vi "H2O_DIAL_NCAR_4CH_TL-15_DREW_Bristal.vi"() -> ()   [LabVIEW 2012]
uses:
  C:/Users/H2ODial/Desktop/Shared Telescope WV DIAL Code/Libraries and VIs/PowerMeterCommands.dll
  Libraries and VIs/PowerMeterCommands.dll
  <vilib>/DAQmx/write.llb/DAQmx Write (Digital 1D Bool NChan 1Samp 1Line).vi
  <vilib>/DAQmx/miscellaneous.llb/DAQmx Fill In Error Info.vi
  <vilib>/Analysis/baseanly.llb/Mean (DBL).vi
  Libraries and VIs/Scalar_Data.vi
  Libraries and VIs/Scalar_Data_3.vi
  Libraries and VIs/Scalar_Data_2.vi
  Libraries and VIs/Scalar_Data_4.vi
  <vilib>/Analysis/NI_AALBase.lvlib
  Libraries and VIs/CLDevIFace.dll
panel:
  out "FileHour":i32=23
  out "L_Count":i32=53
  out "sigma_off_total":dbl[](array[numeric])=[5.208849205039598e-25, 5.179959292841174e-25, 5.151195803046657e-25, 5.1225586514732085e-25, 5.094047747144251e-25, 5.065662992367965e-25, 5.037404282778186e-25, 5.00927150737618e-25, 4.98126454861227e-25, 4.953383282405838e-25, 4.925627578216075e-25, 4.897997299094336e-25, 4.870492301729357e-25, 4.843112436506362e-25, 4.815857547548482e-25, 4.788727472782032e-25, 4.7617220439738645e-25, 4.734841086795625e-25, 4.708084420857158e-25, 4.681451859776211e-25, 4.654943211207717e-25, 4.628558276908839e-25, 4.602296852770688e-25, 4.576158728885113e-25, 4.550143689568926e-25, 4.524251513435461e-25, 4.498481973414584e-25, 4.472834836810143e-25, 4.447309865353064e-25, 4.421906815219908e-25, 4.396625437097018e-25, 4.37146547621306e-25, 4.34642667238312e-25, 4.321508760048986e-25, 4.296711468309777e-25, 4.272034520972826e-25, 4.247477636588709e-25, 4.2230405284857445e-25, 4.1987229048037515e-25, 4.174524468541791e-25, 4.150444917575941e-25, 4.12648394471143e-25, 4.1026412377049725e-25, 4.0789164793067997e-25, 4.0553093472760867e-25, 4.03181951443899e-25, 4.008446648699997e-25, 3.9851904130758393e-25, 3.9620504657373146e-25, 3.9390264600249443e-25, 3.9161180444812275e-25, 3.8933248628938693e-25, 3.870646554304343e-25, 3.84808275304455e-25, 3.825633088767387e-25, 3.803297186471312e-25, 3.7810746665244923e-25, 3.7589651446973412e-25, 3.7369682321861625e-25, 3.715083535633669e-25, 3.693310657166629e-25, 3.6716491944131738e-25, 3.650098740528568e-25, 3.6286588842268585e-25, 3.6073292098036786e-25, 3.5861092971590296e-25, 3.5649987218229575e-25, 3.5439970549843686e-25, 3.5231038635231225e-25, 3.5023187100210476e-25, 3.481641152797277e-25, 3.461070745934916e-25, 3.440607039307999e-25, 3.420249578605639e-25, 3.3999979053628286e-25, 3.379851556985435e-25, 3.359810066782027e-25, 3.339872963989893e-25, 3.3200397738047987e-25, 3.300310017418253e-25, 3.280683212038771e-25, 3.26115887093071e-25, 3.2417365034402865e-25, 3.222415615047108e-25, 3.2031957073673925e-25, 3.1840762782254487e-25, 3.1650568216660012e-25, 3.146136828003442e-25, 3.1273157838503186e-25, 3.108593172181254e-25, 3.089968472349119e-25, 3.0714411601444525e-25, 3.053010707845716e-25, 3.0346765842511636e-25, 3.016438254736196e-25, 2.9982951813091775e-25, 2.9802468226611423e-25, 2.962292634217252e-25, 2.9444320682080165e-25, 2.9266645737124647e-25, 2.9089895967297565e-25, 2.8914065802543346e-25, 2.8739149643214034e-25, 2.8565141861062935e-25, 2.8392036799705346e-25, 2.8219828775633244e-25, 2.8048512078777227e-25, 2.78780809737001e-25, 2.7708529700069687e-25, 2.7539852473878644e-25, 2.7372043488187197e-25, 2.7205096914273037e-25, 2.703900690255505e-25, 2.6873767583778413e-25, 2.6709373069960633e-25, 2.654581745560292e-25, 2.6383094819074984e-25, 2.6221199223631447e-25, 2.606012471889248e-25, 2.589986534187844e-25, 2.574041511891159e-25, 2.5581768066557376e-25, 2.542391819344354e-25, 2.526685950182175e-25, 2.5110585988760766e-25, 2.4955091648422562e-25, 2.4800370473221455e-25, 2.4646416456015127e-25, 2.4493223591642267e-25, 2.4340785878790737e-25, 2.4189097322232995e-25, 2.4038151934512195e-25, 2.3887943737973404e-25, 2.3738466767012817e-25, 2.3589715070396223e-25, 2.3441682712794586e-25, 2.3294363777860924e-25, 2.314775236976836e-25, 2.3001842616240263e-25, 2.2856628670238404e-25, 2.2712104713105327e-25, 2.2568264956406535e-25, 2.2425103644896206e-25, 2.2282615058785225e-25, 2.214079351630966e-25, 2.199963337672995e-25, 2.185912904247297e-25, 2.171927496176536e-25, 2.1580065631915612e-25, 2.1441495601166053e-25, 2.130355947199571e-25, 2.1166251903489134e-25, 2.102956761434408e-25, 2.089350138475947e-25, 2.075804806020214e-25, 2.0623202553022427e-25, 2.0488959845615565e-25, 2.0355314992873334e-25, 2.022226312470449e-25, 2.0089799448255746e-25, 1.9957919250810776e-25, 1.982661790138582e-25, 1.9695890854004894e-25, 1.9565733648873598e-25, 1.9436141915111585e-25, 1.9307111372629915e-25, 1.91786378336177e-25, 1.9050717205270306e-25, 1.8923345490220962e-25, 1.8796518789023204e-25, 1.8670233300839603e-25, 1.8544485325389802e-25, 1.841927126361547e-25, 1.8294587618299684e-25, 1.8170430995555026e-25, 1.804679810480881e-25, 1.7923685759181059e-25, 1.7801090876455487e-25, 1.7679010477844128e-25, 1.755744168902948e-25, 1.7436381738487216e-25, 1.7315827958133316e-25, 1.7195777781516077e-25, 1.7076228743061302e-25, 1.695717847711208e-25, 1.6838624715732568e-25, 1.6720565287447544e-25, 1.6602998115080602e-25, 1.6485921213522993e-25, 1.6369332687266632e-25, 1.6253230727521978e-25, 1.6137613609636032e-25, 1.6022479689748776e-25, 1.590782740120926e-25, 1.5793655251315856e-25, 1.5679961817100763e-25, 1.5566745741448175e-25, 1.545400572901165e-25, 1.5341740540969998e-25, 1.5229948991303635e-25, 1.5118629941358614e-25, 1.5007782295195033e-25, 1.489740499358663e-25, 1.4787497009842329e-25, 1.4678057342897598e-25, 1.4569085013281887e-25, 1.446057905553199e-25, 1.4352538513748305e-25, 1.424496243524175e-25, 1.413784986430072e-25, 1.403119983632073e-25, 1.39250113710464e-25, 1.3819283467716064e-25, 1.3714015097427362e-25, 1.3609205198754617e-25, 1.3504852669717757e-25, 1.3400956363074166e-25]
  out "sigma_on_total":dbl[](array[numeric])=[1.7816460568521e-23, 1.773895265159062e-23, 1.7660996726964617e-23, 1.7582606635691275e-23, 1.7503796165295856e-23, 1.742457904707209e-23, 1.7344968950332225e-23, 1.7264979476788507e-23, 1.7184624158522698e-23, 1.7103916450731765e-23, 1.70228697290092e-23, 1.6941497285179008e-23, 1.6859812322635967e-23, 1.6777827953068067e-23, 1.6695557191750322e-23, 1.6613012955150683e-23, 1.6530208056178096e-23, 1.6447155202046477e-23, 1.6363866989483097e-23, 1.628035590346711e-23, 1.6196634312396877e-23, 1.6112714466774645e-23, 1.6028608494950746e-23, 1.594432840236233e-23, 1.585988606693132e-23, 1.5775293239155563e-23, 1.5690561537464667e-23, 1.5605702447345527e-23, 1.5520727320269274e-23, 1.5435647369440912e-23, 1.5350473670174112e-23, 1.526521715738014e-23, 1.5179888624371733e-23, 1.5094498721480932e-23, 1.5009057953909757e-23, 1.4923576681755396e-23, 1.4838065118663258e-23, 1.4752533330592848e-23, 1.4666991234694497e-23, 1.4581448599733737e-23, 1.4495915043723148e-23, 1.441040003511776e-23, 1.432491289122247e-23, 1.4239462778701797e-23, 1.4154058711623008e-23, 1.406870955384024e-23, 1.398342401692949e-23, 1.3898210660483915e-23, 1.3813077893314117e-23, 1.3728033972217122e-23, 1.3643087002505864e-23, 1.3558244939697985e-23, 1.347351558797704e-23, 1.3388906601482023e-23, 1.330442548510279e-23, 1.3220079594796904e-23, 1.3135876137976992e-23, 1.3051822174761862e-23, 1.2967924618478218e-23, 1.2884190235963751e-23, 1.2800625649506368e-23, 1.2717237336984178e-23, 1.2634031632853991e-23, 1.25510147297007e-23, 1.246819267904798e-23, 1.2385571392220061e-23, 1.2303156641504887e-23, 1.222095406160734e-23, 1.2138969151380218e-23, 1.2057207273833233e-23, 1.1975673658193516e-23, 1.1894373401234403e-23, 1.1813311468632808e-23, 1.1732492696110752e-23, 1.1651921791093205e-23, 1.1571603333900983e-23, 1.1491541779450773e-23, 1.1411741458492443e-23, 1.1332206579108972e-23, 1.1252941228701505e-23, 1.1173949374808691e-23, 1.1095234867122125e-23, 1.1016801438577447e-23, 1.0938652708072228e-23, 1.0860792179973072e-23, 1.0783223247992995e-23, 1.0705949195180339e-23, 1.0628973196199999e-23, 1.0552298318266127e-23, 1.047592752408124e-23, 1.0399863671888359e-23, 1.0324109517969625e-23, 1.0248667718463947e-23, 1.0173540830105773e-23, 1.0098731312270984e-23, 1.0024241528791567e-23, 9.950073749338678e-24, 9.876230150809686e-24, 9.802712819544858e-24, 9.729523752075448e-24, 9.656664857121758e-24, 9.584137957566187e-24, 9.511944790994246e-24, 9.44008701246367e-24, 9.368566194835521e-24, 9.297383831309462e-24, 9.226541335953e-24, 9.15604004658773e-24, 9.085881224717996e-24, 9.016066058188983e-24, 8.946595661885089e-24, 8.877471079766275e-24, 8.80869328593128e-24, 8.74026318642537e-24, 8.672181620096636e-24, 8.604449360193221e-24, 8.537067116299817e-24, 8.470035534974442e-24, 8.403355201652768e-24, 8.337026641094161e-24, 8.27105032013882e-24, 8.205426647591286e-24, 8.140155976403815e-24, 8.075238604943476e-24, 8.010674777219785e-24, 7.946464685681034e-24, 7.882608471068495e-24, 7.819106224648686e-24, 7.755957988728922e-24, 7.693163757842924e-24, 7.630723480569596e-24, 7.56863706001298e-24, 7.506904354936172e-24, 7.445525181195512e-24, 7.384499313141995e-24, 7.323826483428576e-24, 7.263506385649789e-24, 7.203538673968723e-24, 7.143922965385938e-24, 7.084658839512623e-24, 7.025745840785392e-24, 6.967183478374333e-24, 6.908971227895747e-24, 6.851108531901346e-24, 6.793594800808018e-24, 6.736429414386207e-24, 6.67961172191959e-24, 6.623141043091801e-24, 6.567016669697881e-24, 6.5112378653508866e-24, 6.455803867159162e-24, 6.400713886115458e-24, 6.345967108304617e-24, 6.2915626947315444e-24, 6.237499783446669e-24, 6.18377748907835e-24, 6.130394904244926e-24, 6.077351100139125e-24, 6.024645127233271e-24, 5.972276015715119e-24, 5.9202427766811525e-24, 5.868544402036172e-24, 5.817179866157465e-24, 5.766148125522754e-24, 5.7154481199633725e-24, 5.6650787731456875e-24, 5.6150389928060976e-24, 5.565327672180314e-24, 5.515943689491057e-24, 5.466885909347513e-24, 5.418153182700111e-24, 5.36974434796048e-24, 5.321658231169485e-24, 5.273893646284607e-24, 5.2264493962483505e-24, 5.1793242730199045e-24, 5.1325170580578076e-24, 5.086026523333733e-24, 5.0398514309077376e-24, 4.993990534244649e-24, 4.9484425777837306e-24, 4.9032062982178666e-24, 4.8582804242653355e-24, 4.813663677287351e-24, 4.7693547718840175e-24, 4.7253524158646564e-24, 4.681655310929801e-24, 4.638262152931246e-24, 4.595171632226394e-24, 4.552382434023412e-24, 4.5098932386213854e-24, 4.467702721932566e-24, 4.425809555702291e-24, 4.3842124077257986e-24, 4.3429099423396456e-24, 4.301900820527674e-24, 4.261183700301938e-24, 4.220757237070317e-24, 4.180620083546408e-24, 4.140770890465617e-24, 4.101208306569908e-24, 4.061930979032737e-24, 4.022937553353332e-24, 3.9842266741114735e-24, 3.94579698459456e-24, 3.907647127699094e-24, 3.8697757453874826e-24, 3.832181479485934e-24, 3.79486297171598e-24, 3.757818863809392e-24, 3.7210477977800845e-24, 3.684548415872136e-24, 3.648319361213695e-24, 3.612359277439583e-24, 3.576666809480403e-24, 3.54124060303094e-24, 3.506079305171125e-24]
  out "background start":u32=209
  in  "Tab Control 2":enum32{"WV ND far", "WV ND near"}(tab)
  out "Water Vapor Number Density":dbl[][](graph)=[[-3.869176758577077, 1.7276694935317216, 2.7488871422111054, 1.7014197300850586, 1.5903170185720343, 1.5423321275662938, 1.8132607286797402, 1.9740256778767107, 1.8741507349652864, 1.86470777497544, 1.8050217471405994, 1.66518518330514, 1.7222522935643614, 1.742698018284987, 1.7186667192977487, 1.76396406976016, 1.8206709341870522, 1.8804172540359552, 1.7798038295977383, 1.685641859418033, 1.7032805323016422, 1.6821483240571278, 1.7628527236349734, 1.8316160827388441, 1.7868354165982292, 1.8176435654609677, 1.8911325035020297, 1.9070639564654333, 1.6511262934763296, 1.3290513703392042, 1.261765913847659, 1.1879210634564727, 1.3181838592004227, 1.4770043973103777, 1.515246627762386, 1.4475403930811108, 1.065848464452276, 1.0853345452851404, 1.2017781570763117, 0.9102790626084151, 0.9318943803136962, 0.9732524106405078, 0.8179973089248536, 0.6079032662908113, 0.561139551967481, 0.366828467183368, 0.05249595600990845, -0.09415617998531356, -0.03868889564187686, 0.07617721364907153, 0.03962425104838462, -0.12021617725713296, 0.03637946037051569, 0.14077744142052095, 0.0245296261927154, 0.24563205234877428, 0.5539197433725966, 0.263890494465195, 0.04766355724545887, 0.09570570854419765, 0.1664575082800971, 0.06746981079040626, -0.38375673627375345, -0.3520441975802064, -0.22147709479573255, -0.2987058066521773, -0.01283079930649804, 0.27293559298756215, 0.26610575594455993, 0.00637948968643232, -0.36080028041915424, -0.7602209267225687, 0.4514801381952214, 1.1532965328629945, -0.23548265802060744, -0.25988039893494896, -0.10346486157003504, -0.9068324993519856, -1.275622846338939, -0.7873849995684254, 0.5363570467662349, 1.1750455340428092, -0.4637762421465685, -0.9826963080532389, 0.7015531311665566, 1.2530696546508981, 1.0822536008721295, 1.7170434774279757, 1.2226388206906942, -0.16161614279730033, -0.5683199941258456, -0.5177748284798833, 0.08469425738265512, -0.19130410683826007, -0.08656337463651688, -0.3423075638169604, -0.840233672330641, -0.5847959086269064, 0.3038014646272331, -0.13050495344579416, -0.1376727003604833, 3.131072497793134, 1.0729187415399541, 0.08025498921874048, -0.3838816719506945, -0.9725388459388364, -0.6672976015227235, 2.560758632555869, 2.729719175818429, 2.3215477291096027, 3.992511565505456, -3.4414781626187976, -0.46339897120913937, 5.1718139470877835, 5.339784841332441, 1.5152541194098013, 0.14047483029231167, -2.810651224807273, -2.894122973967911, -0.9646913594986185, -3.1457768234772865, 0.9532976438947683, 0.2558999676656563, -4.453408932787016, -4.666689490838906, 0.37315557538439503, 2.2772866584050298, 9.102342735433101, 14.75511277527104, 5.0407452084138225, -2.8128831706899127, 5.027850129919315, 1.8931389085909622, -2.5178123636904877, -9.123913386897096, -7.628293920055456, -7.247916135816338, -21.468900020294242, -27.22073007893985, -13.633022532482114, -6.147500862719829, -3.560625137342051, 8.50678028294044, -9.907610681399557, -0.5951038934066528, 7.40264971170572, 15.060151878437237, 11.921795085668185, 18.717702285329914, 1.661459093699086, -2.719045903890811, -1.7707613039198502, -21.905540574534093, -1.0246737433253428, 11.484928239923606, -18.946452941933938, -17.06198763650667, -8.948109634815614, -24.40872593826368, -1.1349299955140333, 17.76186196255086, 7.211953881151515, 5.768882684316489, 1.8197219317421747, -8.601060392003859, 28.569279644062227, 45.756313628626245, -3.0966253403425252, 24.64942593279667, 6.740715774414794, -13.517696399672857, -18.245119081981933, -15.538137694765226, 43.914897074779645, -11.896913533924605, -38.50542587824902, -60.431586714709645, 3.4942649258288485, -2.9978367720438235, -15.508923651730063, -32.856452935921865, 1.3021555172975168, 8.620556918106015, -36.48761227825641, 10.036727386562887, 27.44659631342583, -6.0226777499226545, 27.362796040286657, -37.45596081084036, 86.37563919610214, 63.19805672056316, 25.89420561946089, 0.556775142694816, 80.7843185510899, 4.8800300899385975, -21.298521924929055, 13.798770304785254, 41.276796377764, 25.133260462123662, -131.76792036329653, -63.33200841129719, -42.49224251142825, -17.61716602055814, -100.97764607148362, -23.093541216998897, 20.565346438983532, -21.166943213929525, -66.85855512778777, 34.9469970207709, -36.534646589901264, 127.648061869762, 113.71968873955664, 116.76977055808356, 111.55231169466157, 114.09907634429825, 88.66274623657421, 0.0, 0.0, 0.0, 0.0]]
  out "Water Vapor Number Density 2":dbl[][](graph)=[[-1.5443306097046143, 2.8522805328006084, 3.9503962044958856, 1.7990159877935195, 1.718543728389198, 1.6932470135146567, 1.7872890959132228, 1.9444655123923098, 1.9109163630014983, 1.786790355844181, 1.8203570881289517, 1.8278832324692647, 1.8215867030739905, 1.8693881519091904, 1.774018488126486, 1.7651448395397114, 2.1121219489333822, 2.2540664534955406, 2.0439110551035746, 1.9629919736185735, 1.8298595633003019, 1.7095043482327141, 1.666013989260466, 1.366285095794705, 1.4616902151466857, 2.2573272602146743, 2.697366393087735, 2.767503701368858, 2.824231151211559, 1.8391949709521593, 1.7420479845117984, 2.830301488157029, 2.1524489733156393, 2.2937880254474106, 3.9229074879334824, 3.6257729421620533, 2.4101625171808236, 2.5600619420232316, 1.2917633097948769, 1.0096849664051895, 22.61444578462568, 0.25534016546905675, -0.8899854648514799, 1.8426887683335105, -0.7431804976403255, -3.091147289752489, -3.2685662586591704, -0.6268978238054816, 9.457130422245957, 12.987376965471386, -15.76217946676521, 5.117351146699065, 9.935146112695032, 5.310666522331181, 2.8243785343871637, 2.219814346002247, -1.6824882949711026, -3.1347232460324044, 6.274677522391716, -15.294434193506227, 4.9655234368204315, -7.499211539861518, -18.986284869525754, -22.146770284669905, -15.358627756713357, -11.410536018137048, 2.694880288695569, 1.0084240385621965, -24.302059778902542, -5.424444800831853, -8.374133035691955, -3.839271193448914, -7.237647107240136, -8.381370981005263, -12.644696124542769, -14.758763725308427, -229.1767077139342, -26.690833610496536, -27.137431619530496, -35.64066674098872, -29.396651111364527, -26.79804782533207, 0.5331643103900505, 7.663673000483812, 11.575946950935077, 6.507396151064453, 209.12899102577234, 11.41629111125545, 17.293199830760145, 6.792318505705173, 32.50778308178908, 44.797851527429785, 39.153268976697944, 34.703453008989634, 30.76080492824301, 49.359391431456224, 42.446731318655694, 30.0888196357715, 8.433409642645435, 13.168323747779349, -22.073856515721904, -28.682049927165874, -44.14597625638005, -32.48394246704076, -23.003786727142135, -47.09138656023136, -47.920840441120504, -31.8982280785437, -16.04539071651972, -2.7480282517398633, 5.248156676680989, 4.922612847871278, 0.318336139544576, -0.4862458105609459, -4.179014617318633, 0.7669045218891034, 13.338663676578376, 18.57437167630363, 38.78732302419309, 26.400175395888585, 17.39277458143397, 18.272895200830188, 27.623342106489204, 20.864190489619656, 26.226824008859122, 8.996876024344196, -16.383735405016303, -23.47162210047236, -33.740458481599866, -18.105503466986512, -48.11166006948978, -42.593887413019544, -24.53098108754986, -16.94813071741411, -25.996257810862737, -0.39358969043194625, 27.123587253355726, 8.014421627535988, -6.935017542522941, 1.4770044975105434, 36.40827027087462, 36.8340413388943, 18.655014433644215, -3.3515131672034886, -21.48412539473853, -20.759894357501476, -15.862065254431439, 9.101365563103611, 20.359635034836895, 0.6709218106358483, -9.832471896842145, -16.84514663391321, -20.5476550377528, -13.656934323110177, 17.193357185961737, -3.001810086333975, -30.404097981013283, -2.8019970495102795, 11.187088633119922, 11.930034566140032, -2.3269211234070606, -17.865366856340884, -7.841326713329807, 11.502546001559406, -5.698207821198067, 8.183280425430254, 24.595245021019227, -9.239519757011584, -56.82051834132085, -25.45057389070378, 3.68551297425237, 13.924870638300932, -11.703807237602431, 1.7327637589277107, 23.617738062249668, -0.38832652817943536, -9.793160089936272, 28.29754334951125, 53.38824852184467, -9.390908410980694, -7.039011955964897, -27.352587599268645, 24.40018260217878, 23.274510436680274, -14.773755808771865, 19.203702709910885, 41.08553410088621, -25.433481617817737, -42.296254212448005, 29.341189509465494, 8.293515144836189, 12.836812085227644, 12.01172385875116, -23.51640940790944, -3.844970096464795, 24.7018027378986, -15.629344885370898, 46.841354406997496, 18.846412127663438, -8.01413384755022, 20.173550353711494, 40.332927124397294, -36.0632814643046, 42.42659273396934, 15.266963000405319, -43.789869007181714, -4.314897141425726, -71.56712981596844, -14.119956089715068, -16.016149328363884, 13.688096121679713, 15.964585047763242, 60.89547744616684, -7.0780618158529744, 21.580968070414038, 45.81592366790833, 0.0, 0.0, 0.0, 0.0]] caption="Water Vapor Number Density"
  out "RingBuffer offline near":dbl[][](array[numeric])
  out "RingBuffer aerosol near":dbl[][](array[numeric])
  in  "?":T1(tab)=enum."Raw Counts far"
  out "NRB":dbl[][](graph)=[[0.003930472506649335, 0.01856167580177092, 0.02113550600005818, 0.00020659819039981744, 0.0004794046077180199, 0.001083137552512623, 0.0021988013419836265, 0.0041092544329047785, 0.007064816134335353, 0.011356733211595298, 0.01736467597668339, 0.025026701435469114, 0.03423478045562495, 0.044428545350929015, 0.05540162610487789, 0.06689414791198389, 0.07668063258939913, 0.08177270565134998, 0.08504838543823319, 0.0941773217771789, 0.1084250899373609, 0.13043489216970022, 0.16993149950013392, 0.21569106534945648, 0.24627293298723196, 0.2621348983374077, 0.2688103499187474, 0.2614066916235843, 0.23984353258011334, 0.21654175844380677, 0.20729347010352947, 0.211907581747061, 0.21498518012682463, 0.2099940641656903, 0.20422798251892263, 0.2002067122669493, 0.1956553193564138, 0.19231512805902898, 0.18941127292353704, 0.18521706136815214, 0.18228261326514122, 0.1803780884227828, 0.17451505611111093, 0.15596012460703929, 0.12845284806608473, 0.10613962907170191, 0.08638109669200546, 0.0698685441035237, 0.0657771979941857, 0.06701804654176632, 0.06592159640438976, 0.06744466192881599, 0.07920468748072622, 0.10083415139682901, 0.13028089521913505, 0.1620054293079384, 0.18624602524852493, 0.19705712872187683, 0.18360257948359815, 0.14751724796554955, 0.1096764233903891, 0.08021880453362741, 0.061532589115181065, 0.0816391129923796, 0.1743614835528636, 0.24584930708492536, 0.1850726081138991, 0.09165193218672707, 0.05956306826808834, 0.05340250064997599, 0.04709384690987805, 0.04552738122485284, 0.10513881642759977, 0.36679509075168293, 0.6832500352597682, 0.6228452598361331, 0.2955400136740759, 0.0965288379381804, 0.04463785561721723, 0.03331459806286399, 0.0295454069625369, 0.02954898513465661, 0.03053152365445197, 0.029744787993018985, 0.028849851226770928, 0.028395038404537717, 0.02752666688359724, 0.02637978994395, 0.024532339573489555, 0.022686590876590036, 0.022164556173745933, 0.024448917357890163, 0.025449268385637276, 0.024717277849119708, 0.025034235387734093, 0.03709636240721259, 0.08373681834453293, 0.1575651146703995, 0.23175935815265392, 0.26905595638618013, 0.2660007080148815, 0.281347881372177, 0.29637751983063615, 0.2120397193829469, 0.0822185358341878, 0.02420612946619511, 0.020626164977171818, 0.02295934815454573, 0.02239546298987765, 0.020926378758381003, 0.018942726450896123, 0.02027737989045651, 0.017257308197544903, 0.01648011969227998, 0.018769849948021472, 0.01825593588795685, 0.017358907238197958, 0.018140817164234692, 0.017772892504258498, 0.017134510556994755, 0.018184511447133216, 0.015589634114438389, 0.017449874393049788, 0.021395199934042586, 0.028950512550262614, 0.04868713410644236, 0.05855925424019936, 0.056765697373354365, 0.054040949320453766, 0.03018220698627995, 0.011980903082859833, 0.013481520746379885, 0.013317721859532882, 0.012036726009435648, 0.009066141155603936, 0.010518616820675755, 0.014832016505210856, 0.014950059454567273, 0.009275637744439192, 0.009477692868505897, 0.014639857997371816, 0.015408844654833068, 0.009071008168571152, 0.006225854023779428, 0.011299265176167623, 0.012492724514216815, 0.012401612152277457, 0.010192179039525382, 0.008941655568516869, 0.00783059022139205, 0.010807654434608422, 0.014283307333364035, 0.014288825705708002, 0.010849886806011332, 0.004980035722601281, 0.005826766078719105, 0.0075934368539790275, 0.008037485025773526, 0.008886305124129305, 0.008753787211165693, 0.0056883188106616875, 0.005371602816749897, 0.008808142387202697, 0.011136376378372276, 0.004318833387582044, 0.0020970880048393737, 0.007452790671203962, 0.004158550753810091, 0.004530769527373028, 0.006894416785182974, 0.00837296741786389, 0.008085657965933137, 0.0029017041584067137, 0.006012750679637745, 0.007359146716082699, 0.008062443335548567, 0.010250086388599922, 0.004833505314473423, 0.0010466212212718276, 0.005252360150149767, 0.008100118134763674, 0.006376919009661436, 0.008745621975673537, 0.012547520645679548, 0.008878360514416051, -0.003558532177769385, -0.003931068685129671, 0.009813463187450404, 0.012245644138306774, 0.00989792059445067, 0.010224238477378817, 0.006712617893126215, -0.002666463678070868, -0.00645420474485784, -0.0031184219652592524, 0.00369116947800459, 0.0072690806727548, 0.007990187139209782, 0.008002292031103739, 0.014824575432041054, 0.014797694751457974, 0.0022899778851920263, 0.004926149957744118, 0.010253351686953951, 0.012435192336721605, 0.003082031211657591, -0.0031790134065153614, -0.0028339485571887506, -0.005707333338889842, 0.0005976659162923159, -0.000982411230437747, -0.006145669137729354, -0.00044932331870984173, 0.00428091386606607, 0.006409250601951215, 0.006428477325402283, 0.004156327474142488, 0.0, 0.0, 0.0]] caption="Water Vapor Number Density"
  out "NRB 2":dbl[][](graph)=[[0.0036371496517445994, 0.01703650318832334, 0.020633248972062875, 0.0013800426335260302, 0.003467331928749565, 0.006919838499311271, 0.011930041065111517, 0.01842671636273905, 0.025866635016207524, 0.033788053491102525, 0.042013493867585815, 0.050516184965233954, 0.059459761392953926, 0.06841915921353516, 0.07661801215634156, 0.08328622123228714, 0.08582003015959876, 0.08226852580228898, 0.0758652361797178, 0.07335427213452467, 0.07399510467073478, 0.077832413415831, 0.09074755980363364, 0.10683744208633218, 0.11379427967792226, 0.11383489707097101, 0.11213088885610459, 0.10518492418354901, 0.0920399200182776, 0.07952493986949206, 0.07523446587339368, 0.07580443903113321, 0.07507434026665262, 0.07232025663049929, 0.07040748731651326, 0.06828916338398419, 0.06567080469336894, 0.06469037970451262, 0.0644425414544769, 0.06318734377370618, 0.06063209355900223, 0.059469665719634884, 0.05748777770520413, 0.04991857127969182, 0.04039318864390559, 0.03185073389094848, 0.024176677628144835, 0.018496094801403275, 0.01776963165623099, 0.01850891772014958, 0.018428861164685752, 0.019807659791999492, 0.024041941128934815, 0.029719396461916653, 0.038809029282185416, 0.05020034200015739, 0.05660877189095595, 0.06076443427680532, 0.05511663020936872, 0.043988455546614416, 0.03331345532712681, 0.02185250713851732, 0.01577029946685516, 0.022446119886150258, 0.05594357391945572, 0.0828190885036247, 0.06050139637782499, 0.02527859256760107, 0.011594307499489899, 0.008638484256569148, 0.008864910520450759, 0.009348729824449415, 0.029540262433234078, 0.12532949022668763, 0.24340139949844283, 0.22138119398182685, 0.10007438941564159, 0.032019365617949685, 0.012390245530805056, 0.004528276018205554, 0.003275796002140223, 0.004952505987005521, 0.0069991223807995846, 0.0018426755657387614, 0.0013916137984439276, 0.003536719849559254, 0.004936369466053812, 0.00805833393141099, 0.003530237474819559, -4.1280975248141e-05, -0.0031128209847992912, -0.0019544928287063244, 0.003915493745935216, 0.001173942428925932, -0.006350329178034576, 0.0006899543668811116, 0.031108497607104286, 0.06399430457460561, 0.09217643099719275, 0.10360682795834994, 0.0988357573984754, 0.10485562014796758, 0.10315263871478404, 0.06938872580477172, 0.018961832555909063, -0.0035917489198442724, -0.002744383733131294, 0.0021338721511815306, 0.01415905229358902, 0.010655942951313698, 0.002254067110314441, 0.007354262975912472, 0.0036375737229856144, 0.0005047422524058872, 0.0035815414407817767, -0.0005178767966525964, -0.009391539564641088, -0.00946712496314058, 0.005303356363483911, 0.0020270499020427057, -0.0035738458960578264, -0.001396774601107916, -0.007521451653945964, -0.00930600236629641, 0.001883706461300565, 0.018403847478748257, 0.021007462570787113, 0.019640636355698602, 0.026383250232868284, 0.006611280584980362, -0.012798886930294198, 0.0024680408939121525, 0.008116803607827227, 0.0011549383540302525, -0.007827595884048846, -0.00495364879429496, 0.01939889749061799, 0.022444448653450716, 0.0021764895193934737, -0.0030793419371683266, 0.00866841075399524, -0.0005811484210449667, -0.01605964672983413, -0.008942504556462935, 0.005416782653565494, 0.001595818932773196, -0.00407852130382172, -0.0058663885807870245, -0.012305286929516712, -0.005294513758219532, 0.009801323745479663, 0.008449529836930333, -0.0026493162817863725, -0.008873147676594886, -0.011268625608977586, -0.002027183814169297, -0.0025514075997150856, 0.0025708727112535097, 0.021153088711398944, 0.013568986385791905, -0.017031895122065075, 0.004432240632801877, 0.0032964694542234113, -0.00902308178105749, 0.0019664276294757313, -0.017791447391965472, -0.0105814723327946, 0.02086255624836402, 0.015289014861491292, -0.011879223092562698, -0.013072802023074051, -0.008053240428419393, 0.0035555595583932225, 0.011444910625672548, 0.025812896369300224, 0.024584415737324762, -0.0014810339765029656, -0.0013586140933279985, -0.0012331517866784963, -0.0022149323139001313, 0.01002370286931542, 0.00163575012314951, -0.004525777742427229, -0.017129143916830177, -0.004835752924455243, 0.01709079326051516, 0.014110065578375252, -0.003813723821663823, 0.0024231432824741634, 0.004732768871162198, 0.008725613632898954, 0.04681544982055149, 0.05126517573045018, 0.008208163504057038, 0.004818076358944868, 0.044330213093104746, 0.019581290580246866, -0.0010954537471730096, 0.05196173543341118, 0.07206495557244628, 0.05212384819727444, 0.05282307279007492, 0.060119382877862344, 0.04502404489351928, 0.02899591798938946, 0.04870805826786507, 0.049069136303961605, 0.05346037076736777, 0.014785011813988698, -0.010377246966110278, 0.0077928132458859115, -0.024042200815203283, -0.03718525117731811, -0.03439665496604084, -0.00445979226507979, 0.0441218508899156, 0.029220984290769872, 0.0, 0.0, 0.0]] caption="Water Vapor Number Density"
  out "raw counts":dbl[][](graph)=[[17706.9, 19006.9, 23324.9, 69.9, 98.9, 165.9, 240.9, 316.9, 472.9, 547.9, 776.9, 879.9, 1050.9, 1300.9, 1491.9, 1492.9, 1595.9, 1497.9, 1327.9, 1459.9, 1423.9, 1517.9, 1909.9, 2153.9, 2285.9, 2360.9, 2225.9, 1991.9, 1677.9, 1479.9, 1256.9, 1211.9, 1215.9, 1123.9, 978.9, 900.9, 804.9, 743.9, 716.9, 664.9, 669.9, 611.9, 598.9, 582.9, 408.9, 338.9, 274.9, 233.9, 150.9, 166.9, 160.9, 130.9, 174.9, 184.9, 216.9, 306.9, 304.9, 351.9, 314.9, 279.9, 202.9, 144.9, 94.9, 95.9, 154.9, 355.9, 376.9, 159.9, 69.9, 60.900000000000006, 58.900000000000006, 19.900000000000006, 40.900000000000006, 137.9, 568.9, 827.9, 528.9, 140.9, 38.900000000000006, 20.900000000000006, 31.900000000000006, 43.900000000000006, 38.900000000000006, 28.900000000000006, 39.900000000000006, 26.900000000000006, 6.900000000000006, 13.900000000000006, 29.900000000000006, 20.900000000000006, 14.900000000000006, 2.9000000000000057, 5.900000000000006, 30.900000000000006, 7.900000000000006, 17.900000000000006, 18.900000000000006, 97.9, 97.9, 139.9, 147.9, 122.9, 137.9, 176.9, 65.9, 27.900000000000006, 13.900000000000006, 48.900000000000006, 14.900000000000006, 14.900000000000006, 12.900000000000006, 12.900000000000006, 2.9000000000000057, 1.9000000000000057, -8.099999999999994, 15.900000000000006, 22.900000000000006, 30.900000000000006, 1.9000000000000057, 19.900000000000006, 12.900000000000006, -6.099999999999994, 21.900000000000006, 0.9000000000000057, 3.9000000000000057, -1.0999999999999943, -10.099999999999994, -8.099999999999994, -9.099999999999994, 13.900000000000006, 4.900000000000006, 8.900000000000006, -8.099999999999994, 9.900000000000006, 2.9000000000000057, 16.900000000000006, 2.9000000000000057, -11.099999999999994, 8.900000000000006, -2.0999999999999943, 7.900000000000006, -4.099999999999994, 3.9000000000000057, 4.900000000000006, 35.900000000000006, -1.0999999999999943, -2.0999999999999943, -6.099999999999994, 0.9000000000000057, 1.9000000000000057, 17.900000000000006, 20.900000000000006, -13.099999999999994, 18.900000000000006, 19.900000000000006, -8.099999999999994, -5.099999999999994, 7.900000000000006, -9.099999999999994, -1.0999999999999943, -2.0999999999999943, 8.900000000000006, -5.099999999999994, 0.9000000000000057, 16.900000000000006, 21.900000000000006, 5.900000000000006, -2.0999999999999943, 2.9000000000000057, 18.900000000000006, 23.900000000000006, 17.900000000000006, 14.900000000000006, 20.900000000000006, 25.900000000000006, 2.9000000000000057, -0.09999999999999432, -18.099999999999994, -2.0999999999999943, 14.900000000000006, 13.900000000000006, -0.09999999999999432, 3.9000000000000057, 0.9000000000000057, 1.9000000000000057, 6.900000000000006, 0.9000000000000057, 18.900000000000006, -1.0999999999999943, 6.900000000000006, 16.900000000000006, 15.900000000000006, 6.900000000000006, -0.09999999999999432, 10.900000000000006, 7.900000000000006, 14.900000000000006, -5.099999999999994, 7.900000000000006, 19.900000000000006, -2.0999999999999943, -19.099999999999994, 0.9000000000000057, 13.900000000000006, 15.900000000000006, 0.9000000000000057, 9.900000000000006, 5.900000000000006, 1.9000000000000057, -21.099999999999994, 8.900000000000006, 14.900000000000006, 11.900000000000006, -6.099999999999994, -0.09999999999999432, 3.9000000000000057, -3.0999999999999943, 3.9000000000000057, -13.099999999999994, 0.0]] caption="Water Vapor Number Density"
  out "raw counts near":dbl[][](graph)=[[17211.1, 16611.1, 22030.1, 377.0999999999999, 727.0999999999999, 995.0999999999999, 1357.1, 1605.1, 1926.1, 2118.1, 2152.1, 2227.1, 2148.1, 2287.1, 2231.1, 2087.1, 1963.1, 1592.1, 1278.1, 1052.1, 993.0999999999999, 1004.0999999999999, 1061.1, 1146.1, 1093.1, 1108.1, 853.0999999999999, 775.0999999999999, 722.0999999999999, 438.0999999999999, 446.0999999999999, 445.0999999999999, 353.0999999999999, 325.0999999999999, 387.0999999999999, 318.0999999999999, 288.0999999999999, 277.0999999999999, 199.0999999999999, 247.0999999999999, 178.0999999999999, 190.0999999999999, 166.0999999999999, 168.0999999999999, 117.09999999999991, 30.09999999999991, -25.90000000000009, 79.09999999999991, 60.09999999999991, 41.09999999999991, 66.09999999999991, 11.099999999999909, 42.09999999999991, 69.09999999999991, 59.09999999999991, 93.09999999999991, 100.09999999999991, 82.09999999999991, 123.09999999999991, 100.09999999999991, 17.09999999999991, -1.900000000000091, 34.09999999999991, -23.90000000000009, 72.09999999999991, 135.0999999999999, 139.0999999999999, 82.09999999999991, 40.09999999999991, 23.09999999999991, -44.90000000000009, -77.90000000000009, -36.90000000000009, 96.09999999999991, 154.0999999999999, 269.0999999999999, 200.0999999999999, 26.09999999999991, 28.09999999999991, -4.900000000000091, -45.90000000000009, -34.90000000000009, 21.09999999999991, -20.90000000000009, 35.09999999999991, 21.09999999999991, -29.90000000000009, -8.900000000000091, -6.900000000000091, -30.90000000000009, -53.90000000000009, 7.099999999999909, 20.09999999999991, 56.09999999999991, -11.900000000000091, -81.90000000000009, -27.90000000000009, 48.09999999999991, 78.09999999999991, 123.09999999999991, 31.09999999999991, 27.09999999999991, 28.09999999999991, 32.09999999999991, -37.90000000000009, 5.099999999999909, -56.90000000000009, 29.09999999999991, -1.900000000000091, -6.900000000000091, 46.09999999999991, 83.09999999999991, -49.90000000000009, -64.90000000000009, -2.900000000000091, 105.09999999999991, -98.90000000000009, -98.90000000000009, -59.90000000000009, -45.90000000000009, 6.099999999999909, -12.900000000000091, 3.099999999999909, -11.900000000000091, -33.90000000000009, -46.90000000000009, -68.90000000000009, 72.09999999999991, -32.90000000000009, 17.09999999999991, -55.90000000000009, -0.900000000000091, -3.900000000000091, -7.900000000000091, 11.099999999999909, -26.90000000000009, -5.900000000000091, -36.90000000000009, -54.90000000000009, 50.09999999999991, 55.09999999999991, 17.09999999999991, 5.099999999999909, -18.90000000000009, 43.09999999999991, -6.900000000000091, 54.09999999999991, -15.900000000000091, 38.09999999999991, -8.900000000000091, 55.09999999999991, 13.099999999999909, -4.900000000000091, 23.09999999999991, 9.099999999999909, 2.099999999999909, 16.09999999999991, 17.09999999999991, -8.900000000000091, 32.09999999999991, -114.90000000000009, 46.09999999999991, -45.90000000000009, -36.90000000000009, 1.099999999999909, -52.90000000000009, -59.90000000000009, -29.90000000000009, 57.09999999999991, -33.90000000000009, 17.09999999999991, -25.90000000000009, -30.90000000000009, 36.09999999999991, -16.90000000000009, -20.90000000000009, 37.09999999999991, -50.90000000000009, -37.90000000000009, 26.09999999999991, 53.09999999999991, 39.09999999999991, -15.900000000000091, -8.900000000000091, -26.90000000000009, -15.900000000000091, -84.90000000000009, 76.09999999999991, 2.099999999999909, -26.90000000000009, -39.90000000000009, 32.09999999999991, 31.09999999999991, 9.099999999999909, 76.09999999999991, 2.099999999999909, -32.90000000000009, 2.099999999999909, -50.90000000000009, -6.900000000000091, 52.09999999999991, -39.90000000000009, -0.900000000000091, -28.90000000000009, -10.900000000000091, -0.900000000000091, 16.09999999999991, -4.900000000000091, 43.09999999999991, 14.099999999999909, 4.099999999999909, 22.09999999999991, -57.90000000000009, -5.900000000000091, 6.099999999999909, -9.900000000000091, -14.900000000000091, 35.09999999999991, 7.099999999999909, 0.0]] caption="Water Vapor Number Density"
  out "Aerosol Smoothed 2":dbl[](array[numeric])=[16757.787962962968, 19211.093518518515, 11076.852777777774, 452.90370370370385, 726.7648148148149, 1005.1259259259261, 1270.5796296296294, 1499.9268518518513, 1661.593518518518, 1756.7879629629624, 1804.6861111111104, 1823.079629629629, 1828.338888888888, 1814.2138888888883, 1770.3527777777772, 1692.3944444444442, 1546.4638888888883, 1324.547222222222, 1098.139814814815, 959.2740740740744, 878.2277777777779, 841.9314814814816, 897.7555555555557, 970.1583333333336, 952.4453703703707, 881.3759259259261, 805.5240740740742, 703.1583333333335, 574.139814814815, 463.93611111111125, 411.2092592592594, 388.8990740740742, 362.2370370370371, 328.80648148148157, 302.1398148148148, 277.0472222222221, 252.2648148148147, 235.6212962962962, 222.85740740740732, 207.75092592592586, 189.7694444444444, 177.3898148148147, 163.61203703703697, 135.71388888888885, 105.01481481481478, 79.26018518518518, 57.63981481481483, 42.283333333333346, 38.98240740740741, 38.99629629629629, 37.32037037037037, 38.58425925925927, 45.079629629629636, 53.67685185185185, 67.56111111111109, 84.28796296296292, 91.73703703703701, 95.10277777777776, 83.3712962962963, 64.34814814814817, 47.15370370370371, 29.945370370370377, 20.931481481481484, 28.86666666666667, 69.72777777777777, 100.09814814814814, 70.97314814814814, 28.797222222222228, 12.829629629629629, 9.287962962962961, 9.264814814814814, 9.500925925925925, 29.200000000000003, 120.47777777777775, 227.59814814814808, 201.63518518518512, 88.87129629629626, 27.723148148148148, 10.459259259259259, 3.727777777777777, 2.6305555555555546, 3.880555555555555, 5.352777777777777, 1.3759259259259249, 1.014814814814814, 2.5194444444444435, 3.4361111111111104, 5.482407407407407, 2.348148148148147, -0.02685185185185268, -1.9805555555555565, -1.2166666666666677, 2.3851851851851844, 0.6999999999999992, -3.707407407407408, 0.3944444444444435, 17.417592592592598, 35.098148148148155, 49.533333333333346, 54.56574074074075, 51.02870370370371, 53.079629629629636, 51.20925925925926, 33.7925925925926, 9.061111111111117, -1.6842592592592602, -1.262962962962964, 0.9638888888888879, 6.278703703703703, 4.639814814814814, 0.963888888888888, 3.088888888888888, 1.500925925925925, 0.20462962962962883, 1.426851851851851, -0.20277777777777864, -3.6148148148148156, -3.582407407407408, 1.9731481481481474, 0.7416666666666658, -1.286111111111112, -0.4944444444444453, -2.6194444444444454, -3.1888888888888896, 0.6351851851851844, 6.107407407407407, 6.8620370370370365, 6.31574074074074, 8.352777777777778, 2.0611111111111104, -3.9296296296296305, 0.7462962962962953, 2.417592592592592, 0.338888888888888, -2.262962962962964, -1.411111111111112, 5.4453703703703695, 6.209259259259259, 0.5935185185185177, -0.8277777777777786, 2.2972222222222216, -0.1518518518518528, -4.137962962962964, -2.272222222222223, 1.3574074074074065, 0.3944444444444435, -0.9944444444444454, -1.411111111111112, -2.9203703703703714, -1.2398148148148158, 2.264814814814814, 1.9268518518518511, -0.5962962962962971, -1.971296296296297, -2.471296296296297, -0.43888888888888977, -0.5453703703703712, 0.5425925925925917, 4.408333333333332, 2.792592592592592, -3.462037037037038, 0.8898148148148142, 0.653703703703703, -1.7675925925925935, 0.38055555555555465, -3.401851851851853, -1.999074074074075, 3.8944444444444435, 2.8203703703703695, -2.1657407407407416, -2.355555555555556, -1.43425925925926, 0.6259259259259251, 1.9916666666666658, 4.44074074074074, 4.18148148148148, -0.24907407407407478, -0.22592592592592675, -0.2027777777777786, -0.36018518518518594, 1.612037037037036, 0.2601851851851843, -0.7120370370370379, -2.6657407407407416, -0.7444444444444451, 2.602777777777777, 2.125925925925925, -0.5685185185185193, 0.35740740740740673, 0.69074074074074, 1.2601851851851842, 6.69074074074074, 7.250925925925925, 1.1490740740740732, 0.6675925925925918, 6.079629629629629, 2.6583333333333323, -0.1472222222222231, 6.912962962962962, 9.491666666666665, 6.797222222222222, 6.8203703703703695, 7.68611111111111, 5.699999999999999, 3.6351851851851844, 6.047222222222221, 6.033333333333332, 6.510185185185184, 1.7833333333333328, -1.2398148148148156, 0.9222222222222214, -2.8185185185185198, -4.31851851851852, -3.957407407407408, -0.5083333333333344, 4.982407407407407, 3.2694444444444435]
  out "Off-Line Smoothed 2":dbl[](array[numeric])=[16312.774744027298, 18964.783276450507, 11043.148464163822, 438.67406143344704, 710.3941979522183, 979.965870307167, 1236.8976109215014, 1450.4846416382252, 1602.967576791809, 1704.5665529010244, 1760.9351535836186, 1781.5341296928336, 1782.6655290102399, 1768.8259385665538, 1735.8720136518778, 1662.2098976109219, 1505.2764505119455, 1299.324232081911, 1129.5051194539246, 1013.9402730375423, 918.7918088737199, 841.8293515358359, 836.4880546075083, 908.7235494880545, 949.8771331058019, 913.1774744027302, 844.2662116040954, 765.8276450511944, 670.1672354948803, 555.3088737201363, 456.5955631399315, 389.5102389078497, 350.48976109215016, 322.43174061433456, 291.2815699658704, 265.90443686006836, 246.4146757679182, 230.16894197952226, 215.2440273037543, 199.32764505119462, 184.04778156996593, 171.46757679180894, 155.95733788395916, 129.65187713310587, 101.11262798634816, 78.63993174061433, 57.863481228668924, 40.47440273037542, 34.24914675767918, 33.046075085324226, 33.74914675767918, 33.35324232081912, 32.21672354948806, 37.479522184300336, 48.97269624573378, 62.35494880546074, 74.09385665529007, 86.12969283276449, 86.95392491467578, 70.26109215017064, 47.21672354948804, 29.581911262798624, 20.203071672354945, 20.21672354948805, 46.61092150170647, 82.56143344709898, 74.0085324232082, 33.064846416382245, 8.481228668941982, 4.665529010238913, 6.709897610921507, 8.25767918088738, 36.76109215017063, 139.70819112627987, 225.44880546075092, 168.0034129692833, 62.9112627986348, 16.11945392491468, 3.7252559726962513, 1.2593856655290157, 0.9266211604095618, -1.063139931740609, 5.329070518200751e-15, -0.6433447098976055, -0.5767918088737147, 0.1723549488054661, -0.8395904436860014, -0.24744027303753724, -2.2781569965870254, -3.3105802047781516, -4.4266211604095504, -1.7133105802047726, 0.8737201365187768, -2.7713310580204724, -5.916382252559721, -0.1365187713310525, 16.27986348122867, 32.339590443686, 43.631399317406135, 47.964163822525585, 47.119453924914666, 50.873720136518756, 51.93003412969283, 37.93174061433447, 12.25938566552901, -2.9539249146757625, -4.286689419795216, -4.633105802047776, -2.032423208191121, -3.7354948805460673, -5.813993174061426, -1.9522184300341243, -0.912969283276445, -2.626279863481223, -1.433447098976104, -1.4965870307167182, -5.969283276450507, -4.76450511945392, -1.291808873720131, -3.7064846416382196, -5.817406143344704, -3.0938566552900966, 4.237201365187719, 16.36689419795222, 44.715017064846435, 124.27474402730378, 246.259385665529, 307.30716723549483, 256.40955631399316, 144.56825938566558, 46.720136518771355, 6.206484641638233, -0.587030716723544, -1.003412969283271, -2.406143344709892, -3.3088737201365133, -0.22866894197951682, 0.5477815699658757, -2.5187713310580153, -4.4317406143344655, -3.3412969283276395, -3.9095563139931686, -7.320819112627984, -5.600682593856652, -2.8191126279863425, -3.9761092150170594, -2.6843003412969226, -3.162116040955626, -4.218430034129687, -1.6058020477815644, -0.7576791808873666, -1.0273037542662062, -2.4914675767918033, -5.617747440273032, -5.9453924914675715, -2.660409556313988, -3.1211604095563086, -2.9709897610921447, 0.9880546075085378, 0.8156996587030771, -1.7218430034129637, -0.4522184300341242, -0.21160409556313453, -3.564846416382247, -3.5887372013651824, -2.14846416382252, -1.8566552901023838, 0.4846416382252613, -0.6706484641638173, -2.7730375426621108, -1.3532423208191071, -1.6211604095563086, -2.2201365187713256, -1.9095563139931686, -0.16382252559726418, 0.8703071672355003, 1.8464163822525652, 1.8174061433447153, -0.6433447098976055, -2.6587030716723494, -3.1365187713310525, -1.6075085324232028, 0.5819112627986402, -1.1484641638225201, -2.1348122866894146, 0.3703071672355003, 2.0068259385665583, 0.35494880546075636, -0.5716723549488, -0.7883959044368546, 1.2559726962457392, 5.576791808873725, 3.626279863481234, -1.3003412969283223, 0.4300341296928383, 4.13993174061434, 1.331058020477821, 0.34300341296928866, 3.694539249146763, 2.2116040955631453, 1.0614334470989815, 2.549488054607514, 1.3634812286689475, 1.0051194539249202, 1.0392491467576845, -0.7679180887371959, -1.4146757679180832, 0.5273037542662171, -0.24914675767917538, -0.8447098976109161, 1.800341296928333, 0.4351535836177529, -0.7081911262798579, 0.2303754266211659, 0.29351535836178017, -1.006825938566548, -0.7559726962457288]
  out "Off-Line Bin Readings 2":dbl[](array[numeric])=[18847.0, 18247.0, 23666.0, 2013.0, 2363.0, 2631.0, 2993.0, 3241.0, 3562.0, 3754.0, 3788.0, 3863.0, 3784.0, 3923.0, 3867.0, 3723.0, 3599.0, 3228.0, 2914.0, 2688.0, 2629.0, 2640.0, 2697.0, 2782.0, 2729.0, 2744.0, 2489.0, 2411.0, 2358.0, 2074.0, 2082.0, 2081.0, 1989.0, 1961.0, 2023.0, 1954.0, 1924.0, 1913.0, 1835.0, 1883.0, 1814.0, 1826.0, 1802.0, 1804.0, 1753.0, 1666.0, 1610.0, 1715.0, 1696.0, 1677.0, 1702.0, 1647.0, 1678.0, 1705.0, 1695.0, 1729.0, 1736.0, 1718.0, 1759.0, 1736.0, 1653.0, 1634.0, 1670.0, 1612.0, 1708.0, 1771.0, 1775.0, 1718.0, 1676.0, 1659.0, 1591.0, 1558.0, 1599.0, 1732.0, 1790.0, 1905.0, 1836.0, 1662.0, 1664.0, 1631.0, 1590.0, 1601.0, 1657.0, 1615.0, 1671.0, 1657.0, 1606.0, 1627.0, 1629.0, 1605.0, 1582.0, 1643.0, 1656.0, 1692.0, 1624.0, 1554.0, 1608.0, 1684.0, 1714.0, 1759.0, 1667.0, 1663.0, 1664.0, 1668.0, 1598.0, 1641.0, 1579.0, 1665.0, 1634.0, 1629.0, 1682.0, 1719.0, 1586.0, 1571.0, 1633.0, 1741.0, 1537.0, 1537.0, 1576.0, 1590.0, 1642.0, 1623.0, 1639.0, 1624.0, 1602.0, 1589.0, 1567.0, 1708.0, 1603.0, 1653.0, 1580.0, 1635.0, 1632.0, 1628.0, 1647.0, 1609.0, 1630.0, 1599.0, 1581.0, 1686.0, 1691.0, 1653.0, 1641.0, 1617.0, 1679.0, 1629.0, 1690.0, 1620.0, 1674.0, 1627.0, 1691.0, 1649.0, 1631.0, 1659.0, 1645.0, 1638.0, 1652.0, 1653.0, 1627.0, 1668.0, 1521.0, 1682.0, 1590.0, 1599.0, 1637.0, 1583.0, 1576.0, 1606.0, 1693.0, 1602.0, 1653.0, 1610.0, 1605.0, 1672.0, 1619.0, 1615.0, 1673.0, 1585.0, 1598.0, 1662.0, 1689.0, 1675.0, 1620.0, 1627.0, 1609.0, 1620.0, 1551.0, 1712.0, 1638.0, 1609.0, 1596.0, 1668.0, 1667.0, 1645.0, 1712.0, 1638.0, 1603.0, 1638.0, 1585.0, 1629.0, 1688.0, 1596.0, 1635.0, 1607.0, 1625.0, 1635.0, 1652.0, 1631.0, 1679.0, 1650.0, 1640.0, 1658.0, 1578.0, 1630.0, 1642.0, 1626.0, 1621.0, 1671.0, 1643.0]
  out "On-Line Smoothed 2":dbl[](array[numeric])=[15541.432423208193, 19397.596245733785, 11398.275426621158, 387.4733788395904, 598.5331058020479, 789.562116040956, 954.8931740614335, 1072.6320819112625, 1130.8965870307165, 1143.3607508532423, 1129.2464163822524, 1093.4255972696246, 1044.734470989761, 992.1832764505118, 930.4477815699661, 851.1491467576795, 740.2890784982937, 610.9836177474406, 501.90170648464175, 428.08088737201376, 370.4477815699659, 323.89317406143346, 309.4238907849829, 322.73447098976106, 325.12696245733787, 304.4119453924915, 270.1610921501707, 230.20716723549486, 189.63037542662107, 147.23788395904432, 113.7447098976109, 95.0877133105802, 80.79249146757678, 69.42730375426618, 61.055290102389066, 51.78225255972696, 43.53139931740615, 38.297610921501715, 34.2703071672355, 29.720819112627986, 27.72764505119454, 24.500682593856652, 19.200341296928322, 11.311262798634804, 3.4324232081911195, 2.7737201365187647, 0.09624573378838841, -6.053924914675779, -6.197269624573389, -3.2433447098976176, -5.610238907849838, -8.412286689419805, -7.315017064846424, -3.6648464163822596, -0.275767918088744, -0.18361774744027987, 3.142320819112621, 4.597952218430027, 2.2208191126279795, -2.420819112627992, -4.253583617747446, -4.410580204778165, -5.623890784982942, -3.33720136518772, -0.09488054607509211, 4.601365187713302, 1.2976109215016982, -6.71262798634813, -6.671672354948813, -8.492491467576798, -9.113651877133112, -9.024914675767926, -6.256996587030725, 19.500682593856652, 39.07747440273038, 26.06552901023891, 5.447781569965863, -6.434470989761099, -9.26211604095564, -8.274061433447107, -9.315017064846426, -12.308191126279873, -12.00955631399318, -9.47542662116042, -11.161433447098986, -11.538566552901035, -12.251877133105811, -9.995904436860073, -7.3645051194539315, -8.844027303754274, -9.67508532423209, -9.197269624573385, -5.50102389078499, -7.209215017064855, -8.30989761092151, -2.844027303754273, -1.934470989761099, -1.669965870307174, -0.4856655290102457, 0.8436860068259319, 1.202047781569959, 0.2191126279863413, 0.6798634812286621, -1.2092150170648532, -4.316723549488061, -6.651194539249154, -9.422525597269633, -11.417406143344717, -9.47201365187714, -5.697269624573385, -3.610238907849836, -5.359385665529017, -7.808191126279871, -6.5761092150170715, -4.420819112627994, -4.804778156996594, -6.893515358361782, -6.367918088737208, -5.485665529010245, -6.18361774744028, -6.617064846416389, -7.668259385665536, -6.700682593856662, -4.480546075085331, 1.3846416382252498, 16.886348122866902, 36.84027303754268, 47.56552901023892, 39.86416382252561, 20.33174061433448, 2.534812286689415, -4.661433447098982, -4.7433447098976185, -3.487372013651884, -3.4071672354948874, -3.4225255972696313, -6.282593856655297, -8.678498293515366, -6.05904436860069, -4.427645051194546, -3.5232081911262867, -3.398634812286696, -3.502730375426628, -8.379863481228677, -8.166552901023898, -3.7655290102389145, -1.7040955631399384, -1.1614334470989829, -1.5726962457337952, -2.1733788395904505, -5.97372013651878, -6.33890784982936, -5.639249146757686, -3.639249146757686, -2.5283276450512013, -2.4071672354948874, -5.018088737201372, -5.393515358361782, -2.5197952218430104, -3.7160409556314065, -2.729692832764512, -3.2399317406143413, -6.221160409556321, -3.2518771331058085, 0.6918088737201298, -0.7774744027303822, -3.664846416382259, -3.7843003412969347, -3.1853242320819177, -4.774061433447105, -3.463481228668949, -5.545392491467584, -7.705802047781577, -3.758703071672362, -2.9481228668942046, -2.5931740614334537, -2.9156996587030783, -4.709215017064853, -6.985665529010246, -4.289419795221851, -1.4941979522184368, -5.567576791808882, -3.9805460750853325, -0.3218430034129761, -0.7843003412969352, -2.0078498293515428, -5.193856655290109, -5.709215017064853, -1.0539249146757748, -0.2757679180887441, 1.770307167235488, 5.2208191126279795, 1.5348122866894132, -2.1187713310580274, -2.610238907849836, -3.2416382252559792, -1.9686006825938636, -2.01979522184301, -3.192150170648471, -3.6068259385665598, -1.8935153583617814, -0.5778156996587099, -1.6017064846416451, 0.10648464163821836, 1.8197952218429965, 0.9682593856655222, 0.6474402730375359, -0.27406143344710565, -1.555631399317413, -0.12730375426621848, -1.2843003412969352, -1.1409556313993243, 1.0109215017064779, -1.282593856655297, 1.0382252559726892, 2.917064846416375, 0.19180887372012967]
  out "On-Line Bin Readings 2":dbl[](array[numeric])=[17690.0, 19080.0, 24921.0, 1970.0, 2377.0, 2636.0, 2978.0, 3075.0, 3208.0, 3294.0, 3254.0, 3210.0, 3136.0, 3089.0, 2993.0, 2779.0, 2704.0, 2538.0, 2330.0, 2319.0, 2124.0, 2097.0, 2104.0, 1996.0, 2078.0, 2019.0, 2024.0, 1923.0, 1881.0, 1791.0, 1803.0, 1761.0, 1814.0, 1758.0, 1741.0, 1734.0, 1841.0, 1709.0, 1734.0, 1717.0, 1705.0, 1682.0, 1694.0, 1804.0, 1662.0, 1689.0, 1651.0, 1669.0, 1645.0, 1596.0, 1608.0, 1526.0, 1655.0, 1621.0, 1668.0, 1741.0, 1594.0, 1718.0, 1623.0, 1704.0, 1664.0, 1722.0, 1646.0, 1654.0, 1667.0, 1692.0, 1721.0, 1700.0, 1615.0, 1607.0, 1615.0, 1574.0, 1708.0, 1650.0, 1725.0, 1686.0, 1705.0, 1623.0, 1662.0, 1621.0, 1654.0, 1611.0, 1609.0, 1603.0, 1668.0, 1686.0, 1573.0, 1553.0, 1635.0, 1661.0, 1661.0, 1681.0, 1635.0, 1636.0, 1667.0, 1623.0, 1677.0, 1630.0, 1682.0, 1609.0, 1655.0, 1652.0, 1573.0, 1686.0, 1566.0, 1631.0, 1644.0, 1640.0, 1701.0, 1657.0, 1651.0, 1630.0, 1602.0, 1689.0, 1600.0, 1614.0, 1616.0, 1628.0, 1700.0, 1663.0, 1627.0, 1606.0, 1650.0, 1617.0, 1683.0, 1696.0, 1662.0, 1676.0, 1571.0, 1653.0, 1643.0, 1715.0, 1591.0, 1678.0, 1613.0, 1653.0, 1617.0, 1634.0, 1513.0, 1639.0, 1602.0, 1677.0, 1749.0, 1618.0, 1585.0, 1659.0, 1600.0, 1688.0, 1655.0, 1668.0, 1623.0, 1581.0, 1618.0, 1615.0, 1632.0, 1615.0, 1653.0, 1596.0, 1587.0, 1613.0, 1645.0, 1633.0, 1624.0, 1611.0, 1567.0, 1608.0, 1682.0, 1625.0, 1579.0, 1575.0, 1604.0, 1591.0, 1649.0, 1660.0, 1596.0, 1576.0, 1686.0, 1694.0, 1689.0, 1676.0, 1706.0, 1728.0, 1602.0, 1637.0, 1661.0, 1694.0, 1595.0, 1624.0, 1690.0, 1623.0, 1598.0, 1522.0, 1655.0, 1572.0, 1638.0, 1659.0, 1615.0, 1621.0, 1715.0, 1611.0, 1666.0, 1682.0, 1651.0, 1701.0, 1601.0, 1653.0, 1602.0, 1695.0, 1680.0, 1673.0, 1701.0, 1623.0, 1697.0, 1652.0, 1600.0, 1639.0, 1636.0, 1568.0, 1698.0]
  in  "stop":bool
  in  "Reset Average":bool=TRUE
  in  "Save Data?":bool=TRUE
  in  "Collect Data?":bool=TRUE
  in  "ILX Address":i32=6 min=0 step=1
  in  "Lambda On DBR Current":dbl=158.08
  in  "Lambda Off DBR Current":dbl=160.0
  in  "Tab Control":T2(tab)=enum."g/m^3"
  out "Water Vapor Number Density  2":cluster{"Y":dbl[], "Y":dbl[]}[](graph)=[{"Y"=array[216 elements], "Y"=[0.075, 0.15, 0.22499999999999998, 0.3, 0.375, 0.45, 0.5249999999999999, 0.6, 0.6749999999999999, 0.7499999999999999, 0.825, 0.8999999999999999, 0.9749999999999999, 1.05, 1.125, 1.2, 1.275, 1.3499999999999999, 1.4249999999999998, 1.5, 1.575, 1.65, 1.7249999999999999, 1.7999999999999998, 1.8749999999999998, 1.95, 2.025, 2.1, 2.1750000000000003, 2.25, 2.325, 2.4, 2.475, 2.5500000000000003, 2.625, 2.7, 2.775, 2.85, 2.9250000000000003, 3.0, 3.075, 3.15, 3.225, 3.3000000000000003, 3.375, 3.45, 3.525, 3.6, 3.675, 3.75, 3.825, 3.9, 3.975, 4.05, 4.125, 4.2, 4.275, 4.35, 4.425, 4.5, 4.575, 4.65, 4.725, 4.8, 4.875, 4.95, 5.025, 5.1, 5.175, 5.25, 5.325, 5.4, 5.475, 5.55, 5.625, 5.7, 5.775, 5.85, 5.925, 6.0, 6.075, 6.15, 6.225, 6.3, 6.375, 6.45, 6.525, 6.6, 6.675, 6.75, 6.825, 6.9, 6.975, 7.05, 7.125, 7.2, 7.2749999999999995, 7.35, 7.425, 7.5, 7.575, 7.6499999999999995, 7.725, 7.8, 7.875, 7.95, 8.024999999999999, 8.1, 8.174999999999999, 8.249999999999998, 8.325, 8.399999999999999, 8.475, 8.549999999999999, 8.624999999999998, 8.7, 8.774999999999999, 8.85, 8.924999999999999, 8.999999999999998, 9.075, 9.149999999999999, 9.225, 9.299999999999999, 9.374999999999998, 9.45, 9.524999999999999, 9.6, 9.674999999999999, 9.749999999999998, 9.825, 9.899999999999999, 9.975, 10.049999999999999, 10.124999999999998, 10.2, 10.274999999999999, 10.35, 10.424999999999999, 10.499999999999998, 10.575, 10.649999999999999, 10.725, 10.799999999999999, 10.874999999999998, 10.95, 11.024999999999999, 11.1, 11.174999999999999, 11.249999999999998, 11.325, 11.399999999999999, 11.475, 11.549999999999999, 11.624999999999998, 11.7, 11.774999999999999, 11.85, 11.924999999999999, 11.999999999999998, 12.075, 12.149999999999999, 12.225, 12.299999999999999, 12.374999999999998, 12.45, 12.524999999999999, 12.6, 12.674999999999999, 12.749999999999998, 12.825, 12.899999999999999, 12.975, 13.049999999999999, 13.124999999999998, 13.2, 13.274999999999999, 13.35, 13.424999999999999, 13.499999999999998, 13.575, 13.649999999999999, 13.725, 13.799999999999999, 13.874999999999998, 13.95, 14.024999999999999, 14.1, 14.174999999999999, 14.249999999999998, 14.325, 14.399999999999999, 14.474999999999998, 14.549999999999999, 14.624999999999998, 14.7, 14.774999999999999, 14.849999999999998, 14.924999999999999, 14.999999999999998, 15.075, 15.149999999999999, 15.224999999999998, 15.299999999999999, 15.374999999999998, 15.45, 15.524999999999999, 15.599999999999998, 15.674999999999999, 15.749999999999998, 15.825, 15.899999999999999, 15.974999999999998, 16.05, 16.125, 16.2, 16.275, 16.349999999999998, 16.424999999999997, 16.5]}, {"Y"=array[216 elements], "Y"=[0.075, 0.15, 0.22499999999999998, 0.3, 0.375, 0.45, 0.5249999999999999, 0.6, 0.6749999999999999, 0.7499999999999999, 0.825, 0.8999999999999999, 0.9749999999999999, 1.05, 1.125, 1.2, 1.275, 1.3499999999999999, 1.4249999999999998, 1.5, 1.575, 1.65, 1.7249999999999999, 1.7999999999999998, 1.8749999999999998, 1.95, 2.025, 2.1, 2.1750000000000003, 2.25, 2.325, 2.4, 2.475, 2.5500000000000003, 2.625, 2.7, 2.775, 2.85, 2.9250000000000003, 3.0, 3.075, 3.15, 3.225, 3.3000000000000003, 3.375, 3.45, 3.525, 3.6, 3.675, 3.75, 3.825, 3.9, 3.975, 4.05, 4.125, 4.2, 4.275, 4.35, 4.425, 4.5, 4.575, 4.65, 4.725, 4.8, 4.875, 4.95, 5.025, 5.1, 5.175, 5.25, 5.325, 5.4, 5.475, 5.55, 5.625, 5.7, 5.775, 5.85, 5.925, 6.0, 6.075, 6.15, 6.225, 6.3, 6.375, 6.45, 6.525, 6.6, 6.675, 6.75, 6.825, 6.9, 6.975, 7.05, 7.125, 7.2, 7.2749999999999995, 7.35, 7.425, 7.5, 7.575, 7.6499999999999995, 7.725, 7.8, 7.875, 7.95, 8.024999999999999, 8.1, 8.174999999999999, 8.249999999999998, 8.325, 8.399999999999999, 8.475, 8.549999999999999, 8.624999999999998, 8.7, 8.774999999999999, 8.85, 8.924999999999999, 8.999999999999998, 9.075, 9.149999999999999, 9.225, 9.299999999999999, 9.374999999999998, 9.45, 9.524999999999999, 9.6, 9.674999999999999, 9.749999999999998, 9.825, 9.899999999999999, 9.975, 10.049999999999999, 10.124999999999998, 10.2, 10.274999999999999, 10.35, 10.424999999999999, 10.499999999999998, 10.575, 10.649999999999999, 10.725, 10.799999999999999, 10.874999999999998, 10.95, 11.024999999999999, 11.1, 11.174999999999999, 11.249999999999998, 11.325, 11.399999999999999, 11.475, 11.549999999999999, 11.624999999999998, 11.7, 11.774999999999999, 11.85, 11.924999999999999, 11.999999999999998, 12.075, 12.149999999999999, 12.225, 12.299999999999999, 12.374999999999998, 12.45, 12.524999999999999, 12.6, 12.674999999999999, 12.749999999999998, 12.825, 12.899999999999999, 12.975, 13.049999999999999, 13.124999999999998, 13.2, 13.274999999999999, 13.35, 13.424999999999999, 13.499999999999998, 13.575, 13.649999999999999, 13.725, 13.799999999999999, 13.874999999999998, 13.95, 14.024999999999999, 14.1, 14.174999999999999, 14.249999999999998, 14.325, 14.399999999999999, 14.474999999999998, 14.549999999999999, 14.624999999999998, 14.7, 14.774999999999999, 14.849999999999998, 14.924999999999999, 14.999999999999998, 15.075, 15.149999999999999, 15.224999999999998, 15.299999999999999, 15.374999999999998, 15.45, 15.524999999999999, 15.599999999999998, 15.674999999999999, 15.749999999999998, 15.825, 15.899999999999999, 15.974999999999998, 16.05, 16.125, 16.2, 16.275, 16.349999999999998, 16.424999999999997, 16.5]}]
  out "Absolute Humidity":cluster{"Y":dbl[], "Y":dbl[]}[](graph)=[{"Y"=array[216 elements], "Y"=[0.075, 0.15, 0.22499999999999998, 0.3, 0.375, 0.45, 0.5249999999999999, 0.6, 0.6749999999999999, 0.7499999999999999, 0.825, 0.8999999999999999, 0.9749999999999999, 1.05, 1.125, 1.2, 1.275, 1.3499999999999999, 1.4249999999999998, 1.5, 1.575, 1.65, 1.7249999999999999, 1.7999999999999998, 1.8749999999999998, 1.95, 2.025, 2.1, 2.1750000000000003, 2.25, 2.325, 2.4, 2.475, 2.5500000000000003, 2.625, 2.7, 2.775, 2.85, 2.9250000000000003, 3.0, 3.075, 3.15, 3.225, 3.3000000000000003, 3.375, 3.45, 3.525, 3.6, 3.675, 3.75, 3.825, 3.9, 3.975, 4.05, 4.125, 4.2, 4.275, 4.35, 4.425, 4.5, 4.575, 4.65, 4.725, 4.8, 4.875, 4.95, 5.025, 5.1, 5.175, 5.25, 5.325, 5.4, 5.475, 5.55, 5.625, 5.7, 5.775, 5.85, 5.925, 6.0, 6.075, 6.15, 6.225, 6.3, 6.375, 6.45, 6.525, 6.6, 6.675, 6.75, 6.825, 6.9, 6.975, 7.05, 7.125, 7.2, 7.2749999999999995, 7.35, 7.425, 7.5, 7.575, 7.6499999999999995, 7.725, 7.8, 7.875, 7.95, 8.024999999999999, 8.1, 8.174999999999999, 8.249999999999998, 8.325, 8.399999999999999, 8.475, 8.549999999999999, 8.624999999999998, 8.7, 8.774999999999999, 8.85, 8.924999999999999, 8.999999999999998, 9.075, 9.149999999999999, 9.225, 9.299999999999999, 9.374999999999998, 9.45, 9.524999999999999, 9.6, 9.674999999999999, 9.749999999999998, 9.825, 9.899999999999999, 9.975, 10.049999999999999, 10.124999999999998, 10.2, 10.274999999999999, 10.35, 10.424999999999999, 10.499999999999998, 10.575, 10.649999999999999, 10.725, 10.799999999999999, 10.874999999999998, 10.95, 11.024999999999999, 11.1, 11.174999999999999, 11.249999999999998, 11.325, 11.399999999999999, 11.475, 11.549999999999999, 11.624999999999998, 11.7, 11.774999999999999, 11.85, 11.924999999999999, 11.999999999999998, 12.075, 12.149999999999999, 12.225, 12.299999999999999, 12.374999999999998, 12.45, 12.524999999999999, 12.6, 12.674999999999999, 12.749999999999998, 12.825, 12.899999999999999, 12.975, 13.049999999999999, 13.124999999999998, 13.2, 13.274999999999999, 13.35, 13.424999999999999, 13.499999999999998, 13.575, 13.649999999999999, 13.725, 13.799999999999999, 13.874999999999998, 13.95, 14.024999999999999, 14.1, 14.174999999999999, 14.249999999999998, 14.325, 14.399999999999999, 14.474999999999998, 14.549999999999999, 14.624999999999998, 14.7, 14.774999999999999, 14.849999999999998, 14.924999999999999, 14.999999999999998, 15.075, 15.149999999999999, 15.224999999999998, 15.299999999999999, 15.374999999999998, 15.45, 15.524999999999999, 15.599999999999998, 15.674999999999999, 15.749999999999998, 15.825, 15.899999999999999, 15.974999999999998, 16.05, 16.125, 16.2, 16.275, 16.349999999999998, 16.424999999999997, 16.5]}, {"Y"=array[216 elements], "Y"=[0.075, 0.15, 0.22499999999999998, 0.3, 0.375, 0.45, 0.5249999999999999, 0.6, 0.6749999999999999, 0.7499999999999999, 0.825, 0.8999999999999999, 0.9749999999999999, 1.05, 1.125, 1.2, 1.275, 1.3499999999999999, 1.4249999999999998, 1.5, 1.575, 1.65, 1.7249999999999999, 1.7999999999999998, 1.8749999999999998, 1.95, 2.025, 2.1, 2.1750000000000003, 2.25, 2.325, 2.4, 2.475, 2.5500000000000003, 2.625, 2.7, 2.775, 2.85, 2.9250000000000003, 3.0, 3.075, 3.15, 3.225, 3.3000000000000003, 3.375, 3.45, 3.525, 3.6, 3.675, 3.75, 3.825, 3.9, 3.975, 4.05, 4.125, 4.2, 4.275, 4.35, 4.425, 4.5, 4.575, 4.65, 4.725, 4.8, 4.875, 4.95, 5.025, 5.1, 5.175, 5.25, 5.325, 5.4, 5.475, 5.55, 5.625, 5.7, 5.775, 5.85, 5.925, 6.0, 6.075, 6.15, 6.225, 6.3, 6.375, 6.45, 6.525, 6.6, 6.675, 6.75, 6.825, 6.9, 6.975, 7.05, 7.125, 7.2, 7.2749999999999995, 7.35, 7.425, 7.5, 7.575, 7.6499999999999995, 7.725, 7.8, 7.875, 7.95, 8.024999999999999, 8.1, 8.174999999999999, 8.249999999999998, 8.325, 8.399999999999999, 8.475, 8.549999999999999, 8.624999999999998, 8.7, 8.774999999999999, 8.85, 8.924999999999999, 8.999999999999998, 9.075, 9.149999999999999, 9.225, 9.299999999999999, 9.374999999999998, 9.45, 9.524999999999999, 9.6, 9.674999999999999, 9.749999999999998, 9.825, 9.899999999999999, 9.975, 10.049999999999999, 10.124999999999998, 10.2, 10.274999999999999, 10.35, 10.424999999999999, 10.499999999999998, 10.575, 10.649999999999999, 10.725, 10.799999999999999, 10.874999999999998, 10.95, 11.024999999999999, 11.1, 11.174999999999999, 11.249999999999998, 11.325, 11.399999999999999, 11.475, 11.549999999999999, 11.624999999999998, 11.7, 11.774999999999999, 11.85, 11.924999999999999, 11.999999999999998, 12.075, 12.149999999999999, 12.225, 12.299999999999999, 12.374999999999998, 12.45, 12.524999999999999, 12.6, 12.674999999999999, 12.749999999999998, 12.825, 12.899999999999999, 12.975, 13.049999999999999, 13.124999999999998, 13.2, 13.274999999999999, 13.35, 13.424999999999999, 13.499999999999998, 13.575, 13.649999999999999, 13.725, 13.799999999999999, 13.874999999999998, 13.95, 14.024999999999999, 14.1, 14.174999999999999, 14.249999999999998, 14.325, 14.399999999999999, 14.474999999999998, 14.549999999999999, 14.624999999999998, 14.7, 14.774999999999999, 14.849999999999998, 14.924999999999999, 14.999999999999998, 15.075, 15.149999999999999, 15.224999999999998, 15.299999999999999, 15.374999999999998, 15.45, 15.524999999999999, 15.599999999999998, 15.674999999999999, 15.749999999999998, 15.825, 15.899999999999999, 15.974999999999998, 16.05, 16.125, 16.2, 16.275, 16.349999999999998, 16.424999999999997, 16.5]}]
  out "NRB plot":cluster{"Y":dbl[], "Y":dbl[]}[](graph)=[{"Y"=array[217 elements], "Y"=[0.075, 0.15, 0.22499999999999998, 0.3, 0.375, 0.45, 0.5249999999999999, 0.6, 0.6749999999999999, 0.7499999999999999, 0.825, 0.8999999999999999, 0.9749999999999999, 1.05, 1.125, 1.2, 1.275, 1.3499999999999999, 1.4249999999999998, 1.5, 1.575, 1.65, 1.7249999999999999, 1.7999999999999998, 1.8749999999999998, 1.95, 2.025, 2.1, 2.1750000000000003, 2.25, 2.325, 2.4, 2.475, 2.5500000000000003, 2.625, 2.7, 2.775, 2.85, 2.9250000000000003, 3.0, 3.075, 3.15, 3.225, 3.3000000000000003, 3.375, 3.45, 3.525, 3.6, 3.675, 3.75, 3.825, 3.9, 3.975, 4.05, 4.125, 4.2, 4.275, 4.35, 4.425, 4.5, 4.575, 4.65, 4.725, 4.8, 4.875, 4.95, 5.025, 5.1, 5.175, 5.25, 5.325, 5.4, 5.475, 5.55, 5.625, 5.7, 5.775, 5.85, 5.925, 6.0, 6.075, 6.15, 6.225, 6.3, 6.375, 6.45, 6.525, 6.6, 6.675, 6.75, 6.825, 6.9, 6.975, 7.05, 7.125, 7.2, 7.2749999999999995, 7.35, 7.425, 7.5, 7.575, 7.6499999999999995, 7.725, 7.8, 7.875, 7.95, 8.024999999999999, 8.1, 8.174999999999999, 8.249999999999998, 8.325, 8.399999999999999, 8.475, 8.549999999999999, 8.624999999999998, 8.7, 8.774999999999999, 8.85, 8.924999999999999, 8.999999999999998, 9.075, 9.149999999999999, 9.225, 9.299999999999999, 9.374999999999998, 9.45, 9.524999999999999, 9.6, 9.674999999999999, 9.749999999999998, 9.825, 9.899999999999999, 9.975, 10.049999999999999, 10.124999999999998, 10.2, 10.274999999999999, 10.35, 10.424999999999999, 10.499999999999998, 10.575, 10.649999999999999, 10.725, 10.799999999999999, 10.874999999999998, 10.95, 11.024999999999999, 11.1, 11.174999999999999, 11.249999999999998, 11.325, 11.399999999999999, 11.475, 11.549999999999999, 11.624999999999998, 11.7, 11.774999999999999, 11.85, 11.924999999999999, 11.999999999999998, 12.075, 12.149999999999999, 12.225, 12.299999999999999, 12.374999999999998, 12.45, 12.524999999999999, 12.6, 12.674999999999999, 12.749999999999998, 12.825, 12.899999999999999, 12.975, 13.049999999999999, 13.124999999999998, 13.2, 13.274999999999999, 13.35, 13.424999999999999, 13.499999999999998, 13.575, 13.649999999999999, 13.725, 13.799999999999999, 13.874999999999998, 13.95, 14.024999999999999, 14.1, 14.174999999999999, 14.249999999999998, 14.325, 14.399999999999999, 14.474999999999998, 14.549999999999999, 14.624999999999998, 14.7, 14.774999999999999, 14.849999999999998, 14.924999999999999, 14.999999999999998, 15.075, 15.149999999999999, 15.224999999999998, 15.299999999999999, 15.374999999999998, 15.45, 15.524999999999999, 15.599999999999998, 15.674999999999999, 15.749999999999998, 15.825, 15.899999999999999, 15.974999999999998, 16.05, 16.125, 16.2, 16.275, 16.349999999999998, 16.424999999999997, 16.5]}, {"Y"=array[217 elements], "Y"=[0.075, 0.15, 0.22499999999999998, 0.3, 0.375, 0.45, 0.5249999999999999, 0.6, 0.6749999999999999, 0.7499999999999999, 0.825, 0.8999999999999999, 0.9749999999999999, 1.05, 1.125, 1.2, 1.275, 1.3499999999999999, 1.4249999999999998, 1.5, 1.575, 1.65, 1.7249999999999999, 1.7999999999999998, 1.8749999999999998, 1.95, 2.025, 2.1, 2.1750000000000003, 2.25, 2.325, 2.4, 2.475, 2.5500000000000003, 2.625, 2.7, 2.775, 2.85, 2.9250000000000003, 3.0, 3.075, 3.15, 3.225, 3.3000000000000003, 3.375, 3.45, 3.525, 3.6, 3.675, 3.75, 3.825, 3.9, 3.975, 4.05, 4.125, 4.2, 4.275, 4.35, 4.425, 4.5, 4.575, 4.65, 4.725, 4.8, 4.875, 4.95, 5.025, 5.1, 5.175, 5.25, 5.325, 5.4, 5.475, 5.55, 5.625, 5.7, 5.775, 5.85, 5.925, 6.0, 6.075, 6.15, 6.225, 6.3, 6.375, 6.45, 6.525, 6.6, 6.675, 6.75, 6.825, 6.9, 6.975, 7.05, 7.125, 7.2, 7.2749999999999995, 7.35, 7.425, 7.5, 7.575, 7.6499999999999995, 7.725, 7.8, 7.875, 7.95, 8.024999999999999, 8.1, 8.174999999999999, 8.249999999999998, 8.325, 8.399999999999999, 8.475, 8.549999999999999, 8.624999999999998, 8.7, 8.774999999999999, 8.85, 8.924999999999999, 8.999999999999998, 9.075, 9.149999999999999, 9.225, 9.299999999999999, 9.374999999999998, 9.45, 9.524999999999999, 9.6, 9.674999999999999, 9.749999999999998, 9.825, 9.899999999999999, 9.975, 10.049999999999999, 10.124999999999998, 10.2, 10.274999999999999, 10.35, 10.424999999999999, 10.499999999999998, 10.575, 10.649999999999999, 10.725, 10.799999999999999, 10.874999999999998, 10.95, 11.024999999999999, 11.1, 11.174999999999999, 11.249999999999998, 11.325, 11.399999999999999, 11.475, 11.549999999999999, 11.624999999999998, 11.7, 11.774999999999999, 11.85, 11.924999999999999, 11.999999999999998, 12.075, 12.149999999999999, 12.225, 12.299999999999999, 12.374999999999998, 12.45, 12.524999999999999, 12.6, 12.674999999999999, 12.749999999999998, 12.825, 12.899999999999999, 12.975, 13.049999999999999, 13.124999999999998, 13.2, 13.274999999999999, 13.35, 13.424999999999999, 13.499999999999998, 13.575, 13.649999999999999, 13.725, 13.799999999999999, 13.874999999999998, 13.95, 14.024999999999999, 14.1, 14.174999999999999, 14.249999999999998, 14.325, 14.399999999999999, 14.474999999999998, 14.549999999999999, 14.624999999999998, 14.7, 14.774999999999999, 14.849999999999998, 14.924999999999999, 14.999999999999998, 15.075, 15.149999999999999, 15.224999999999998, 15.299999999999999, 15.374999999999998, 15.45, 15.524999999999999, 15.599999999999998, 15.674999999999999, 15.749999999999998, 15.825, 15.899999999999999, 15.974999999999998, 16.05, 16.125, 16.2, 16.275, 16.349999999999998, 16.424999999999997, 16.5]}]
  in  "background length":i32=10
  out "Correction":cluster{"Y":dbl[], "Y":dbl[]}[](graph)=[{"Y"=array[217 elements], "Y"=[0.075, 0.15, 0.22499999999999998, 0.3, 0.375, 0.45, 0.5249999999999999, 0.6, 0.6749999999999999, 0.7499999999999999, 0.825, 0.8999999999999999, 0.9749999999999999, 1.05, 1.125, 1.2, 1.275, 1.3499999999999999, 1.4249999999999998, 1.5, 1.575, 1.65, 1.7249999999999999, 1.7999999999999998, 1.8749999999999998, 1.95, 2.025, 2.1, 2.1750000000000003, 2.25, 2.325, 2.4, 2.475, 2.5500000000000003, 2.625, 2.7, 2.775, 2.85, 2.9250000000000003, 3.0, 3.075, 3.15, 3.225, 3.3000000000000003, 3.375, 3.45, 3.525, 3.6, 3.675, 3.75, 3.825, 3.9, 3.975, 4.05, 4.125, 4.2, 4.275, 4.35, 4.425, 4.5, 4.575, 4.65, 4.725, 4.8, 4.875, 4.95, 5.025, 5.1, 5.175, 5.25, 5.325, 5.4, 5.475, 5.55, 5.625, 5.7, 5.775, 5.85, 5.925, 6.0, 6.075, 6.15, 6.225, 6.3, 6.375, 6.45, 6.525, 6.6, 6.675, 6.75, 6.825, 6.9, 6.975, 7.05, 7.125, 7.2, 7.2749999999999995, 7.35, 7.425, 7.5, 7.575, 7.6499999999999995, 7.725, 7.8, 7.875, 7.95, 8.024999999999999, 8.1, 8.174999999999999, 8.249999999999998, 8.325, 8.399999999999999, 8.475, 8.549999999999999, 8.624999999999998, 8.7, 8.774999999999999, 8.85, 8.924999999999999, 8.999999999999998, 9.075, 9.149999999999999, 9.225, 9.299999999999999, 9.374999999999998, 9.45, 9.524999999999999, 9.6, 9.674999999999999, 9.749999999999998, 9.825, 9.899999999999999, 9.975, 10.049999999999999, 10.124999999999998, 10.2, 10.274999999999999, 10.35, 10.424999999999999, 10.499999999999998, 10.575, 10.649999999999999, 10.725, 10.799999999999999, 10.874999999999998, 10.95, 11.024999999999999, 11.1, 11.174999999999999, 11.249999999999998, 11.325, 11.399999999999999, 11.475, 11.549999999999999, 11.624999999999998, 11.7, 11.774999999999999, 11.85, 11.924999999999999, 11.999999999999998, 12.075, 12.149999999999999, 12.225, 12.299999999999999, 12.374999999999998, 12.45, 12.524999999999999, 12.6, 12.674999999999999, 12.749999999999998, 12.825, 12.899999999999999, 12.975, 13.049999999999999, 13.124999999999998, 13.2, 13.274999999999999, 13.35, 13.424999999999999, 13.499999999999998, 13.575, 13.649999999999999, 13.725, 13.799999999999999, 13.874999999999998, 13.95, 14.024999999999999, 14.1, 14.174999999999999, 14.249999999999998, 14.325, 14.399999999999999, 14.474999999999998, 14.549999999999999, 14.624999999999998, 14.7, 14.774999999999999, 14.849999999999998, 14.924999999999999, 14.999999999999998, 15.075, 15.149999999999999, 15.224999999999998, 15.299999999999999, 15.374999999999998, 15.45, 15.524999999999999, 15.599999999999998, 15.674999999999999, 15.749999999999998, 15.825, 15.899999999999999, 15.974999999999998, 16.05, 16.125, 16.2, 16.275, 16.349999999999998, 16.424999999999997, 16.5]}, {"Y"=array[217 elements], "Y"=[0.075, 0.15, 0.22499999999999998, 0.3, 0.375, 0.45, 0.5249999999999999, 0.6, 0.6749999999999999, 0.7499999999999999, 0.825, 0.8999999999999999, 0.9749999999999999, 1.05, 1.125, 1.2, 1.275, 1.3499999999999999, 1.4249999999999998, 1.5, 1.575, 1.65, 1.7249999999999999, 1.7999999999999998, 1.8749999999999998, 1.95, 2.025, 2.1, 2.1750000000000003, 2.25, 2.325, 2.4, 2.475, 2.5500000000000003, 2.625, 2.7, 2.775, 2.85, 2.9250000000000003, 3.0, 3.075, 3.15, 3.225, 3.3000000000000003, 3.375, 3.45, 3.525, 3.6, 3.675, 3.75, 3.825, 3.9, 3.975, 4.05, 4.125, 4.2, 4.275, 4.35, 4.425, 4.5, 4.575, 4.65, 4.725, 4.8, 4.875, 4.95, 5.025, 5.1, 5.175, 5.25, 5.325, 5.4, 5.475, 5.55, 5.625, 5.7, 5.775, 5.85, 5.925, 6.0, 6.075, 6.15, 6.225, 6.3, 6.375, 6.45, 6.525, 6.6, 6.675, 6.75, 6.825, 6.9, 6.975, 7.05, 7.125, 7.2, 7.2749999999999995, 7.35, 7.425, 7.5, 7.575, 7.6499999999999995, 7.725, 7.8, 7.875, 7.95, 8.024999999999999, 8.1, 8.174999999999999, 8.249999999999998, 8.325, 8.399999999999999, 8.475, 8.549999999999999, 8.624999999999998, 8.7, 8.774999999999999, 8.85, 8.924999999999999, 8.999999999999998, 9.075, 9.149999999999999, 9.225, 9.299999999999999, 9.374999999999998, 9.45, 9.524999999999999, 9.6, 9.674999999999999, 9.749999999999998, 9.825, 9.899999999999999, 9.975, 10.049999999999999, 10.124999999999998, 10.2, 10.274999999999999, 10.35, 10.424999999999999, 10.499999999999998, 10.575, 10.649999999999999, 10.725, 10.799999999999999, 10.874999999999998, 10.95, 11.024999999999999, 11.1, 11.174999999999999, 11.249999999999998, 11.325, 11.399999999999999, 11.475, 11.549999999999999, 11.624999999999998, 11.7, 11.774999999999999, 11.85, 11.924999999999999, 11.999999999999998, 12.075, 12.149999999999999, 12.225, 12.299999999999999, 12.374999999999998, 12.45, 12.524999999999999, 12.6, 12.674999999999999, 12.749999999999998, 12.825, 12.899999999999999, 12.975, 13.049999999999999, 13.124999999999998, 13.2, 13.274999999999999, 13.35, 13.424999999999999, 13.499999999999998, 13.575, 13.649999999999999, 13.725, 13.799999999999999, 13.874999999999998, 13.95, 14.024999999999999, 14.1, 14.174999999999999, 14.249999999999998, 14.325, 14.399999999999999, 14.474999999999998, 14.549999999999999, 14.624999999999998, 14.7, 14.774999999999999, 14.849999999999998, 14.924999999999999, 14.999999999999998, 15.075, 15.149999999999999, 15.224999999999998, 15.299999999999999, 15.374999999999998, 15.45, 15.524999999999999, 15.599999999999998, 15.674999999999999, 15.749999999999998, 15.825, 15.899999999999999, 15.974999999999998, 16.05, 16.125, 16.2, 16.275, 16.349999999999998, 16.424999999999997, 16.5]}]
  in  "dead time":dbl=3.7e-08
  out "Optical Depth":cluster{"Y":dbl[], "Y":dbl[]}[](graph)=[{"Y"=array[217 elements], "Y"=[0.075, 0.15, 0.22499999999999998, 0.3, 0.375, 0.45, 0.5249999999999999, 0.6, 0.6749999999999999, 0.7499999999999999, 0.825, 0.8999999999999999, 0.9749999999999999, 1.05, 1.125, 1.2, 1.275, 1.3499999999999999, 1.4249999999999998, 1.5, 1.575, 1.65, 1.7249999999999999, 1.7999999999999998, 1.8749999999999998, 1.95, 2.025, 2.1, 2.1750000000000003, 2.25, 2.325, 2.4, 2.475, 2.5500000000000003, 2.625, 2.7, 2.775, 2.85, 2.9250000000000003, 3.0, 3.075, 3.15, 3.225, 3.3000000000000003, 3.375, 3.45, 3.525, 3.6, 3.675, 3.75, 3.825, 3.9, 3.975, 4.05, 4.125, 4.2, 4.275, 4.35, 4.425, 4.5, 4.575, 4.65, 4.725, 4.8, 4.875, 4.95, 5.025, 5.1, 5.175, 5.25, 5.325, 5.4, 5.475, 5.55, 5.625, 5.7, 5.775, 5.85, 5.925, 6.0, 6.075, 6.15, 6.225, 6.3, 6.375, 6.45, 6.525, 6.6, 6.675, 6.75, 6.825, 6.9, 6.975, 7.05, 7.125, 7.2, 7.2749999999999995, 7.35, 7.425, 7.5, 7.575, 7.6499999999999995, 7.725, 7.8, 7.875, 7.95, 8.024999999999999, 8.1, 8.174999999999999, 8.249999999999998, 8.325, 8.399999999999999, 8.475, 8.549999999999999, 8.624999999999998, 8.7, 8.774999999999999, 8.85, 8.924999999999999, 8.999999999999998, 9.075, 9.149999999999999, 9.225, 9.299999999999999, 9.374999999999998, 9.45, 9.524999999999999, 9.6, 9.674999999999999, 9.749999999999998, 9.825, 9.899999999999999, 9.975, 10.049999999999999, 10.124999999999998, 10.2, 10.274999999999999, 10.35, 10.424999999999999, 10.499999999999998, 10.575, 10.649999999999999, 10.725, 10.799999999999999, 10.874999999999998, 10.95, 11.024999999999999, 11.1, 11.174999999999999, 11.249999999999998, 11.325, 11.399999999999999, 11.475, 11.549999999999999, 11.624999999999998, 11.7, 11.774999999999999, 11.85, 11.924999999999999, 11.999999999999998, 12.075, 12.149999999999999, 12.225, 12.299999999999999, 12.374999999999998, 12.45, 12.524999999999999, 12.6, 12.674999999999999, 12.749999999999998, 12.825, 12.899999999999999, 12.975, 13.049999999999999, 13.124999999999998, 13.2, 13.274999999999999, 13.35, 13.424999999999999, 13.499999999999998, 13.575, 13.649999999999999, 13.725, 13.799999999999999, 13.874999999999998, 13.95, 14.024999999999999, 14.1, 14.174999999999999, 14.249999999999998, 14.325, 14.399999999999999, 14.474999999999998, 14.549999999999999, 14.624999999999998, 14.7, 14.774999999999999, 14.849999999999998, 14.924999999999999, 14.999999999999998, 15.075, 15.149999999999999, 15.224999999999998, 15.299999999999999, 15.374999999999998, 15.45, 15.524999999999999, 15.599999999999998, 15.674999999999999, 15.749999999999998, 15.825, 15.899999999999999, 15.974999999999998, 16.05, 16.125, 16.2, 16.275, 16.349999999999998, 16.424999999999997, 16.5]}] caption="XY Graph"
  out "RingBuffer offline far":dbl[][](array[numeric])
  out "RingBuffer aerosol far":dbl[][](array[numeric])
  in  "Weather":T3(tab)=enum."Pulse Energy (Micro Joule)"
  in  "Temperature (C)":dbl=15.0
  out "Temperature (C)":dbl(graph)=15.0
  in  "Pressure (mbar or hPa)":dbl=832.0
  out "Pressure (mb)":dbl(graph)=832.0
  out "Relative Humdity (%)":dbl(graph)=40.0
  out "Pulse Energy (Micro Joule)":T4(graph)={"Online Pulse Energy"=5.089021, "Pulse Energy Offline"=5.111813}
  out "?":cluster{"mean":dbl, "mean":dbl}(graph)={"mean"=21620.0, "mean"=327180.0}
  out "Index":i32=54
  out "Aerosol Smoothed":dbl[](array[numeric])=[18132.924074074064, 20901.215740740732, 11453.206481481477, 68.77592592592589, 102.11388888888885, 160.14629629629627, 238.71111111111122, 341.29907407407416, 463.20648148148155, 602.5074074074075, 760.4657407407406, 919.8638888888884, 1070.9611111111103, 1197.2620370370364, 1299.5444444444438, 1378.2990740740734, 1399.3129629629625, 1331.7111111111108, 1243.9148148148142, 1243.1416666666662, 1297.6231481481477, 1421.0351851851851, 1690.4333333333334, 1966.4796296296292, 2067.6925925925925, 2035.322222222222, 1936.8453703703701, 1753.7759259259258, 1502.8731481481477, 1270.1231481481475, 1139.8083333333327, 1093.8685185185177, 1043.9055555555549, 961.1648148148142, 882.6370370370366, 818.248148148148, 757.3499999999999, 706.0259259259258, 660.387037037037, 614.0907407407408, 575.4055555555556, 542.7342592592593, 501.10925925925926, 427.93796296296296, 337.1972222222223, 266.78055555555574, 208.0675925925927, 161.41018518518518, 145.8361111111111, 142.70648148148146, 134.92870370370366, 132.7898148148148, 150.0953703703704, 184.02592592592597, 229.12314814814826, 274.73888888888905, 304.7944444444446, 311.4472222222223, 280.49351851851867, 218.01666666666674, 156.89166666666665, 111.1185185185185, 82.56759259259258, 106.13240740740738, 219.56759259259266, 300.10000000000014, 219.35000000000008, 105.54444444444441, 66.63703703703699, 58.053703703703675, 49.76666666666665, 46.78518518518517, 105.05833333333334, 356.01203703703703, 644.2157407407408, 572.2157407407408, 265.1138888888889, 84.49814814814813, 38.10462962962963, 27.73425925925926, 23.99351851851852, 23.414814814814815, 23.613888888888887, 22.461111111111116, 21.275925925925936, 20.45648148148149, 19.377777777777784, 18.150925925925932, 16.502777777777787, 14.924074074074083, 14.262037037037047, 15.391666666666676, 15.678703703703714, 14.905555555555566, 14.780555555555562, 21.447222222222226, 47.41018518518517, 87.37314814814812, 125.8962962962963, 143.22962962962964, 138.81759259259258, 143.95648148148146, 148.7111111111111, 104.39166666666664, 39.72962962962961, 11.479629629629635, 9.600000000000001, 10.48888888888889, 10.044444444444444, 9.215740740740742, 8.192592592592591, 8.613888888888887, 7.201851851851852, 6.757407407407408, 7.562962962962963, 7.22962962962963, 6.757407407407408, 6.942592592592593, 6.687962962962963, 6.34074074074074, 6.618518518518518, 5.581481481481482, 6.146296296296297, 7.414814814814815, 9.873148148148152, 16.34074074074075, 19.34537037037038, 18.461111111111123, 17.303703703703714, 9.516666666666671, 3.720370370370372, 4.12314814814815, 4.0120370370370395, 3.5722222222222233, 2.650925925925927, 3.0305555555555572, 4.211111111111112, 4.183333333333335, 2.5583333333333345, 2.576851851851853, 3.924074074074076, 4.072222222222224, 2.3638888888888903, 1.600000000000001, 2.86388888888889, 3.12314814814815, 3.058333333333335, 2.4796296296296303, 2.1462962962962964, 1.8546296296296299, 2.5259259259259266, 3.2944444444444456, 3.252777777777779, 2.437962962962964, 1.1046296296296305, 1.275925925925927, 1.641666666666668, 1.7157407407407415, 1.8731481481481487, 1.8222222222222224, 1.169444444444445, 1.090740740740742, 1.766666666666667, 2.206481481481482, 0.8453703703703717, 0.40555555555555634, 1.424074074074075, 0.7851851851851862, 0.8453703703703709, 1.2712962962962966, 1.5259259259259266, 1.4564814814814822, 0.5166666666666677, 1.058333333333334, 1.2805555555555563, 1.387037037037038, 1.7435185185185196, 0.8129629629629641, 0.1740740740740751, 0.8638888888888899, 1.3175925925925938, 1.0259259259259272, 1.3916666666666675, 1.9750000000000005, 1.3824074074074082, -0.5481481481481472, -0.5990740740740732, 1.479629629629631, 1.826851851851853, 1.4611111111111121, 1.4935185185185196, 0.9703703703703711, -0.38148148148148053, -0.9138888888888879, -0.437037037037036, 0.512037037037038, 0.9981481481481491, 1.0861111111111121, 1.0768518518518528, 1.9750000000000012, 1.951851851851853, 0.2990740740740751, 0.6370370370370381, 1.3129629629629638, 1.5768518518518524, 0.3870370370370377, -0.3953703703703694, -0.34907407407407304, -0.6962962962962953, 0.07222222222222324, -0.11759259259259158, -0.7287037037037027, -0.05277777777777676, 0.4981481481481492, 0.7388888888888899, 0.7342592592592602, 0.47037037037037127]
  out "Off-Line  Bin Readings":dbl[](array[numeric])=[17815.0, 19115.0, 23433.0, 178.0, 207.0, 274.0, 349.0, 425.0, 581.0, 656.0, 885.0, 988.0, 1159.0, 1409.0, 1600.0, 1601.0, 1704.0, 1606.0, 1436.0, 1568.0, 1532.0, 1626.0, 2018.0, 2262.0, 2394.0, 2469.0, 2334.0, 2100.0, 1786.0, 1588.0, 1365.0, 1320.0, 1324.0, 1232.0, 1087.0, 1009.0, 913.0, 852.0, 825.0, 773.0, 778.0, 720.0, 707.0, 691.0, 517.0, 447.0, 383.0, 342.0, 259.0, 275.0, 269.0, 239.0, 283.0, 293.0, 325.0, 415.0, 413.0, 460.0, 423.0, 388.0, 311.0, 253.0, 203.0, 204.0, 263.0, 464.0, 485.0, 268.0, 178.0, 169.0, 167.0, 128.0, 149.0, 246.0, 677.0, 936.0, 637.0, 249.0, 147.0, 129.0, 140.0, 152.0, 147.0, 137.0, 148.0, 135.0, 115.0, 122.0, 138.0, 129.0, 123.0, 111.0, 114.0, 139.0, 116.0, 126.0, 127.0, 206.0, 206.0, 248.0, 256.0, 231.0, 246.0, 285.0, 174.0, 136.0, 122.0, 157.0, 123.0, 123.0, 121.0, 121.0, 111.0, 110.0, 100.0, 124.0, 131.0, 139.0, 110.0, 128.0, 121.0, 102.0, 130.0, 109.0, 112.0, 107.0, 98.0, 100.0, 99.0, 122.0, 113.0, 117.0, 100.0, 118.0, 111.0, 125.0, 111.0, 97.0, 117.0, 106.0, 116.0, 104.0, 112.0, 113.0, 144.0, 107.0, 106.0, 102.0, 109.0, 110.0, 126.0, 129.0, 95.0, 127.0, 128.0, 100.0, 103.0, 116.0, 99.0, 107.0, 106.0, 117.0, 103.0, 109.0, 125.0, 130.0, 114.0, 106.0, 111.0, 127.0, 132.0, 126.0, 123.0, 129.0, 134.0, 111.0, 108.0, 90.0, 106.0, 123.0, 122.0, 108.0, 112.0, 109.0, 110.0, 115.0, 109.0, 127.0, 107.0, 115.0, 125.0, 124.0, 115.0, 108.0, 119.0, 116.0, 123.0, 103.0, 116.0, 128.0, 106.0, 89.0, 109.0, 122.0, 124.0, 109.0, 118.0, 114.0, 110.0, 87.0, 117.0, 123.0, 120.0, 102.0, 108.0, 112.0, 105.0, 112.0, 95.0]
  out "Off-Line Smoothed":dbl[](array[numeric])=[18133.184641638247, 20883.78020477818, 11445.612969283287, 70.39965870307174, 104.06689419795234, 161.3331058020479, 240.57372013651866, 341.3092150170645, 462.83993174061385, 605.3774744027298, 766.4883959044364, 931.7597269624576, 1082.5822525597277, 1213.2972696245747, 1326.0310580204791, 1404.672696245735, 1412.720477815701, 1361.648805460752, 1332.4252559726974, 1364.3126279863495, 1414.9491467576809, 1475.0344709897627, 1632.2597269624591, 1919.355290102391, 2144.587372013654, 2177.285324232084, 2101.4832764505136, 1978.8757679180906, 1795.746075085326, 1544.2802047781588, 1297.1812286689437, 1129.3467576791822, 1038.3279863481237, 964.9406143344718, 883.2511945392494, 814.4167235494879, 762.2836177474398, 718.5037542662112, 674.211945392491, 628.2563139931735, 585.0105802047776, 548.4747440273032, 503.4559726962452, 429.6010238907845, 347.0003412969279, 276.524232081911, 211.49351535836178, 162.4116040955633, 142.59419795221856, 139.56689419795234, 136.9013651877134, 131.4354948805462, 131.23412969283294, 145.79385665529026, 177.62491467576808, 222.79044368600682, 266.64368600682576, 294.3808873720133, 292.2119453924911, 245.41843003412953, 176.03105802047787, 121.60784982935166, 87.79726962457349, 89.57542662116052, 169.72730375426625, 273.65904436860046, 249.96450511945375, 132.5993174061434, 68.59078498293522, 58.070307167235526, 51.26313993174061, 48.71706484641636, 133.85017064846414, 426.845051194539, 664.6778156996581, 503.70682593856617, 203.08566552901016, 65.07713310580208, 34.11979522184297, 27.222184300341265, 23.964505119453904, 22.612969283276428, 22.271672354948784, 21.26825938566551, 20.239249146757658, 19.199999999999974, 18.619795221842978, 17.944027303754243, 17.024232081911247, 16.10273037542661, 15.452559726962448, 15.374061433447089, 15.698293515358351, 15.713651877133096, 15.186348122866885, 25.061774744027282, 55.374061433447125, 93.50204778157007, 125.70511945392502, 138.76825938566563, 136.17098976109224, 147.41501706484652, 159.02252559726975, 120.93378839590454, 53.38771331058025, 15.978156996587021, 9.746075085324241, 10.099317406143353, 9.133447098976117, 8.058361774744036, 7.96109215017066, 7.590784982935164, 7.295563139931749, 7.986689419795232, 8.034470989761102, 7.734129692832774, 6.863822525597277, 6.491808873720145, 6.476450511945401, 5.5788395904436925, 6.172696245733797, 9.720477815699665, 22.455972696245738, 52.959385665529084, 124.11808873720142, 319.044709897611, 611.2307167235496, 751.5378839590442, 627.8774744027303, 363.30750853242324, 127.51399317406145, 22.42866894197952, 4.3843003412969335, 3.3587030716723563, 2.8808873720136523, 3.2563139931740617, 3.9269624573378863, 4.403071672354955, 3.2750853242320837, 2.548122866894196, 3.1249146757679176, 3.6163822525597284, 2.6675767918088744, 1.7494880546075087, 2.3672354948805463, 2.534470989761092, 2.614675767918089, 2.752901023890784, 2.1317406143344693, 1.6641638225255968, 1.7017064846416385, 2.2546075085324224, 2.2989761092150163, 1.935494880546075, 2.010580204778156, 2.1505119453924895, 1.5327645051194532, 1.0225255972696254, 1.5378839590443691, 1.6488054607508535, 1.406484641638226, 1.1368600682593861, 1.7665529010238905, 2.1232081911262797, 1.3740614334470993, 1.7017064846416377, 2.322866894197951, 2.1095563139931732, 1.447440273037543, 1.0634812286689426, 0.9713310580204784, 0.9798634812286693, 1.399658703071672, 0.9713310580204779, 0.6505119453924921, 1.4440273037542664, 1.2938566552901027, 0.6010238907849836, 0.3518771331058027, 0.8450511945392498, 1.3843003412969288, 0.9525597269624578, 1.1300341296928327, 1.4781569965870305, 1.0122866894197955, 0.5310580204778163, 0.20341296928327746, 0.7119453924914684, 1.476450511945393, 1.4218430034129699, 0.9116040955631408, 0.7017064846416388, 0.4593856655290104, -0.4860068259385663, -0.294880546075085, 0.8075085324232087, 0.7580204778157005, 0.7051194539249153, 0.5174061433447106, 0.4832764505119463, 1.3126279863481227, 0.906484641638225, 0.049829351535837035, 0.9098976109215019, 1.1658703071672358, -0.08327645051194416, -0.4313993174061423, -0.32901023890784903, -0.5030716723549478, 0.5498293515358366, 0.24778156996586975, -0.6771331058020477, 0.19488054607508645, 0.4747440273037553, 0.3757679180887381, 0.017406143344710523, -0.35802047781569907]
  out "On-Line  Smoothed":dbl[](array[numeric])=[15120.81331058021, 21087.279180887384, 11665.705802047789, 65.04368600682595, 92.10000000000004, 136.6477815699659, 196.36109215017063, 267.3696245733788, 344.7877133105801, 429.5095563139931, 519.963481228669, 602.557337883959, 671.6443686006826, 722.859385665529, 756.1119453924914, 768.6955631399317, 741.0931740614335, 684.3167235494881, 640.4344709897612, 626.7160409556313, 624.8935153583616, 625.637542662116, 665.3252559726963, 752.4293515358362, 805.2484641638225, 784.0880546075086, 726.6802047781568, 655.6631399317405, 569.6563139931741, 469.27406143344706, 381.9549488054605, 323.32013651877116, 289.0027303754265, 262.0692832764504, 231.95836177474393, 207.31160409556313, 187.3901023890785, 171.76552901023894, 158.29112627986348, 143.36791808873716, 130.48907849829345, 120.42423208191124, 107.96006825938571, 89.93959044368604, 71.97201365187716, 57.219453924914696, 42.700682593856655, 31.671672354948804, 28.21092150170647, 28.043686006825922, 27.176791808873702, 26.71945392491466, 27.76382252559726, 31.036860068259386, 37.079522184300345, 45.38327645051194, 53.45153583617747, 58.89180887372015, 57.51638225255975, 48.05733788395905, 34.83208191126279, 23.611945392491457, 16.714334470989755, 18.09317406143344, 35.01638225255972, 54.69897610921503, 48.593174061433466, 26.188737201365186, 14.458361774744024, 12.113651877133105, 10.553924914675767, 9.987372013651878, 25.63754266211604, 82.26552901023888, 130.81501706484636, 100.58122866894196, 42.035153583617756, 14.615358361774739, 6.658020477815699, 4.685324232081912, 5.115358361774748, 4.826962457337887, 4.350853242320821, 4.753583617747442, 4.891808873720139, 4.354266211604097, 3.5470989761092158, 3.3389078498293516, 3.581228668941981, 3.263822525597271, 2.960068259385665, 2.709215017064846, 2.6136518771331056, 2.6972696245733783, 3.016382252559727, 5.750170648464162, 11.465187713310575, 18.80307167235494, 25.980546075085314, 28.82013651877132, 26.44129692832763, 27.460068259385658, 30.122184300341296, 22.746757679180885, 10.176791808873718, 3.693856655290104, 2.0505119453924916, 1.333788395904437, 1.6273037542662117, 1.6443686006825935, 1.6221843003412966, 1.6068259385665526, 1.5078498293515352, 1.0846416382252555, 1.0812286689419794, 1.3098976109215017, 0.8645051194539253, 1.3372013651877133, 1.2194539249146754, 0.598293515358362, 0.6477815699658709, 1.6733788395904439, 4.454948805460752, 10.106825938566551, 23.719453924914678, 60.22627986348125, 112.92252559726961, 136.70921501706476, 113.79965870307163, 66.60000000000001, 23.465187713310588, 3.726279863481229, 0.6733788395904438, 0.23651877133105811, 0.11023890784982943, 0.349146757679181, 0.951535836177475, 0.4600682593856657, -0.4733788395904437, 0.588054607508533, 1.427645051194539, 1.2911262798634806, 0.8525597269624572, 1.1358361774744024, 1.5539249146757668, 1.1238907849829347, 1.1802047781569962, 0.4464163822525592, 0.14607508532423152, 1.0129692832764499, 0.804778156996587, 0.40204778156996646, 0.1819112627986353, 0.39180887372013656, 0.2211604095563143, -0.7720136518771326, -0.828327645051194, -0.19863481228668917, -0.7993174061433455, -1.0245733788395908, 0.23481228668942053, 1.0573378839590444, 0.6648464163822524, 0.9532423208191129, 1.2843003412969287, 0.6836177474402731, 0.2877133105802046, 0.24163822525597262, 0.4583617747440276, 0.5436860068259394, 0.3406143344709902, -0.08941979522184297, 0.01467576791808875, 0.5163822525597274, 0.08122866894197994, -0.3232081911262797, 0.4515358361774748, 0.27747440273037566, -0.33686006825938564, 0.016382252559726945, 1.0744027303754269, 1.454948805460751, 1.1358361774744024, 0.5965870307167236, -0.17133105802047757, 0.3627986348122866, 0.6819112627986347, 0.3047781569965875, 0.7518771331058024, 0.4156996587030717, -0.3590443686006821, -0.16450511945392426, 0.6392491467576794, -0.03481228668942016, -0.5825938566552904, -0.0023890784982933053, 0.04027303754266254, 0.057337883959044524, -0.2310580204778157, 0.0010238907849831058, -0.34197952218430006, -0.6952218430034128, -0.024573378839590557, 0.006143344709897511, -0.40511945392491444, -0.6030716723549483, -0.9034129692832762, -0.31638225255972674, 0.5726962457337886, 0.47030716723549515, 0.2433447098976111, -0.16962457337883946, -0.3010238907849825, 0.16655290102389134, 0.02320819112628028, -0.6730375426621158, 0.0010238907849831613]
  out "On-Line Bin Readings":dbl[](array[numeric])=[13265.0, 19818.0, 24045.0, 199.0, 212.0, 279.0, 329.0, 423.0, 508.0, 578.0, 667.0, 784.0, 892.0, 950.0, 1040.0, 999.0, 1023.0, 1014.0, 891.0, 834.0, 836.0, 803.0, 952.0, 1083.0, 1091.0, 1116.0, 1002.0, 837.0, 696.0, 625.0, 520.0, 499.0, 508.0, 472.0, 389.0, 410.0, 311.0, 320.0, 301.0, 306.0, 257.0, 272.0, 279.0, 254.0, 191.0, 177.0, 171.0, 175.0, 145.0, 157.0, 146.0, 165.0, 151.0, 189.0, 154.0, 187.0, 202.0, 178.0, 193.0, 174.0, 165.0, 134.0, 149.0, 156.0, 164.0, 212.0, 202.0, 143.0, 104.0, 124.0, 114.0, 121.0, 121.0, 140.0, 209.0, 309.0, 199.0, 144.0, 134.0, 129.0, 120.0, 122.0, 100.0, 132.0, 99.0, 111.0, 132.0, 126.0, 113.0, 98.0, 113.0, 111.0, 115.0, 104.0, 111.0, 108.0, 110.0, 127.0, 125.0, 154.0, 167.0, 110.0, 154.0, 153.0, 140.0, 133.0, 121.0, 134.0, 120.0, 115.0, 132.0, 109.0, 129.0, 105.0, 109.0, 114.0, 113.0, 109.0, 106.0, 124.0, 106.0, 99.0, 109.0, 110.0, 88.0, 110.0, 110.0, 117.0, 114.0, 119.0, 103.0, 108.0, 103.0, 101.0, 108.0, 116.0, 104.0, 121.0, 110.0, 117.0, 134.0, 137.0, 114.0, 117.0, 110.0, 108.0, 94.0, 131.0, 115.0, 105.0, 116.0, 94.0, 108.0, 136.0, 103.0, 114.0, 110.0, 121.0, 117.0, 129.0, 124.0, 100.0, 99.0, 106.0, 125.0, 106.0, 103.0, 108.0, 107.0, 131.0, 113.0, 87.0, 108.0, 99.0, 113.0, 109.0, 130.0, 126.0, 112.0, 116.0, 122.0, 111.0, 104.0, 110.0, 106.0, 105.0, 133.0, 97.0, 105.0, 99.0, 124.0, 120.0, 104.0, 102.0, 115.0, 118.0, 110.0, 124.0, 111.0, 88.0, 113.0, 110.0, 101.0, 100.0, 117.0, 111.0, 91.0, 113.0, 103.0, 115.0, 109.0, 121.0, 126.0, 114.0, 107.0, 130.0, 97.0, 106.0, 112.0]
  out "Range Corrected Altitude Array":dbl[](array[numeric])=[5625.0, 22500.0, 50625.0, 90000.0, 140625.0, 202500.0, 275625.0, 360000.0, 455625.0, 562500.0, 680625.0, 810000.0, 950625.0, 1102500.0, 1265625.0, 1440000.0, 1625625.0, 1822500.0, 2030625.0, 2250000.0, 2480625.0, 2722500.0, 2975625.0, 3240000.0, 3515625.0, 3802500.0, 4100625.0, 4410000.0, 4730625.0, 5062500.0, 5405625.0, 5760000.0, 6125625.0, 6502500.0, 6890625.0, 7290000.0, 7700625.0, 8122500.0, 8555625.0, 9000000.0, 9455625.0, 9922500.0, 10400625.0, 10890000.0, 11390625.0, 11902500.0, 12425625.0, 12960000.0, 13505625.0, 14062500.0, 14630625.0, 15210000.0, 15800625.0, 16402500.0, 17015625.0, 17640000.0, 18275625.0, 18922500.0, 19580625.0, 20250000.0, 20930625.0, 21622500.0, 22325625.0, 23040000.0, 23765625.0, 24502500.0, 25250625.0, 26010000.0, 26780625.0, 27562500.0, 28355625.0, 29160000.0, 29975625.0, 30802500.0, 31640625.0, 32490000.0, 33350625.0, 34222500.0, 35105625.0, 36000000.0, 36905625.0, 37822500.0, 38750625.0, 39690000.0, 40640625.0, 41602500.0, 42575625.0, 43560000.0, 44555625.0, 45562500.0, 46580625.0, 47610000.0, 48650625.0, 49702500.0, 50765625.0, 51840000.0, 52925625.0, 54022500.0, 55130625.0, 56250000.0, 57380625.0, 58522500.0, 59675625.0, 60840000.0, 62015625.0, 63202500.0, 64400625.0, 65610000.0, 66830625.0, 68062500.0, 69305625.0, 70560000.0, 71825625.0, 73102500.0, 74390625.0, 75690000.0, 77000625.0, 78322500.0, 79655625.0, 81000000.0, 82355625.0, 83722500.0, 85100625.0, 86490000.0, 87890625.0, 89302500.0, 90725625.0, 92160000.0, 93605625.0, 95062500.0, 96530625.0, 98010000.0, 99500625.0, 101002500.0, 102515625.0, 104040000.0, 105575625.0, 107122500.0, 108680625.0, 110250000.0, 111830625.0, 113422500.0, 115025625.0, 116640000.0, 118265625.0, 119902500.0, 121550625.0, 123210000.0, 124880625.0, 126562500.0, 128255625.0, 129960000.0, 131675625.0, 133402500.0, 135140625.0, 136890000.0, 138650625.0, 140422500.0, 142205625.0, 144000000.0, 145805625.0, 147622500.0, 149450625.0, 151290000.0, 153140625.0, 155002500.0, 156875625.0, 158760000.0, 160655625.0, 162562500.0, 164480625.0, 166410000.0, 168350625.0, 170302500.0, 172265625.0, 174240000.0, 176225625.0, 178222500.0, 180230625.0, 182250000.0, 184280625.0, 186322500.0, 188375625.0, 190440000.0, 192515625.0, 194602500.0, 196700625.0, 198810000.0, 200930625.0, 203062500.0, 205205625.0, 207360000.0, 209525625.0, 211702500.0, 213890625.0, 216090000.0, 218300625.0, 220522500.0, 222755625.0, 225000000.0, 227255625.0, 229522500.0, 231800625.0, 234090000.0, 236390625.0, 238702500.0, 241025625.0, 243360000.0, 245705625.0, 248062500.0, 250430625.0, 252810000.0, 255200625.0, 257602500.0, 260015625.0, 262440000.0, 264875625.0, 267322500.0, 269780625.0, 272250000.0]
  out "Altitude Array (km)":dbl[](array[numeric])=[0.075, 0.15, 0.22499999999999998, 0.3, 0.375, 0.45, 0.5249999999999999, 0.6, 0.6749999999999999, 0.7499999999999999, 0.825, 0.8999999999999999, 0.9749999999999999, 1.05, 1.125, 1.2, 1.275, 1.3499999999999999, 1.4249999999999998, 1.5, 1.575, 1.65, 1.7249999999999999, 1.7999999999999998, 1.8749999999999998, 1.95, 2.025, 2.1, 2.1750000000000003, 2.25, 2.325, 2.4, 2.475, 2.5500000000000003, 2.625, 2.7, 2.775, 2.85, 2.9250000000000003, 3.0, 3.075, 3.15, 3.225, 3.3000000000000003, 3.375, 3.45, 3.525, 3.6, 3.675, 3.75, 3.825, 3.9, 3.975, 4.05, 4.125, 4.2, 4.275, 4.35, 4.425, 4.5, 4.575, 4.65, 4.725, 4.8, 4.875, 4.95, 5.025, 5.1, 5.175, 5.25, 5.325, 5.4, 5.475, 5.55, 5.625, 5.7, 5.775, 5.85, 5.925, 6.0, 6.075, 6.15, 6.225, 6.3, 6.375, 6.45, 6.525, 6.6, 6.675, 6.75, 6.825, 6.9, 6.975, 7.05, 7.125, 7.2, 7.2749999999999995, 7.35, 7.425, 7.5, 7.575, 7.6499999999999995, 7.725, 7.8, 7.875, 7.95, 8.024999999999999, 8.1, 8.174999999999999, 8.249999999999998, 8.325, 8.399999999999999, 8.475, 8.549999999999999, 8.624999999999998, 8.7, 8.774999999999999, 8.85, 8.924999999999999, 8.999999999999998, 9.075, 9.149999999999999, 9.225, 9.299999999999999, 9.374999999999998, 9.45, 9.524999999999999, 9.6, 9.674999999999999, 9.749999999999998, 9.825, 9.899999999999999, 9.975, 10.049999999999999, 10.124999999999998, 10.2, 10.274999999999999, 10.35, 10.424999999999999, 10.499999999999998, 10.575, 10.649999999999999, 10.725, 10.799999999999999, 10.874999999999998, 10.95, 11.024999999999999, 11.1, 11.174999999999999, 11.249999999999998, 11.325, 11.399999999999999, 11.475, 11.549999999999999, 11.624999999999998, 11.7, 11.774999999999999, 11.85, 11.924999999999999, 11.999999999999998, 12.075, 12.149999999999999, 12.225, 12.299999999999999, 12.374999999999998, 12.45, 12.524999999999999, 12.6, 12.674999999999999, 12.749999999999998, 12.825, 12.899999999999999, 12.975, 13.049999999999999, 13.124999999999998, 13.2, 13.274999999999999, 13.35, 13.424999999999999, 13.499999999999998, 13.575, 13.649999999999999, 13.725, 13.799999999999999, 13.874999999999998, 13.95, 14.024999999999999, 14.1, 14.174999999999999, 14.249999999999998, 14.325, 14.399999999999999, 14.474999999999998, 14.549999999999999, 14.624999999999998, 14.7, 14.774999999999999, 14.849999999999998, 14.924999999999999, 14.999999999999998, 15.075, 15.149999999999999, 15.224999999999998, 15.299999999999999, 15.374999999999998, 15.45, 15.524999999999999, 15.599999999999998, 15.674999999999999, 15.749999999999998, 15.825, 15.899999999999999, 15.974999999999998, 16.05, 16.125, 16.2, 16.275, 16.349999999999998, 16.424999999999997, 16.5]
  out "Offline Pulse Energy":dbl=5.101813999999999
  out "Online Pulse Energy":dbl=5.089021
  in  "Instrument Control":T5(tab)
  in  "ILX Address On":dbl=1.0 min=0.0 step=1.0
  in  "ILX Address Off":dbl=2.0 min=0.0 step=1.0
  in  "OnLineLD":dbl=170.4
  in  "OffLineLD":dbl=172.55
  in  "Pulse B Polarity":enum32{"Low", "High"}(ring)=enum."High"
  in  "Pulse A Delay(ns)":u32=1040 min=80 max=327600
  in  "Pulse B Delay(ns)":u32=170000 min=80 max=327600 step=1
  in  "Accumulation Delay(ns)":u32=10 min=10 max=1270 step=1
  in  "Sync Pulse Polarity":enum32{"Low", "High"}(ring)=enum."High"
  in  "Pulse A Polarity":enum32{"Low", "High"}(ring)=enum."High"
  in  "Number of Bins":u32=220 min=2 max=4095 step=1
  in  "Number of Accumulates":u32=10000 min=1 max=32767 step=1
  in  "Time Resolution Per Bin(ns)":u32=500 min=5 max=1063 step=1
  in  "Lambda On Set (nm)":dbl=828.198 format="%.5f"
  out "Lambda On Read (nm)":dbl=828.1989571183617 format="%.5f"
  out "Lambda Off Read (nm)":dbl=828.2984734786044 format="%.5f"
  in  "Lambda Off Set (nm)":dbl=828.29765 format="%#.5f"
  in  "Bristol In":i32=5
  out "Bristol Out":i32=4
  out "AB_DIF":dbl=5e-05 format="%#_15g"
  out "NONAB_DIF":dbl=5e-05 format="%#_15g"
  out "Wavelength Lock Online":bool=TRUE
  out "Wavelength Lock Offline":bool=TRUE
  in  "calculate absorption cross sections":bool
  in  "Smoothing Range":dbl=150.0
  in  "Total DIAL Integration Time (Minutes)":i32=3
  in  "Data Reads (number of loops)":i32=1
  in  "Total Aerosol Integration Time (Minutes)":dbl=0.5
  in  "Scalar Wait Time":u32
  out "Smoothed Bins":dbl=2.0
  in  "NewportIn":string
  in  "logging":bool
  out "Newport Device Key":string="1918-C SN10503"
  in  "SampleSize":i32=2
  out "NewportRef":refnum<k24>
  in  "Switch Comm Port":refnum<visa-resource-name>="COM3"
  out "FF_On_Ref":refnum<file>
  out "FF_On_Ptr":i64=4304848 format="%.2p"
  out "FF_Off_Ref":refnum<file>
  out "FF_Off_Ptr":i64=4304848 format="%.2p"
  out "NF_On_Ref":refnum<file>
  out "NF_On_Ptr":i64=4304848 format="%.2p"
  out "NF_Off_Ref":refnum<file>
  out "NF_Off_Ptr":i64=4304848 format="%.2p"
  out "DataOpen":bool=TRUE
  out "File Path_Far Field (out)":string="E:\\Micropulse_DIAL_data\\140717FF\\23"
  out "File Path_Near Field (out)":string="E:\\Micropulse_DIAL_data\\140717NF\\23"
  in  "Data File DIR (in)":string="C:\\Users\\H2ODial\\Desktop\\SharedTeleWVData\\"
  in  "bins":u32=220 min=2 max=4095 step=1
  out "y offset":u32=10
  in  "ns scale":u32=500
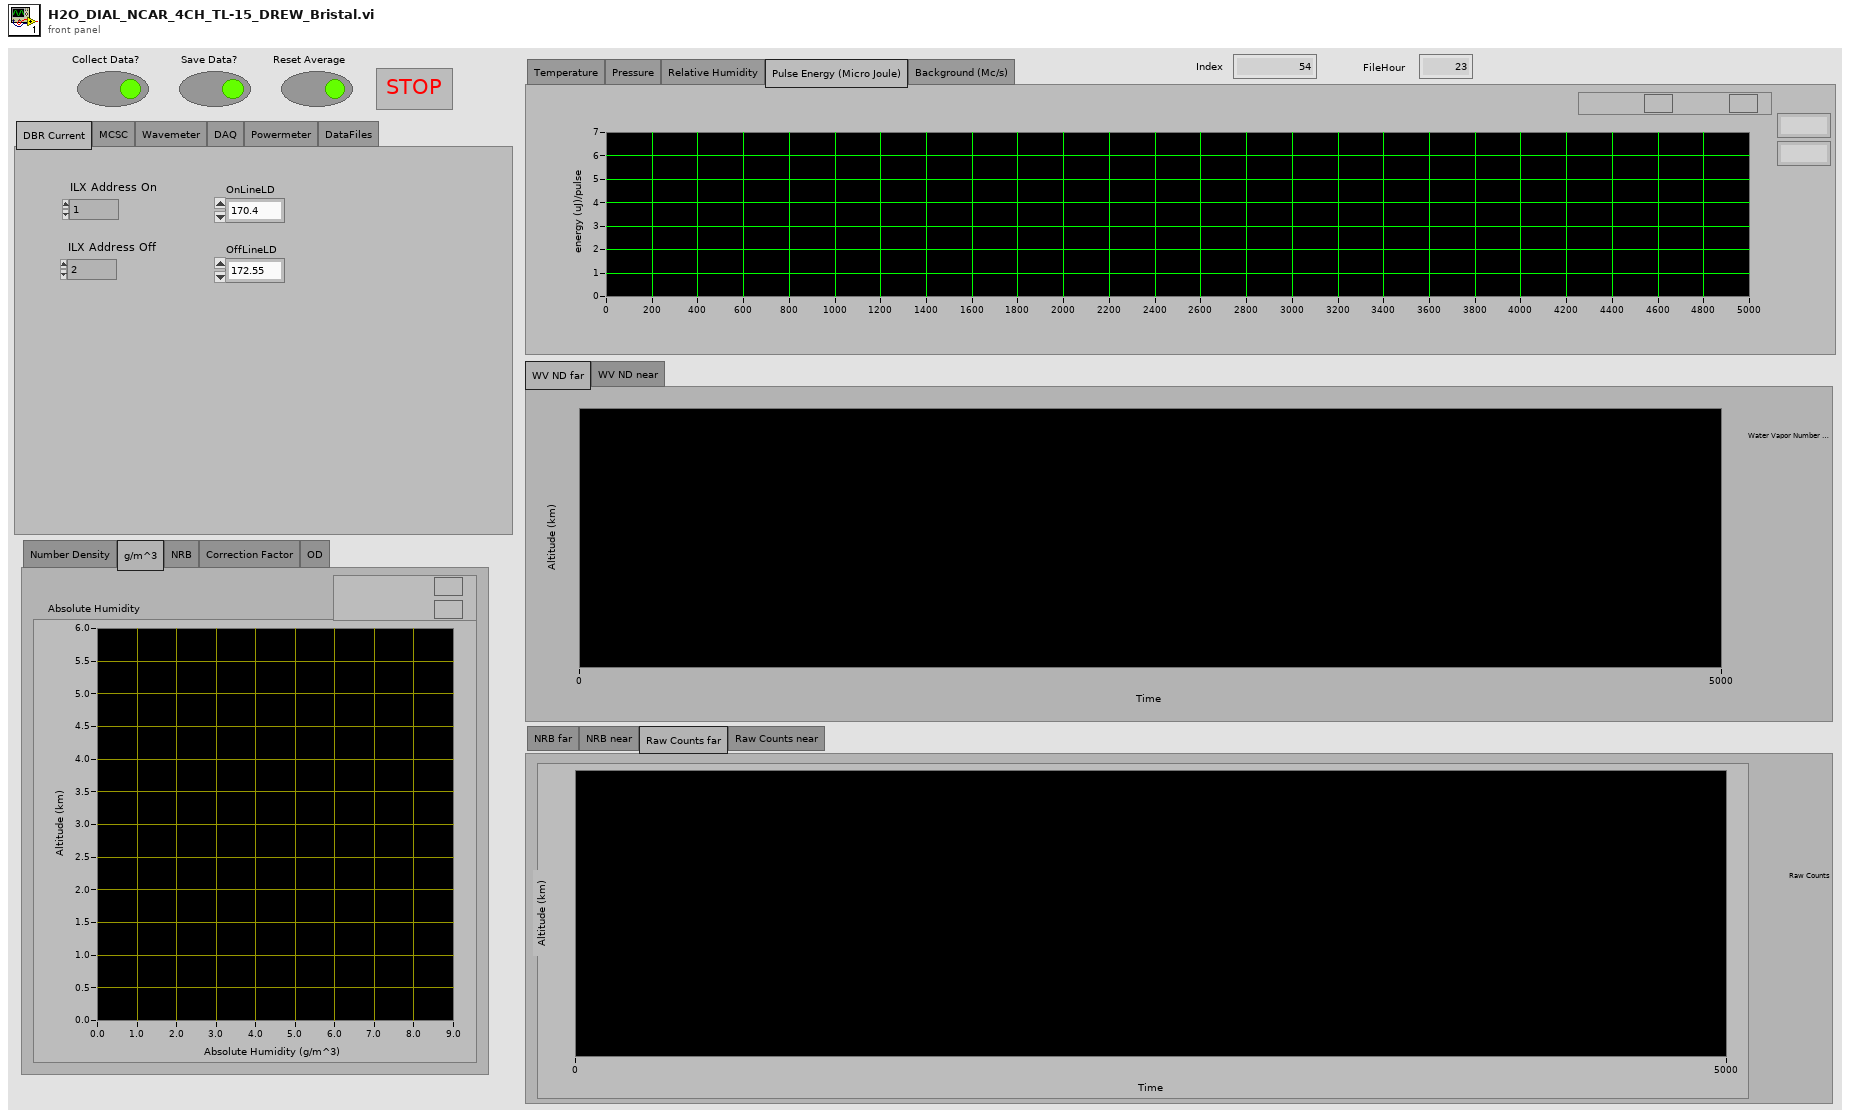
[diagram p1: front panel]
types:
  T1 = enum32{"NRB far", "NRB near", "Raw Counts far", "Raw Counts near"}
  T2 = enum32{"Number Density", "g/m^3", "NRB", "Correction Factor", "OD"}
  T3 = enum32{"Temperature", "Pressure", "Relative Humidity", "Pulse Energy (Micro Joule)", "Background (Mc/s)"}
  T4 = cluster{"Online Pulse Energy":dbl, "Pulse Energy Offline":dbl}
  T5 = enum32{"DBR Current", "MCSC", "Wavemeter", "DAQ", "Powermeter", "DataFiles"}
  T6 = enum16{"Initialize ILX", "Set ON T", "Set Off T", "Set ON I", "Set Off I", "Set On Lim", "Set Off Lim", "Read ILX", "TEC ON/OFF", "LASER ON/OFF", "Status?", "ILX OFF"}
  T7 = enum16{"open", "replace", "create", "open or create", "replace or create", "replace or create with confirmation"}
  T8 = typedef "LVDateTimeRec.ctl" = cluster{"fractional second":dbl, "second":i32, "minute":i32, "hour":i32, "day of month":i32, "month":i32, "year":i32, "day of week":i32, "day of year":i32, "DST":i32}
  T9 = cluster{"Online Pulse Energy":dbl, "Offline Pulse Energy":dbl}
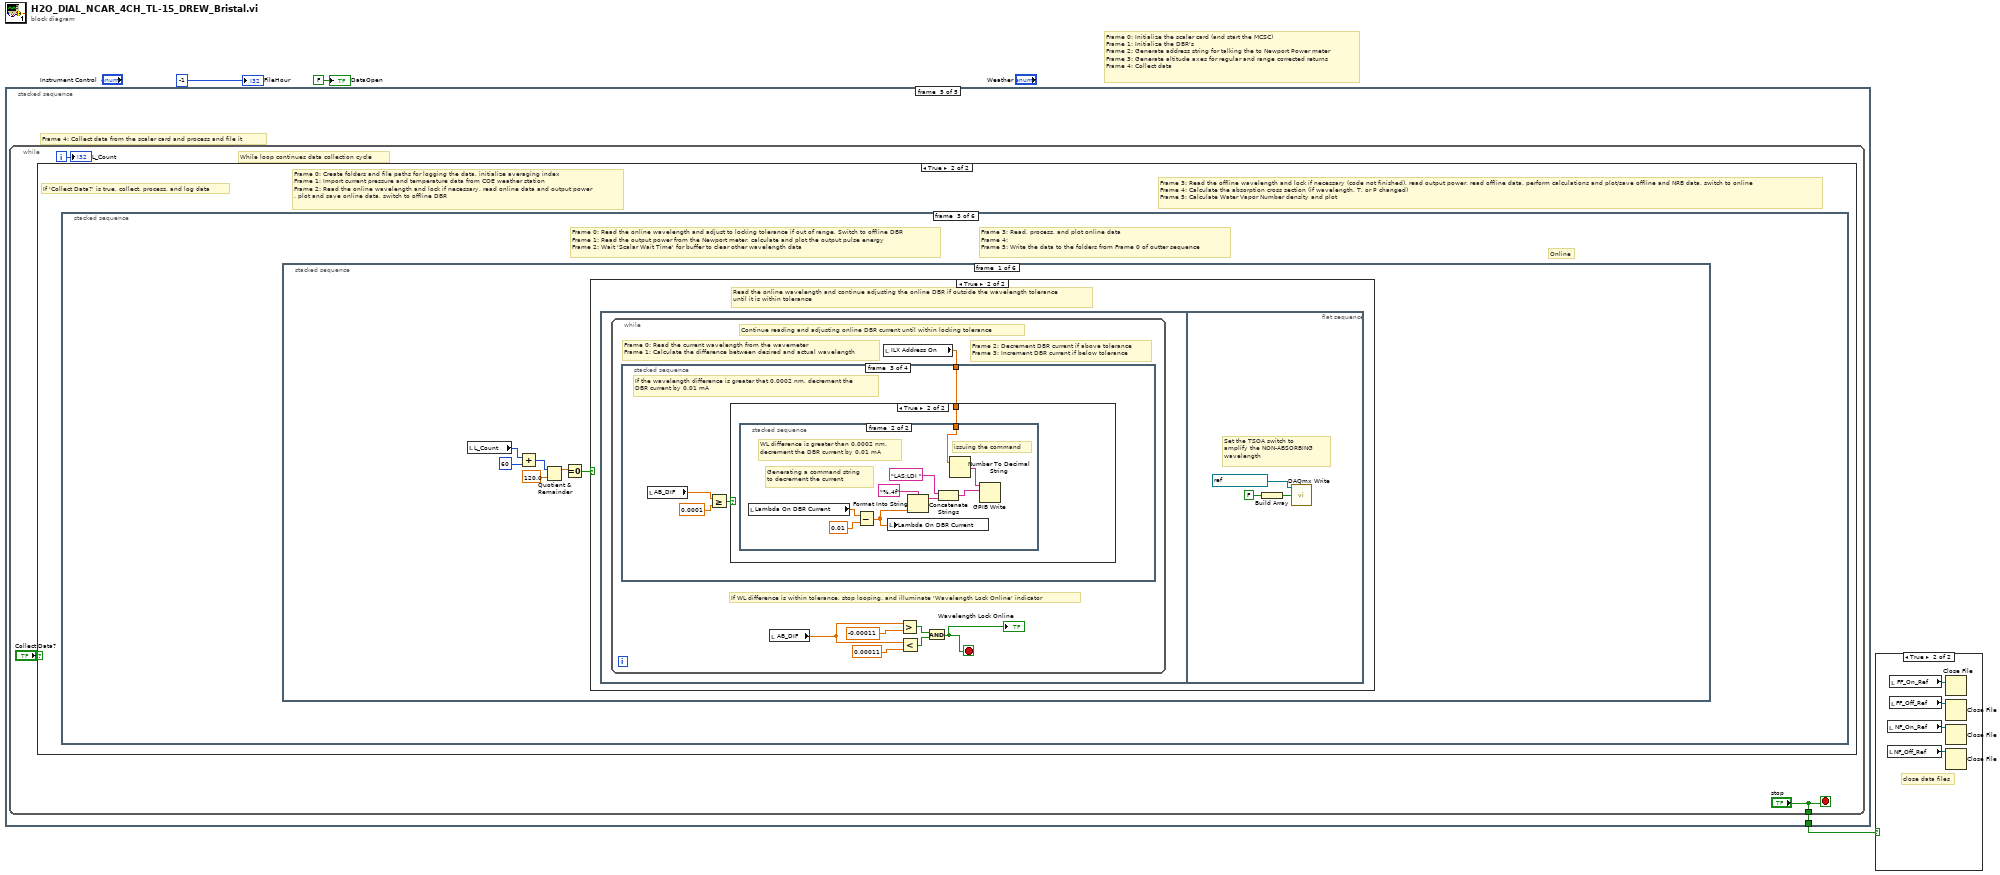
[diagram p0: block diagram]
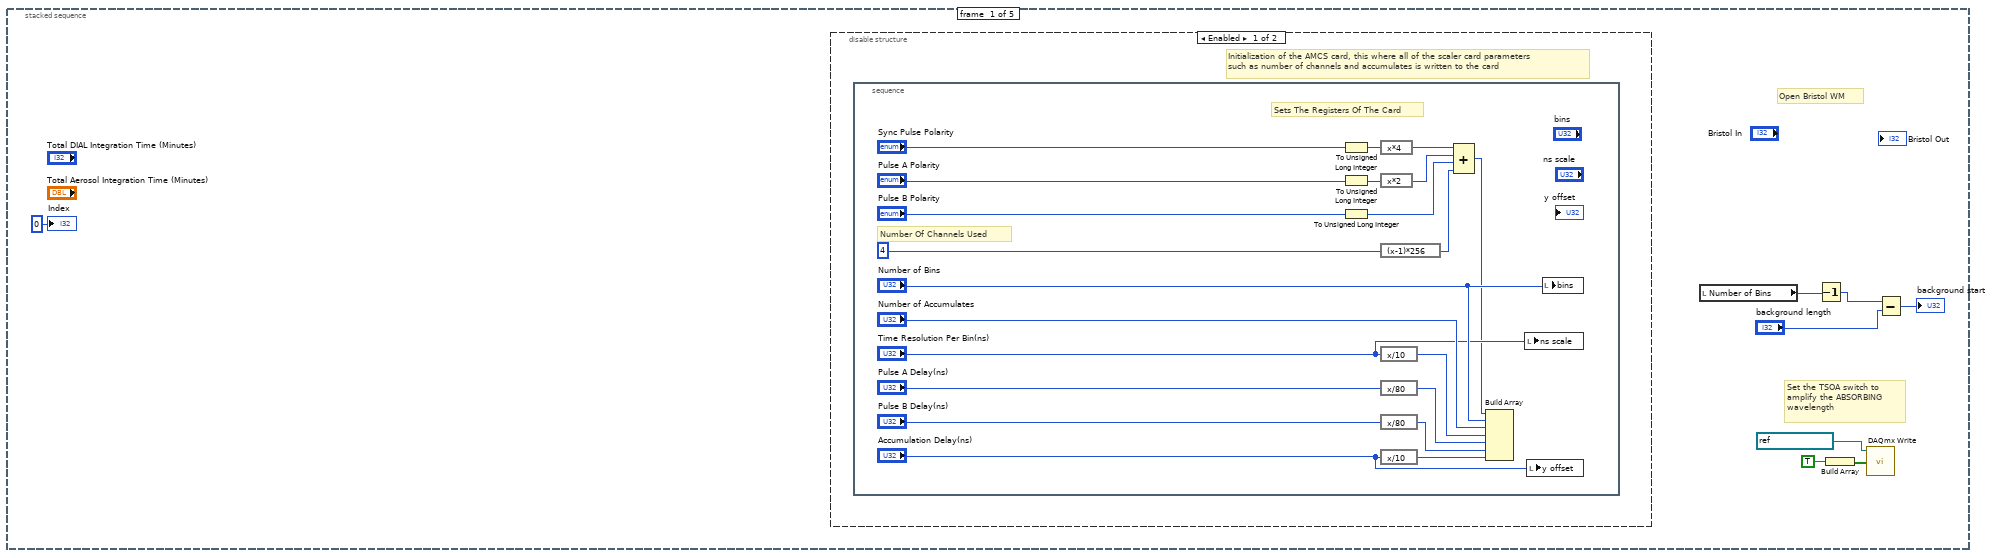
[diagram p3: hidden frame]
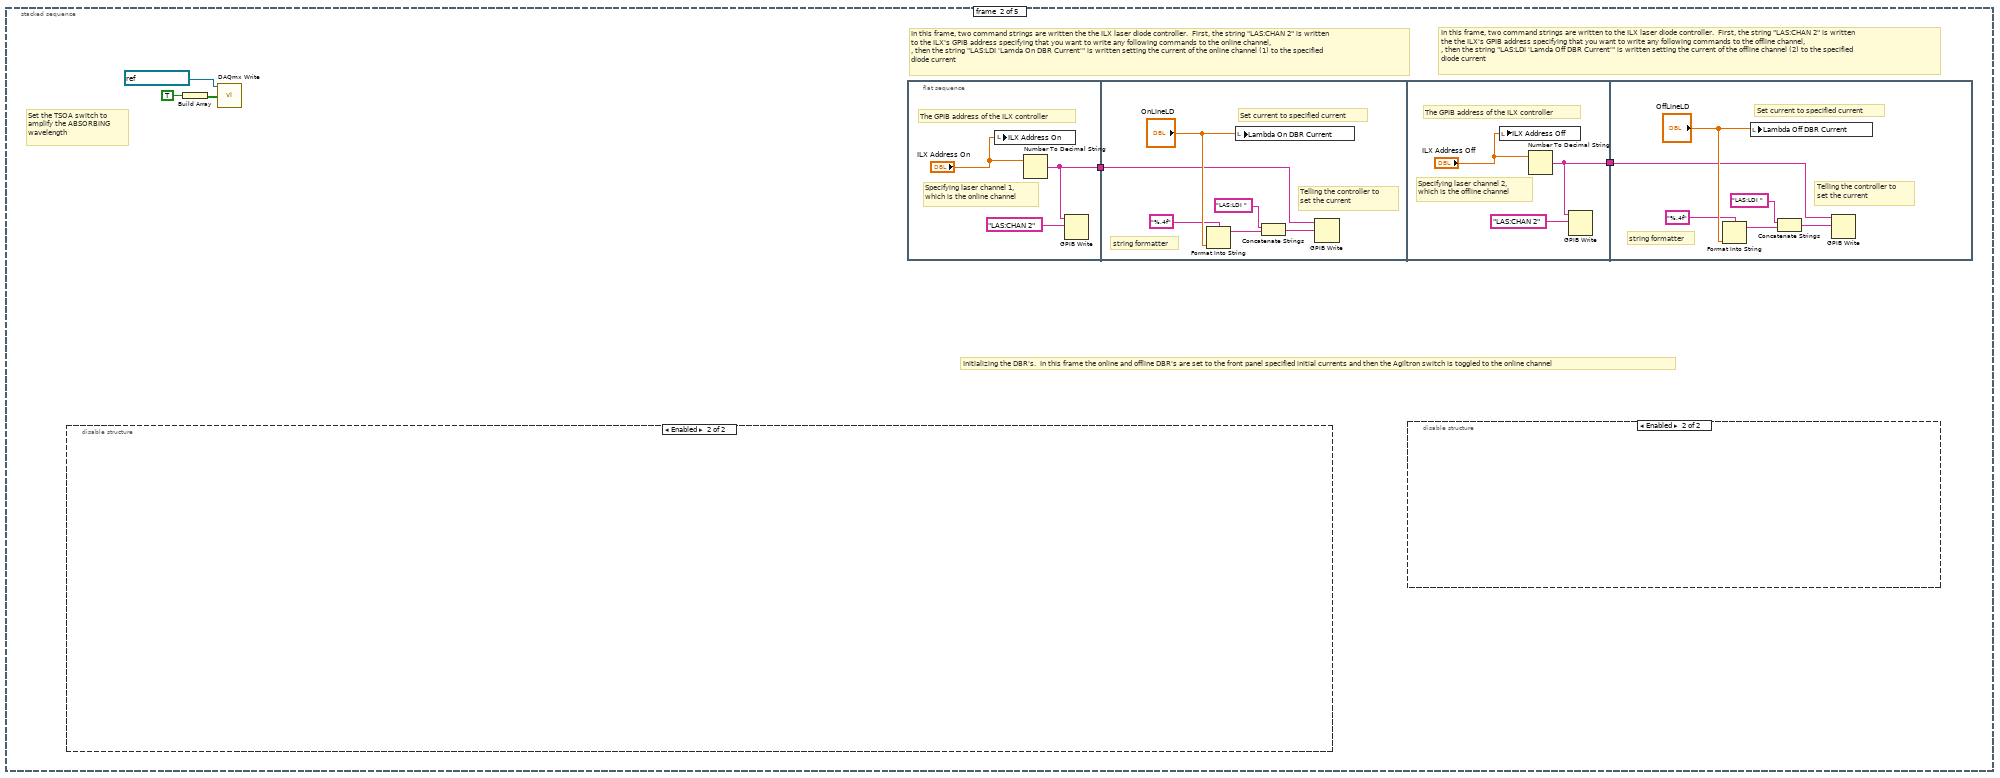
[diagram p5: hidden frame]
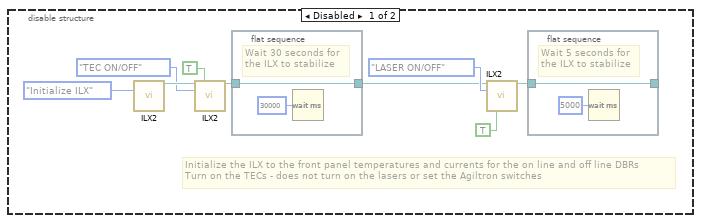
[diagram p6: hidden frame]
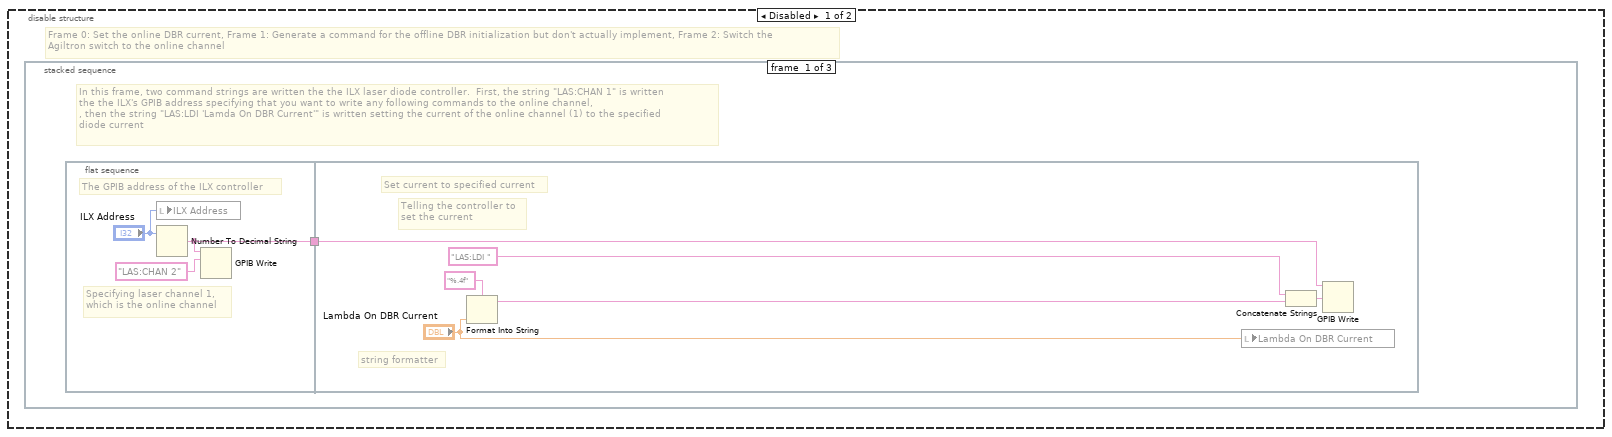
[diagram p7: hidden frame]
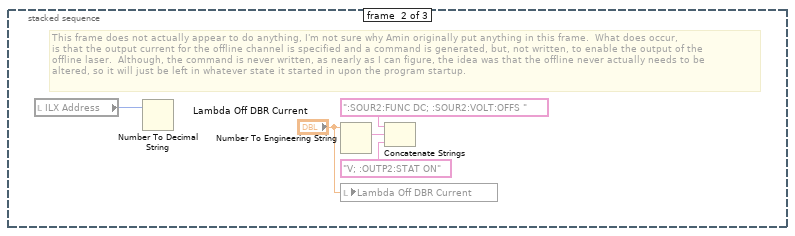
[diagram p8: hidden frame]
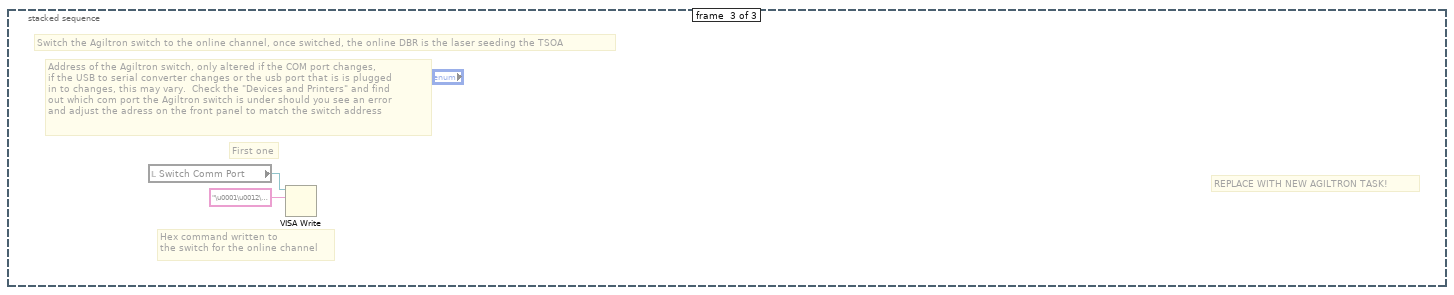
[diagram p9: hidden frame]
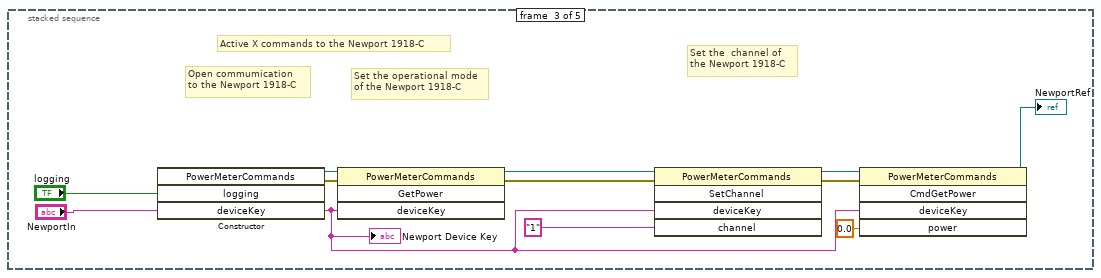
[diagram p10: hidden frame]
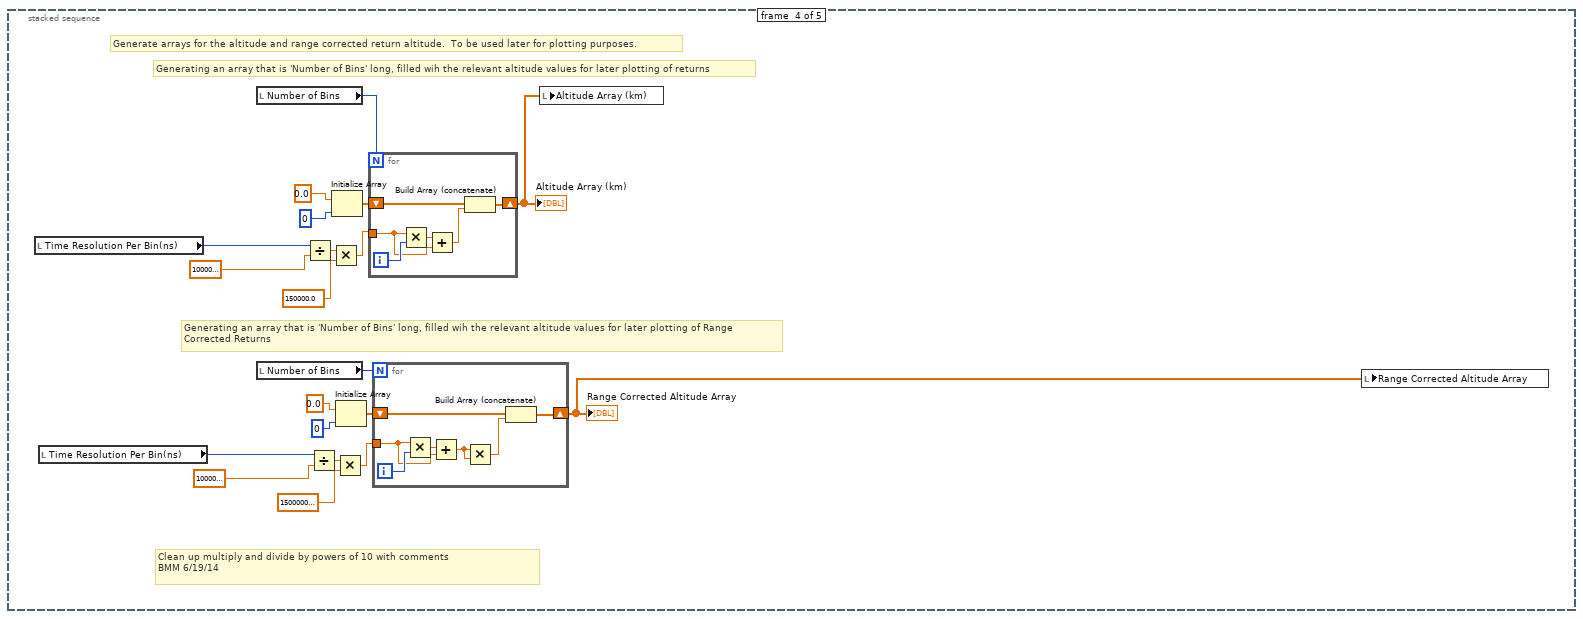
[diagram p11: hidden frame]
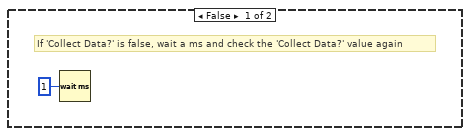
[diagram p12: hidden frame]
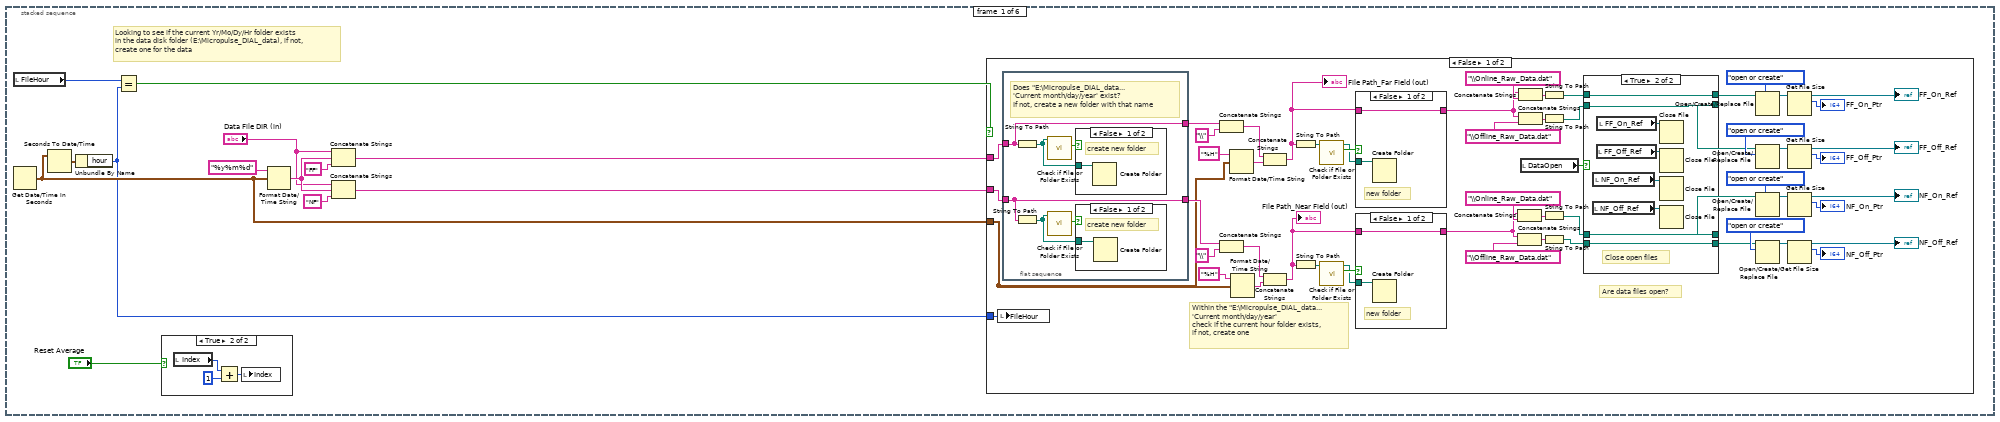
[diagram p13: hidden frame]
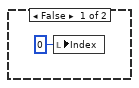
[diagram p20: hidden frame]
diagram:
  # "Frame 0: Initialize the scaler card (and start the MCSC)\nFrame 1: Initialize the DBR's\nFrame 2: Generate address string for talking the to Newport Power meter\nFrame 3: Generate altitude axes for regular and range corrected returns\nFrame 4: Collect data"
  n1 = stacked-sequence {
    tunnel: [_ _ _ _ w131] -> w3
    frame #0 {
      # "Set the TSOA switch to\namplify the ABSORBING\nwavelength"
      # "Open Bristol WM"
      n2 = disable-structure shown="Enabled" {
        frame Enabled {
          # "Initialization of the AMCS card, this where all of the scaler card parameters\nsuch as number of channels and accumulates is written to the card"
          n3 = stacked-sequence {
            frame #0 {
              # "Sets The Registers Of The Card"
              # "Number Of Channels Used"
              n4 = To Unsigned Long Integer(number="Sync Pulse Polarity") -> (unsigned 32bit integer=w12:u32)
              n5 = To Unsigned Long Integer(number="Pulse A Polarity") -> (unsigned 32bit integer=w16:u32)
              n6 = To Unsigned Long Integer(number="Pulse B Polarity") -> (unsigned 32bit integer=w14:u32)
              n7 = expression code="x*4"(w12) -> (w21:u32)
              n8 = expression code="x*2"(w16) -> (w20:u32)
              n9 = expression code="(x-1)*256"(u32 4 ("Number of Channels Used")) -> (w19:u32)
              n10 = expression code="x/10"("Time Resolution Per Bin(ns)") -> (w23:u32)
              n11 = expression code="x/80"("Pulse A Delay(ns)") -> (w30:u32)
              n12 = expression code="x/80"("Pulse B Delay(ns)") -> (w32:u32)
              n13 = expression code="x/10"("Accumulation Delay(ns)") -> (w31:u32)
              n14 = Compound Arithmetic op=ADD(w21, w20, w14, w19) -> (w18:u32)
              n15 = Build Array(w18, "Number of Bins", "Number of Accumulates", w23, w30, w32, w31) -> ()  [unwired: 1 out]
              n16 = local write "ns scale"("Time Resolution Per Bin(ns)") -> ()
              n17 = local write "y offset"("Accumulation Delay(ns)") -> ()
              n18 = local write "bins"("Number of Bins") -> ()
            }
          }
        }
        frame Disabled {
        }
      }
      n19 = local read "Number of Bins"() -> (w10:u32)
      n20 = Decrement(x=w10) -> (x-1=w9:u32)
      n21 = Build Array(TRUE ("Boolean")) -> (w6:bool[])
      n22 = call-poly <vilib>:"DAQmx Write.vi"("task/channels in"=refnum<k21> "BristolWM", "data"=w6) -> ()  [unwired: 11 in, 3 out]
      n23 = Subtract(x=w9, y="background length") -> (x-y=→"background start":u32)
      "Index" <- 0 ("Index")
    }
    frame #1 {
      # "In this frame, two command strings are written to the ILX laser diode controller.  First, the string \"LAS:CHAN 2\" is written\nthe the ILX's GPIB address specifying that you want to write any following commands to the offline channel,\n, then the string \"LAS:LDI 'Lamda Off DBR Current'\" is written setting the current of the offline channel (2) to the specified \ndiode current"
      # "In this frame, two command strings are written the the ILX laser diode controller.  First, the string \"LAS:CHAN 2\" is written\nto the ILX's GPIB address specifying that you want to write any following commands to the online channel,\n, then the string \"LAS:LDI 'Lamda On DBR Current'\" is written setting the current of the online channel (1) to the specified \ndiode current"
      # "Set the TSOA switch to\namplify the ABSORBING\nwavelength"
      # "Initializing the DBR's.  In this frame the online and offline DBR's are set to the front panel specified initial currents and then the Agiltron switch is toggled to the online channel"
      n24 = disable-structure shown="Enabled" {
        frame Disabled {
          # "Frame 0: Set the online DBR current, Frame 1: Generate a command for the offline DBR initialization but don't actually implement, Frame 2: Switch the \nAgiltron switch to the online channel"
          n25 = stacked-sequence {
            frame #0 {
              # "In this frame, two command strings are written the the ILX laser diode controller.  First, the string \"LAS:CHAN 1\" is written\nthe the ILX's GPIB address specifying that you want to write any following commands to the online channel,\n, then the string \"LAS:LDI 'Lamda On DBR Current'\" is written setting the current of the online channel (1) to the specified \ndiode current"
              n26 = flat-sequence {
                tunnel: [w71] -> w69
                tunnel: w69 -> [w73]
                frame #0 {
                  # "The GPIB address of the ILX controller"
                  # "Specifying laser channel 1,\nwhich is the online channel"
                  n27 = local write "ILX Address"("ILX Address") -> ()
                  n28 = Number To Decimal String(number="ILX Address") -> (decimal integer string=w71:string)  [unwired: 1 in]
                  n29 = GPIB Write(0:w71, 1:"LAS:CHAN 2") -> ()  [unwired: 3 in, 2 out]
                }
                frame #1 {
                  # "Telling the controller to\nset the current"
                  # "string formatter"
                  # "Set current to specified current"
                  n30 = Format Into String(format string="%.4f" ("Format String"), "Lambda On DBR Current") -> (resulting string=w76:string)  [unwired: 2 in, 1 out]
                  n31 = local write "Lambda On DBR Current"("Lambda On DBR Current") -> ()
                  n32 = Concatenate Strings("LAS:LDI ", w76) -> (w77:string)
                  n33 = GPIB Write(0:w73, 1:w77) -> ()  [unwired: 3 in, 2 out]
                }
              }
            }
            frame #1 {
              # "This frame does not actually appear to do anything, I'm not sure why Amin originally put anything in this frame.  What does occur, \nis that the output current for the offline channel is specified and a command is generated, but, not written, to enable the output of the\noffline laser.  Although, the command is never written, as nearly as I can figure, the idea was that the offline never actually needs to be \naltered, so it will just be left in whatever state it started in upon the program startup."
              n34 = local read "ILX Address"() -> (w79:i32)
              n35 = Number To Decimal String(number=w79) -> ()  [unwired: 1 in, 1 out]
              n36 = Number To Engineering String(4:"Lambda Off DBR Current") -> (0:w83:string)  [unwired: 3 in]
              n37 = local write "Lambda Off DBR Current"("Lambda Off DBR Current") -> ()
              n38 = Concatenate Strings(":SOUR2:FUNC DC; :SOUR2:VOLT:OFFS ", w83, "V; :OUTP2:STAT ON") -> ()  [unwired: 1 out]
            }
            frame #2 {
              # "REPLACE WITH NEW AGILTRON TASK!"
              # "First one"
              # "Address of the Agiltron switch, only altered if the COM port changes,\nif the USB to serial converter changes or the usb port that is is plugged\nin to changes, this may vary.  Check the \"Devices and Printers\" and find \nout which com port the Agiltron switch is under should you see an error \nand adjust the adress on the front panel to match the switch address"
              # "Hex command written to \nthe switch for the online channel"
              # "Switch the Agiltron switch to the online channel, once switched, the online DBR is the laser seeding the TSOA"
              n39 = local read "Switch Comm Port"() -> (w84:refnum<visa-resource-name>)
              n40 = VISA Write(VISA resource name=w84, write buffer="\u0001\u0012\u0000\u0002") -> ()  [unwired: 1 in, 3 out]
            }
          }
        }
        frame Enabled {
        }
      }
      n41 = Build Array(TRUE ("Boolean")) -> (w35:bool[])
      n42 = call-poly <vilib>:"DAQmx Write.vi"("task/channels in"=refnum<k21> "BristolWM", "data"=w35) -> ()  [unwired: 11 in, 3 out]
      n43 = flat-sequence {
        tunnel: [w39] -> w34
        tunnel: w34 -> [w41]
        tunnel: [w47] -> w33
        tunnel: w33 -> [w50]
        frame #0 {
          # "The GPIB address of the ILX controller"
          # "Specifying laser channel 1,\nwhich is the online channel"
          n44 = local write "ILX Address On"("ILX Address On") -> ()
          n45 = Number To Decimal String(number="ILX Address On") -> (decimal integer string=w39:string)  [unwired: 1 in]
          n46 = GPIB Write(0:w39, 1:"LAS:CHAN 2") -> ()  [unwired: 3 in, 2 out]
        }
        frame #1 {
          # "Telling the controller to\nset the current"
          # "string formatter"
          # "Set current to specified current"
          n47 = Format Into String(format string="%.4f" ("Format String"), "OnLineLD") -> (resulting string=w44:string)  [unwired: 2 in, 1 out]
          n48 = local write "Lambda On DBR Current"("OnLineLD") -> ()
          n49 = Concatenate Strings("LAS:LDI ", w44) -> (w45:string)
          n50 = GPIB Write(0:w41, 1:w45) -> ()  [unwired: 3 in, 2 out]
        }
        frame #2 {
          # "The GPIB address of the ILX controller"
          # "Specifying laser channel 2,\nwhich is the offline channel"
          n51 = local write "ILX Address Off"("ILX Address Off") -> ()
          n52 = Number To Decimal String(number="ILX Address Off") -> (decimal integer string=w47:string)  [unwired: 1 in]
          n53 = GPIB Write(0:w47, 1:"LAS:CHAN 2") -> ()  [unwired: 3 in, 2 out]
        }
        frame #3 {
          # "Telling the controller to\nset the current"
          # "string formatter"
          # "Set current to specified current"
          n54 = Format Into String(format string="%.4f" ("Format String"), "OffLineLD") -> (resulting string=w53:string)  [unwired: 2 in, 1 out]
          n55 = local write "Lambda Off DBR Current"("OffLineLD") -> ()
          n56 = Concatenate Strings("LAS:LDI ", w53) -> (w54:string)
          n57 = GPIB Write(0:w50, 1:w54) -> ()  [unwired: 3 in, 2 out]
        }
      }
      n58 = disable-structure shown="Enabled" {
        frame Disabled {
          # "Initialize the ILX to the front panel temperatures and currents for the on line and off line DBRs\nTurn on the TECs - does not turn on the lasers or set the Agiltron switches"
          n59 = call "ILX2.vi"("ILX Command"=T6."Initialize ILX") -> ("Device Out"=w63:refnum<visa-resource-name>)  [unwired: 10 in, 4 out]
          n60 = call "ILX2.vi"("Device In"=w63, "TEC Control"=TRUE, "ILX Command"=T6."TEC ON/OFF") -> ("Device Out"=w60:refnum<visa-resource-name>)  [unwired: 8 in, 4 out]
          n61 = flat-sequence {
            tunnel: w60 -> [w67]
            tunnel: [w67] -> w57
            frame #0 {
              # "Wait 30 seconds for\nthe ILX to stabilize"
              n62 = Wait (ms)(milliseconds to wait=u32 30000) -> ()  [unwired: 1 out]
            }
          }
          n63 = call "ILX2.vi"("Device In"=w57, "ILX Command"=T6."LASER ON/OFF", "Laser Control"=TRUE ("TEC Control")) -> ("Device Out"=w56:refnum<visa-resource-name>)  [unwired: 8 in, 4 out]
          n64 = flat-sequence {
            tunnel: w56 -> [w65]
            tunnel: [w65] -> _
            frame #0 {
              # "Wait 5 seconds for\nthe ILX to stabilize"
              n65 = Wait (ms)(milliseconds to wait=u32 5000) -> ()  [unwired: 1 out]
            }
          }
        }
        frame Enabled {
        }
      }
    }
    frame #2 {
      # "Active X commands to the Newport 1918-C"
      # "Set the  channel of\nthe Newport 1918-C"
      # "Set the operational mode\nof the Newport 1918-C"
      # "Open commumication\nto the Newport 1918-C"
      n66 = constructor class="PowerMeterCommands"("logging"="logging", "deviceKey"="NewportIn") -> (reference out=w97:refnum<k24>, error out=w94:errorcluster, "deviceKey"=w89:string)  [unwired: 3 in, 2 out]
      "Newport Device Key" <- w89
      n67 = invoke class="PowerMeterCommands" method="GetPower"(reference=w97, error in=w94, "deviceKey"=w89) -> (reference out=w96:refnum<k24>, error out=w93:errorcluster)  [unwired: 1 in, 2 out]
      n68 = invoke class="PowerMeterCommands" method="SetChannel"(reference=w96, error in=w93, "deviceKey"=w89, "channel"="1") -> (reference out=w90:refnum<k24>, error out=w92:errorcluster)  [unwired: 1 in, 3 out]
      n69 = invoke class="PowerMeterCommands" method="CmdGetPower"(reference=w90, error in=w92, "deviceKey"=w89, "power"=sgl 0.0) -> (reference out=→"NewportRef":refnum<k24>)  [unwired: 1 in, 4 out]
    }
    frame #3 {
      # "Clean up multiply and divide by powers of 10 with comments\nBMM 6/19/14"
      # "Generating an array that is 'Number of Bins' long, filled wih the relevant altitude values for later plotting of Range \nCorrected Returns"
      # "Generating an array that is 'Number of Bins' long, filled wih the relevant altitude values for later plotting of returns"
      # "Generate arrays for the altitude and range corrected return altitude.  To be used later for plotting purposes."
      n70 = local read "Time Resolution Per Bin(ns)"() -> (w110:u32)
      n71 = local read "Time Resolution Per Bin(ns)"() -> (w100:u32)
      n72 = local read "Number of Bins"() -> (w113:u32)
      n73 = local read "Number of Bins"() -> (w103:u32)
      n74 = Divide(x=w110, y=1000000000.0) -> (x/y=w108:dbl)
      n75 = Divide(x=w100, y=1000000000.0) -> (x/y=w98:dbl)
      n76 = Multiply(x=w108, y=150000.0) -> (x*y=w111:dbl)
      n77 = Initialize Array(0.0, 0) -> (w116:dbl[])
      n78 = Multiply(x=w98, y=150000000.0) -> (x*y=w101:dbl)
      n79 = Initialize Array(0.0, 0) -> (w106:dbl[])
      n80 = for {
        N: w113 -> [_]
        shift-right: [w129] -> w114
        shift-left: w116 -> [w130]
        tunnel: w111 -> [w126]
        i -> [w128]
        n81 = Multiply(x=w126, y=w128) -> (x*y=w127:dbl)
        n82 = Add(x=w127, y=w126) -> (x+y=w125:dbl)
        n83 = Build Array (concatenate)(w130, w125) -> (w129:dbl[])
      }
      "Altitude Array (km)" <- w114
      n84 = for {
        N: w103 -> [_]
        shift-right: [w123] -> w104
        shift-left: w106 -> [w124]
        tunnel: w101 -> [w119]
        i -> [w122]
        n85 = Multiply(x=w119, y=w122) -> (x*y=w120:dbl)
        n86 = Add(x=w120, y=w119) -> (x+y=w118:dbl)
        n87 = Multiply(x=w118, y=w118) -> (x*y=w121:dbl)
        n88 = Build Array (concatenate)(w124, w121) -> (w123:dbl[])
      }
      "Range Corrected Altitude Array" <- w104
      n89 = local write "Altitude Array (km)"(w114) -> ()
      n90 = local write "Range Corrected Altitude Array"(w104) -> ()
    }
    frame #4 {
      # "Frame 4: Collect data from the scaler card and process and file it"
      n91 = while {
        tunnel: ["stop"] -> w131
        i -> [w132]
        stop <- "stop" stop-if-true
        # "While loop continues data collection cycle"
        n92 = case shown="True" "Collect Data?" {
          frame False {
            # "If 'Collect Data?' is false, wait a ms and check the 'Collect Data?' value again"
            n93 = Wait (ms)(milliseconds to wait=u32 1) -> ()  [unwired: 1 out]
          }
          frame True {
            # "Frame 3: Read the offline wavelength and lock if necessary (code not finished), read output power, read offline data, perform calculations and plot/save offline and NRB data, switch to online\nFrame 4: Calculate the absorption cross section (if wavelength, T, or P changed)\nFrame 5: Calculate Water Vapor Number density and plot"
            # "Frame 0: Create folders and file paths for logging the data, initialize averaging index\nFrame 1: Import current pressure and temperature data from COE weather station\nFrame 2: Read the online wavelength and lock if necessary, read online data and output power\n, plot and save online data, switch to offline DBR"
            # "If 'Collect Data?' is true, collect, process, and log data"
            n94 = stacked-sequence {
              frame #0 {
                # "Looking to see if the current Yr/Mo/Dy/Hr folder exists\nin the data disk folder (E:\\Micropulse_DIAL_data), if not,\ncreate one for the data"
                n95 = local read "FileHour"() -> (w145:i32)
                n96 = Get Date/Time In Seconds() -> (seconds since 1Jan1904=w137:timestamp)
                n97 = Seconds To Date/Time(time stamp (now)=w137) -> (date time rec=w147:T8)  [unwired: 1 in]
                n98 = Unbundle By Name(w147) -> ("hour"=w136:i32)
                n99 = Equal?(x=w145, y=w136) -> (x = y?=w146:bool)
                n100 = case shown="True" "Reset Average" {
                  frame False {
                    n101 = local write "Index"(0 ("Index")) -> ()
                  }
                  frame True {
                    n102 = local read "Index"() -> (w235:i32)
                    n103 = Add(x=w235, y=1) -> (x+y=w234:i32)
                    n104 = local write "Index"(w234) -> ()
                  }
                }
                n105 = Format Date/Time String(time format string (%c)="%y%m%d", seconds (now)=w137) -> (date/time string=w141:string)  [unwired: 1 in]
                n106 = Concatenate Strings("Data File DIR (in)", w141, "FF" ("string")) -> (w143:string)
                n107 = Concatenate Strings("Data File DIR (in)", w141, "NF" ("string")) -> (w138:string)
                n108 = case shown="False" w146 {
                  tunnel: w143 -> [w205 _]
                  tunnel: w138 -> [w204 _]
                  tunnel: w137 -> [w191 _]
                  tunnel: w136 -> [w167 _]
                  frame False {
                    # "Are data files open?"
                    # "Within the \"E:\\Micropulse_DIAL_data...\n'Current month/day/year' \ncheck if the current hour folder exists,\nif not, create one"
                    n109 = local write "FileHour"(w167) -> ()
                    n110 = flat-sequence {
                      tunnel: [w225] -> w192
                      tunnel: w205 -> [w224]
                      tunnel: w204 -> [w225]
                      tunnel: [w224] -> w193
                      frame #0 {
                        # "Does \"E:\\Micropulse_DIAL_data...\n'Current month/day/year' exist?\nIf not, create a new folder with that name"
                        n111 = String To Path(string=w224) -> (path=w229:path)
                        n112 = String To Path(string=w225) -> (path=w227:path)
                        n113 = call <vilib>:"Check if File or Folder Exists.vi"("path"=w229) -> ("file or folder exists?"=w228:bool)  [unwired: 8 in, 2 out]
                        n114 = call <vilib>:"Check if File or Folder Exists.vi"("path"=w227) -> ("file or folder exists?"=w226:bool)  [unwired: 8 in, 2 out]
                        n115 = case shown="False" w228 {
                          tunnel: w229 -> [w231 _]
                          frame False {
                            # "create new folder"
                            n116 = Create Folder(path (use dialog)=w231) -> ()  [unwired: 2 in, 3 out]
                          }
                          frame True {
                            # "Folder exists\ndo nothing"
                          }
                        }
                        n117 = case shown="False" w226 {
                          tunnel: w227 -> [w230 _]
                          frame False {
                            # "create new folder"
                            n118 = Create Folder(path (use dialog)=w230) -> ()  [unwired: 2 in, 3 out]
                          }
                          frame True {
                            # "Folder exists\ndo nothing"
                          }
                        }
                      }
                    }
                    n119 = Concatenate Strings(w193, "\\" ("string")) -> (w200:string)
                    n120 = Concatenate Strings(w192, "\\" ("string")) -> (w195:string)
                    n121 = Format Date/Time String(time format string (%c)="%H", seconds (now)=w191) -> (date/time string=w203:string)  [unwired: 1 in]
                    n122 = Format Date/Time String(time format string (%c)="%H", seconds (now)=w191) -> (date/time string=w198:string)  [unwired: 1 in]
                    n123 = Concatenate Strings(w200, w203) -> (w163:string)
                    "File Path_Far Field (out)" <- w163
                    n124 = Concatenate Strings(w195, w198) -> (w164:string)
                    "File Path_Near Field (out)" <- w164
                    n125 = String To Path(string=w163) -> (path=w201:path)
                    n126 = String To Path(string=w164) -> (path=w196:path)
                    n127 = call <vilib>:"Check if File or Folder Exists.vi"("path"=w201) -> ("file or folder exists?"=w190:bool, "dup path"=w188:path)  [unwired: 8 in, 1 out]
                    n128 = call <vilib>:"Check if File or Folder Exists.vi"("path"=w196) -> ("file or folder exists?"=w189:bool, "dup path"=w187:path)  [unwired: 8 in, 1 out]
                    n129 = case shown="False" w190 {
                      tunnel: w188 -> [w222 _]
                      tunnel: w163 -> [w221 w223]
                      tunnel: [w221 w223] -> w161
                      frame False {
                        # "new folder"
                        n130 = Create Folder(path (use dialog)=w222) -> ()  [unwired: 2 in, 3 out]
                      }
                      frame True {
                        # "Folder exists\ndo nothing"
                      }
                    }
                    n131 = case shown="False" w189 {
                      tunnel: w187 -> [w219 _]
                      tunnel: w164 -> [w218 w220]
                      tunnel: [w218 w220] -> w162
                      frame False {
                        # "new folder"
                        n132 = Create Folder(path (use dialog)=w219) -> ()  [unwired: 2 in, 3 out]
                      }
                      frame True {
                        # "Folder exists\ndo nothing"
                      }
                    }
                    n133 = Concatenate Strings(w162, "\\Online_Raw_Data.dat" ("string")) -> (w181:string)
                    n134 = Concatenate Strings(w162, "\\Offline_Raw_Data.dat" ("string")) -> (w180:string)
                    n135 = Concatenate Strings(w161, "\\Online_Raw_Data.dat" ("string")) -> (w186:string)
                    n136 = Concatenate Strings(w161, "\\Offline_Raw_Data.dat" ("string")) -> (w185:string)
                    n137 = local read "DataOpen"() -> (w178:bool)
                    n138 = String To Path(string=w186) -> (path=w177:path)
                    n139 = String To Path(string=w185) -> (path=w176:path)
                    n140 = String To Path(string=w181) -> (path=w175:path)
                    n141 = String To Path(string=w180) -> (path=w174:path)
                    n142 = case shown="True" w178 {
                      tunnel: w177 -> [w209 w213]
                      tunnel: [w209 w213] -> w171
                      tunnel: w176 -> [w208 w212]
                      tunnel: [w208 w212] -> w170
                      tunnel: w175 -> [w207 w211]
                      tunnel: [w207 w211] -> w169
                      tunnel: [w206 w210] -> w168
                      tunnel: w174 -> [w206 w210]
                      frame False {
                        # "No files open\ndo nothing"
                      }
                      frame True {
                        # "Close open files"
                        n143 = local read "NF_Off_Ref"() -> (w215:refnum<file>)
                        n144 = local read "NF_On_Ref"() -> (w214:refnum<file>)
                        n145 = local read "FF_Off_Ref"() -> (w217:refnum<file>)
                        n146 = local read "FF_On_Ref"() -> (w216:refnum<file>)
                        n147 = Close File(refnum=w216) -> ()  [unwired: 1 in, 2 out]
                        n148 = Close File(refnum=w217) -> ()  [unwired: 1 in, 2 out]
                        n149 = Close File(refnum=w214) -> ()  [unwired: 1 in, 2 out]
                        n150 = Close File(refnum=w215) -> ()  [unwired: 1 in, 2 out]
                      }
                    }
                    n151 = Open/Create/Replace File(file path (use dialog)=w171, operation (0:open)=T7."open or create") -> (refnum out=w157:refnum<file>)  [unwired: 4 in, 2 out]
                    n152 = Open/Create/Replace File(file path (use dialog)=w170, operation (0:open)=T7."open or create") -> (refnum out=w158:refnum<file>)  [unwired: 4 in, 2 out]
                    n153 = Open/Create/Replace File(file path (use dialog)=w169, operation (0:open)=T7."open or create") -> (refnum out=w159:refnum<file>)  [unwired: 4 in, 2 out]
                    n154 = Open/Create/Replace File(file path (use dialog)=w168, operation (0:open)=T7."open or create") -> (refnum out=w160:refnum<file>)  [unwired: 4 in, 2 out]
                    n155 = Get File Size(file=w157) -> (refnum out=→"FF_On_Ref":refnum<file>, size (in bytes)=→"FF_On_Ptr":i64)  [unwired: 1 in, 1 out]
                    n156 = Get File Size(file=w158) -> (refnum out=→"FF_Off_Ref":refnum<file>, size (in bytes)=→"FF_Off_Ptr":i64)  [unwired: 1 in, 1 out]
                    n157 = Get File Size(file=w159) -> (refnum out=→"NF_On_Ref":refnum<file>, size (in bytes)=→"NF_On_Ptr":i64)  [unwired: 1 in, 1 out]
                    n158 = Get File Size(file=w160) -> (refnum out=→"NF_Off_Ref":refnum<file>, size (in bytes)=→"NF_Off_Ptr":i64)  [unwired: 1 in, 1 out]
                  }
                  frame True {
                    # "Don't need to do anything!"
                  }
                }
              }
              frame #1 {
                # "Writing and plotting retrieved\nweather parameters"
                # "Matlab script goes online and retrieves most recent press, temp, and relative humidity data \nfrom the weather station on the roof of Cobleigh"
                # "Importing the current weather conditions from the COE weather station"
                n159 = disable-structure shown="Disabled" {
                  frame Disabled {
                    n160 = script code="%try\n%s=urlread('http://www.coe.montana.edu/ee/weather/mostCurrentCSV.php');\n%amin=textscan(s,'%s %s %s %s %s %s %s %s %s %s %s %s %s');\n%data=amin{1}{2};\n%[test remain]=strtok(data,',');\n%remain=str2num(remain);\n%press=remain(3)./1000;\n%temp=remain(5);\n%RH=remain(7);\n%catch\npress=.850;\ntemp=20;\nRH=40;\n%end"() -> ()  [unwired: 1 in, 4 out]
                  }
                  frame Enabled {
                  }
                }
                "Temperature (C)" <- "Temperature (C)"
                "Pressure (mb)" <- "Pressure (mbar or hPa)"
                "Relative Humdity (%)" <- 40.0 ("Real")
              }
              frame #2 {
                # "Frame 3: Read, process, and plot online data\nFrame 4:\nFrame 5: Write the data to the folders from Frame 0 of outter sequence"
                # "Frame 0: Read the online wavelength and adjust to locking tolerance if out of range, Switch to offline DBR\nFrame 1: Read the output power from the Newport meter, calculate and plot the output pulse energy\nFrame 2: Wait 'Scalar Wait Time' for buffer to clear other wavelength data"
                # "Online"
                n161 = stacked-sequence {
                  frame #0 {
                    n162 = local read "L_Count"() -> (w241:i32)
                    n163 = Add(x=w241, y=60) -> (x+y=w239:i32)
                    n164 = Quotient & Remainder(x=w239, y=120.0) -> (x-y*floor(x/y)=w243:dbl)  [unwired: 1 out]
                    n165 = Equal To 0?(x=w243) -> (x = 0?=w242:bool)
                    n166 = case shown="True" w242 {
                      frame False {
                      }
                      frame True {
                        # "Read the online wavelength and continue adjusting the online DBR if outside the wavelength tolerance\nuntil it is within tolerance"
                        n167 = flat-sequence {
                          frame #0 {
                            n168 = while {
                              stop <- w245 stop-if-true
                              # "If WL difference is within tolerance, stop looping, and illuminate 'Wavelength Lock Online' indicator"
                              # "Frame 2: Decrement DBR current if above tolerance\nFrame 3: Increment DBR current if below tolerance"
                              # "Frame 0: Read the current wavelength from the wavemeter\nFrame 1: Calculate the difference between desired and actual wavelength"
                              # "Continue reading and adjusting online DBR current until within locking tolerance"
                              n169 = local read "AB_DIF"() -> (w248:dbl)
                              n170 = local read "ILX Address On"() -> (w246:dbl)
                              n171 = stacked-sequence {
                                tunnel: w246 -> [_ _ w260 w277]
                                frame #0 {
                                # "Reading the wavelength from the wavemeter"
                                n172 = flat-sequence {
                                frame #0 {
                                n173 = local read "Bristol In"() -> (w253:i32)
                                n174 = dll-call lib="C:/Users/H2ODial/Desktop/Shared Telescope WV DIAL Code/Libraries and VIs/CLDevIface.dll" fn="CLOpenUSBSerialDevice"("commPort"=w253) -> ("return type"=w252:i32)  [unwired: 4 in, 2 out]
                                n175 = local write "Bristol Out"(w252) -> ()
                                }
                                frame #1 {
                                n176 = local read "Bristol Out"() -> (w254:i32)
                                n177 = dll-call lib="C:/Users/H2ODial/Desktop/Shared Telescope WV DIAL Code/Libraries and VIs/CLDevIface.dll" fn="CLGetLambdaReading"("devHandle"=w254) -> ("return type"=→"Lambda On Read (nm)":dbl)  [unwired: 4 in, 2 out]
                                }
                                frame #2 {
                                n178 = local read "Bristol Out"() -> (w256:i32)
                                n179 = dll-call lib="C:/Users/H2ODial/Desktop/Shared Telescope WV DIAL Code/Libraries and VIs/CLDevIface.dll" fn="CLCloseDevice"("devHandle"=w256) -> ()  [unwired: 5 in, 2 out]
                                }
                                }
                                }
                                frame #1 {
                                # "Calculating the difference between the actual and desired online wavelength"
                                n180 = local read "Lambda On Read (nm)"() -> (w259:dbl)
                                n181 = Subtract(x=w259, y="Lambda On Set (nm)") -> (x-y=→"AB_DIF":dbl)
                                }
                                frame #2 {
                                # "If the wavelength difference is greater that 0.0002 nm, decrement the \nDBR current by 0.01 mA"
                                n182 = local read "AB_DIF"() -> (w263:dbl)
                                n183 = Greater Or Equal?(x=w263, y=0.0001) -> (x >= y?=w261:bool)
                                n184 = case shown="True" w261 {
                                tunnel: w260 -> [_ w264]
                                frame False {
                                # "Wavelength difference is not greater than 0.0002 nm, do nothing"
                                }
                                frame True {
                                n185 = stacked-sequence {
                                tunnel: w264 -> [w265 w268]
                                frame #0 {
                                # "Specifying laser channel 1,\nwhich is the online channel"
                                n186 = Number To Decimal String(number=w265) -> (decimal integer string=w266:string)  [unwired: 1 in]
                                n187 = GPIB Write(0:w266, 1:"LAS:CHAN 2") -> ()  [unwired: 3 in, 2 out]
                                }
                                frame #1 {
                                # "issuing the command"
                                # "Generating a command string\nto decrement the current"
                                # "WL difference is greater than 0.0002 nm,\ndecrement the DBR current by 0.01 mA"
                                n188 = local read "Lambda On DBR Current"() -> (w275:dbl)
                                n189 = Subtract(x=w275, y=0.01) -> (x-y=w269:dbl)
                                n190 = local write "Lambda On DBR Current"(w269) -> ()
                                n191 = Format Into String(format string="%.4f" ("Format String"), w269) -> (resulting string=w272:string)  [unwired: 2 in, 1 out]
                                n192 = Concatenate Strings("LAS:LDI ", w272) -> (w271:string)
                                n193 = Number To Decimal String(number=w268) -> (decimal integer string=w270:string)  [unwired: 1 in]
                                n194 = GPIB Write(0:w270, 1:w271) -> ()  [unwired: 3 in, 2 out]
                                }
                                }
                                }
                                }
                                }
                                frame #3 {
                                # "If WL difference is < 0.0002 nm, increment the DBR current"
                                n195 = local read "AB_DIF"() -> (w280:dbl)
                                n196 = Less Or Equal?(x=w280, y=-0.0001) -> (x <= y?=w278:bool)
                                n197 = case shown="True" w278 {
                                tunnel: w277 -> [_ w281]
                                frame False {
                                # "WL difference is no <= to -0.0002 nm, do nothing"
                                }
                                frame True {
                                n198 = stacked-sequence {
                                tunnel: w281 -> [w283 w285]
                                frame #0 {
                                # "Specifying laser channel 1,\nwhich is the online channel"
                                n199 = Number To Decimal String(number=w283) -> (decimal integer string=w282:string)  [unwired: 1 in]
                                n200 = GPIB Write(0:w282, 1:"LAS:CHAN 2") -> ()  [unwired: 3 in, 2 out]
                                }
                                frame #1 {
                                # "issuing the command"
                                # "Generating a command \nstring to increment the current"
                                # "WL difference is < -0.0002,\nincrement the DBR current by 0.01 mA"
                                n201 = local read "Lambda On DBR Current"() -> (w292:dbl)
                                n202 = Add(x=w292, y=0.01) -> (x+y=w287:dbl)
                                n203 = local write "Lambda On DBR Current"(w287) -> ()
                                n204 = Format Into String(format string="%.4f" ("Format String"), w287) -> (resulting string=w289:string)  [unwired: 2 in, 1 out]
                                n205 = Concatenate Strings("LAS:LDI ", w289) -> (w288:string)
                                n206 = Number To Decimal String(number=w285) -> (decimal integer string=w286:string)  [unwired: 1 in]
                                n207 = GPIB Write(0:w286, 1:w288) -> ()  [unwired: 3 in, 2 out]
                                }
                                }
                                }
                                }
                                }
                              }
                              n208 = Greater?(x=w248, y=-0.00011) -> (0:w250:bool)
                              n209 = Less?(x=w248, y=0.00011) -> (x < y?=w249:bool)
                              n210 = And(x=w250, y=w249) -> (x .and. y?=w245:bool)
                              "Wavelength Lock Online" <- w245
                            }
                          }
                          frame #1 {
                            # "Set the TSOA switch to\namplify the NON-ABSORBING\nwavelength"
                            n211 = Build Array(FALSE ("Boolean")) -> (w294:bool[])
                            n212 = call-poly <vilib>:"DAQmx Write.vi"("task/channels in"=refnum<k21> "BristolWM", "data"=w294) -> ()  [unwired: 11 in, 3 out]
                          }
                        }
                      }
                    }
                  }
                  frame #1 {
                    # "Converting to pulse energy, assumes 5 percent pickoff"
                    # "Reading the Newport Power meter"
                    # "Reading the output power of the laser transmitter from the Newport power meter, once read, convert to corresponding pulse energy and plot"
                    n213 = local read "Newport Device Key"() -> (w301:string)
                    n214 = local read "NewportRef"() -> (w297:refnum<k24>)
                    n215 = disable-structure shown="Disabled" {
                      frame Disabled {
                        # "Plotting the online and offling pulse energies"
                        n216 = local read "Online Pulse Energy"() -> (w312:dbl)
                        n217 = local read "Offline Pulse Energy"() -> (w311:dbl)
                        n218 = Bundle("Online Pulse Energy"=w312, "Offline Pulse Energy"=w311) -> (→"Pulse Energy (Micro Joule)":T9)  [unwired: 1 in]
                      }
                      frame Enabled {
                      }
                    }
                    n219 = Number To Decimal String(number="SampleSize") -> (decimal integer string=w299:string)  [unwired: 1 in]
                    n220 = invoke class="PowerMeterCommands" method="PerformDAQ"(reference=w297, "deviceKey"=w301, "interval"="1", "sampleSize"=w299) -> ("PerformDAQ"=w302:dbl[])  [unwired: 2 in, 5 out]
                    n221 = call-poly <vilib>:"Mean.vi"("X"=w302) -> ("mean"=w300:dbl)  [unwired: 1 out]
                    n222 = Multiply(x=w300, y=1000.0) -> (x*y=w308:dbl)
                    n223 = Divide(x=w308, y=0.05) -> (x/y=w306:dbl)
                    n224 = Divide(x=w306, y=10.0) -> (x/y=→"Online Pulse Energy":dbl)
                  }
                  frame #2 {
                    # "Waiting 'Scalar Wait Time'"
                    # "Wait 'Scalar Wait Time' for the next available batch of scalar card data"
                    n225 = Wait (ms)(milliseconds to wait="Scalar Wait Time") -> ()  [unwired: 1 out]
                  }
                  frame #3 {
                    # "convert time per range bin to meters\nand calculate smoothed bins using\nsmoothing range"
                    # "Plotting online cross section and smoothed online data"
                    # "Calculate the bin by bin mean of the data"
                    # "Collect 'Integration Period (Seconds)' number\nof scalar data"
                    # "Reading, processing, and plotting the online data"
                    n226 = local read "Data Reads (number of loops)"() -> (w339:i32)
                    n227 = for {
                      N: w339 -> [_]
                      tunnel: [w360] -> w351 mode=indexing
                      tunnel: [w359] -> w314 mode=indexing
                      # "Scalar Data is retrieved from Global \nVariable that scaler.vi is writing to,"
                      n228 = global read "Scalar_Data.vi" "Scalar Data"() -> (w360:u16[])
                      n229 = global read "Scalar_Data_3.vi" "Scalar Data 3"() -> (w359:u16[])
                    }
                    n230 = Transpose 2D Array(2D array=w351) -> (transposed array=w355:u16[][])
                    n231 = Transpose 2D Array(2D array=w314) -> (transposed array=w337:u16[][])
                    n232 = for {
                      tunnel: w355 -> [w362] mode=indexing
                      tunnel: [w361] -> w356 mode=indexing
                      n233 = call-poly <vilib>:"Mean.vi"("X"=w362) -> ("mean"=w361:dbl)  [unwired: 1 out]
                    }
                    n234 = for {
                      tunnel: w337 -> [w358] mode=indexing
                      tunnel: [w357] -> w338 mode=indexing
                      n235 = call-poly <vilib>:"Mean.vi"("X"=w358) -> ("mean"=w357:dbl)  [unwired: 1 out]
                    }
                    n236 = local read "bins"() -> (w331:u32)
                    n237 = Array Subset(array=w356, index=1 ("dimension size"), length=w331) -> (w343:dbl[])
                    n238 = Array Subset(array=w338, index=1 ("dimension size"), length=w331) -> (w335:dbl[])
                    n239 = local read "background length"() -> (w321:i32)
                    n240 = local read "background start"() -> (w322:u32)
                    n241 = Array Size(array=w343) -> (size(s)=w340:i32)
                    n242 = Array Size(array=w335) -> (size(s)=w332:i32)
                    n243 = Initialize Array(1.0 ("element"), w340) -> (w342:dbl[])
                    n244 = Initialize Array(1.0 ("element"), w332) -> (w334:dbl[])
                    n245 = Multiply(x=w343, y=w342) -> (x*y=w344:dbl[])
                    "On-Line Bin Readings" <- w344
                    n246 = Multiply(x=w335, y=w334) -> (x*y=w325:dbl[])
                    "On-Line Bin Readings 2" <- w325
                    n247 = local read "Total DIAL Integration Time (Minutes)"() -> (w347:i32)
                    n248 = local read "Time Resolution Per Bin(ns)"() -> (w317:u32)
                    n249 = Array Subset(array=w344, index=w322, length=w321) -> (w353:dbl[])
                    n250 = Array Subset(array=w325, index=w322, length=w321) -> (w327:dbl[])
                    n251 = call-poly <vilib>:"Mean.vi"("X"=w353) -> ("mean"=w352:dbl)  [unwired: 1 out]
                    n252 = call-poly <vilib>:"Mean.vi"("X"=w327) -> ("mean"=w328:dbl)  [unwired: 1 out]
                    n253 = Divide(x=w347, y=w339) -> (x/y=w345:dbl)
                    n254 = local read "Index"() -> (w326:i32)
                    n255 = Subtract(x=w344, y=w352) -> (x-y=w349:dbl[])
                    n256 = Subtract(x=w325, y=w328) -> (x-y=w329:dbl[])
                    n257 = To Double Precision Float(number=w317) -> (double precision float=w318:dbl)
                    n258 = Multiply(x=w345, y=60.0) -> (x*y=w323:dbl)
                    n259 = Multiply(x=w318, y=0.15) -> (x*y=w320:dbl)
                    n260 = call "Ring Buffer Online Far.vi"("Index"=w326, "Profiles to Average"=w323, "Input Array"=w349) -> ("AvgArray"=w348:dbl[])  [unwired: 7 in, 1 out]
                    n261 = call "Ring Buffer Online Near.vi"("Index"=w326, "Profiles to Average"=w323, "Input Array"=w329) -> ("AvgArray"=w330:dbl[])  [unwired: 7 in, 1 out]
                    n262 = Divide(x="Smoothing Range", y=w320) -> (x/y=w315:dbl)
                    "Smoothed Bins" <- w315
                    n263 = call "Smooth Arrray.vi"("smooth size"=w315, "Raw Array"=w348) -> ("Smoothed Array"=→"On-Line  Smoothed":dbl[])  [unwired: 9 in]
                    n264 = call "Smooth Arrray.vi"("smooth size"=w315, "Raw Array"=w330) -> ("Smoothed Array"=→"On-Line Smoothed 2":dbl[])  [unwired: 9 in]
                    n265 = disable-structure shown="Disabled" {
                      frame Disabled {
                        n266 = script code="format long;\ncounts=sum(Online);\nif counts >=0.5e6\ntime=time;\nelse\ntime=time\nend"() -> ()  [unwired: 3 in, 2 out]
                      }
                      frame Enabled {
                      }
                    }
                  }
                  frame #4 {
                    # "Toggling the Agiltron switch to the offline DBR seed laser"
                    n267 = disable-structure shown="Disabled" {
                      frame Disabled {
                        n268 = flat-sequence {
                          frame #0 {
                            # "Second one"
                            # "Command the switch to switch to position 2\ncorresponding to the offline DBR"
                            # "Hex string command \ncorrespond to offline"
                            n269 = VISA Write(VISA resource name="Switch Comm Port", write buffer="\u0001\u0012\u0000\u0001") -> ()  [unwired: 1 in, 3 out]
                          }
                        }
                      }
                      frame Enabled {
                      }
                    }
                  }
                  frame #5 {
                    # "Save the recently collected online data if 'Save Data?' is true"
                    n270 = case shown="True" "Save Data?" {
                      frame False {
                        # "'Save Data?' is false, do nothing"
                      }
                      frame True {
                        # "'Save Data?' is true, save onfline data to the Data Disk"
                        # "Write only one copy of data at this time"
                        # "Retrieve Julian Date"
                        n271 = local read "Lambda On DBR Current"() -> (w390:dbl)
                        n272 = local read "Lambda On Read (nm)"() -> (w391:dbl)
                        n273 = local read "On-Line Bin Readings 2"() -> (w385:dbl[])
                        n274 = local read "Relative Humdity (%)"() -> (w386:dbl)
                        n275 = local read "On-Line Bin Readings"() -> (w393:dbl[])
                        n276 = local read "Online Pulse Energy"() -> (w389:dbl)
                        n277 = local read "Temperature (C)"() -> (w388:dbl)
                        n278 = local read "Pressure (mb)"() -> (w387:dbl)
                        n279 = call "Julian_Date_2.vi"() -> ("Julian Date"=w392:dbl)  [unwired: 11 in]
                        n280 = Build Array (concatenate)(w392, w391, w390, w389, w388, w387, w386, w393) -> (w380:dbl[])
                        n281 = Build Array (concatenate)(w392, w391, w390, w389, w388, w387, w386, w385) -> (w370:dbl[])
                        n282 = local write "DataOpen"(TRUE ("DataOpen")) -> ()
                        n283 = local read "NF_On_Ref"() -> (w368:refnum<file>)
                        n284 = local read "FF_On_Ref"() -> (w384:refnum<file>)
                        n285 = local read "NF_On_Ptr"() -> (w369:i64)
                        n286 = local read "FF_On_Ptr"() -> (w383:i64)
                        n287 = Set File Position(offset (in bytes) (0)=w383, refnum=w384) -> (refnum out=w381:refnum<file>, error out=w378:errorcluster)  [unwired: 2 in]
                        n288 = Set File Position(offset (in bytes) (0)=w369, refnum=w368) -> (refnum out=w374:refnum<file>, error out=w372:errorcluster)  [unwired: 2 in]
                        n289 = Write to Binary File(file (use dialog)=w374, data=w370, error in=w372, 5:FALSE ("prepend array or string size? (T)")) -> (refnum out=w373:refnum<file>, error out=w371:errorcluster)  [unwired: 2 in, 1 out]
                        n290 = Write to Binary File(file (use dialog)=w381, data=w380, error in=w378, 5:FALSE ("prepend array or string size? (T)")) -> (refnum out=w379:refnum<file>, error out=w377:errorcluster)  [unwired: 2 in, 1 out]
                        n291 = Get File Position(4:w371, 7:w373) -> (2:w367:i64)  [unwired: 2 out]
                        n292 = Get File Position(4:w377, 7:w379) -> (2:w376:i64)  [unwired: 2 out]
                        n293 = local write "NF_On_Ptr"(w367) -> ()
                        n294 = local write "FF_On_Ptr"(w376) -> ()
                      }
                    }
                  }
                }
              }
              frame #3 {
                # "Frame 3: Read offline data, calculate aerosol data, and plot offline and normalized relative backscatter\nFrame 4:\nFrame 5: Save the offline data and related information"
                # "Frame 0: Read the offline wavelength and lock if necessary, Switch to online DBR\nFrame 1: Read the output power from the Newport power meter\nFrame 2: Wait 'Scalar Wait Time' for buffers to clear of online contiminated data"
                # "offline"
                n295 = stacked-sequence {
                  frame #0 {
                    # "Every 60 data collection cycles, read the offline DBR wavelength, and if outside of wavelength tolerance, adjust DBR current until within tolerance"
                    n296 = local read "L_Count"() -> (w395:i32)
                    n297 = Quotient & Remainder(x=w395, y=120.0) -> (x-y*floor(x/y)=w396:dbl)  [unwired: 1 out]
                    n298 = Equal To 0?(x=w396) -> (x = 0?=w394:bool)
                    n299 = case shown="True" w394 {
                      frame False {
                      }
                      frame True {
                        n300 = flat-sequence {
                          frame #0 {
                            n301 = while {
                              stop <- w398 stop-if-true
                              # "If WL difference is within tolerance, stop looping, and illuminate 'Wavelength Lock Offline' indicator"
                              # "Frame 2: Decrement DBR current if above tolerance\nFrame 3: Increment DBR current if below tolerance"
                              # "Frame 0: Read the current wavelength from the wavemeter\nFrame 1: Calculate the difference between desired and actual wavelength"
                              # "Continue reading and adjusting offline DBR current until within locking tolerance"
                              n302 = local read "NONAB_DIF"() -> (w401:dbl)
                              n303 = local read "ILX Address Off"() -> (w399:dbl)
                              n304 = stacked-sequence {
                                tunnel: w399 -> [_ _ w413 w430]
                                frame #0 {
                                # "Reading the wavelength from the wavemeter"
                                n305 = flat-sequence {
                                frame #0 {
                                n306 = local read "Bristol In"() -> (w406:i32)
                                n307 = dll-call lib="C:/Users/H2ODial/Desktop/Shared Telescope WV DIAL Code/Libraries and VIs/CLDevIface.dll" fn="CLOpenUSBSerialDevice"("commPort"=w406) -> ("return type"=w405:i32)  [unwired: 4 in, 2 out]
                                n308 = local write "Bristol Out"(w405) -> ()
                                }
                                frame #1 {
                                n309 = local read "Bristol Out"() -> (w408:i32)
                                n310 = dll-call lib="C:/Users/H2ODial/Desktop/Shared Telescope WV DIAL Code/Libraries and VIs/CLDevIface.dll" fn="CLGetLambdaReading"("devHandle"=w408) -> ("return type"=→"Lambda Off Read (nm)":dbl)  [unwired: 4 in, 2 out]
                                }
                                frame #2 {
                                n311 = local read "Bristol Out"() -> (w409:i32)
                                n312 = dll-call lib="C:/Users/H2ODial/Desktop/Shared Telescope WV DIAL Code/Libraries and VIs/CLDevIface.dll" fn="CLCloseDevice"("commPort"=w409) -> ()  [unwired: 5 in, 2 out]
                                }
                                }
                                }
                                frame #1 {
                                # "Calculating the difference between the actual and desired online wavelength"
                                n313 = local read "Lambda Off Read (nm)"() -> (w412:dbl)
                                n314 = Subtract(x=w412, y="Lambda Off Set (nm)") -> (x-y=→"NONAB_DIF":dbl)
                                }
                                frame #2 {
                                # "If the wavelength difference is greater that 0.0002 nm, decrement the \nDBR current by 0.01 mA"
                                n315 = local read "NONAB_DIF"() -> (w416:dbl)
                                n316 = Greater Or Equal?(x=w416, y=0.0001) -> (x >= y?=w414:bool)
                                n317 = case shown="True" w414 {
                                tunnel: w413 -> [_ w417]
                                frame False {
                                # "Wavelength difference is not greater than 0.0002 nm, do nothing"
                                }
                                frame True {
                                n318 = stacked-sequence {
                                tunnel: w417 -> [w418 w421]
                                frame #0 {
                                # "Specifying laser channel 1,\nwhich is the online channel"
                                n319 = Number To Decimal String(number=w418) -> (decimal integer string=w419:string)  [unwired: 1 in]
                                n320 = GPIB Write(0:w419, 1:"LAS:CHAN 2") -> ()  [unwired: 3 in, 2 out]
                                }
                                frame #1 {
                                # "issuing the command"
                                # "Generating a command string\nto decrement the current"
                                # "WL difference is greater than 0.0002 nm,\ndecrement the DBR current by 0.01 mA"
                                n321 = local read "Lambda Off DBR Current"() -> (w428:dbl)
                                n322 = Subtract(x=w428, y=0.01) -> (x-y=w422:dbl)
                                n323 = local write "Lambda Off DBR Current"(w422) -> ()
                                n324 = Format Into String(format string="%.4f" ("Format String"), w422) -> (resulting string=w425:string)  [unwired: 2 in, 1 out]
                                n325 = Concatenate Strings("LAS:LDI ", w425) -> (w424:string)
                                n326 = Number To Decimal String(number=w421) -> (decimal integer string=w423:string)  [unwired: 1 in]
                                n327 = GPIB Write(0:w423, 1:w424) -> ()  [unwired: 3 in, 2 out]
                                }
                                }
                                }
                                }
                                }
                                frame #3 {
                                # "If WL difference is < 0.0002 nm, increment the DBR current"
                                n328 = local read "NONAB_DIF"() -> (w433:dbl)
                                n329 = Less Or Equal?(x=w433, y=-0.0001) -> (x <= y?=w431:bool)
                                n330 = case shown="True" w431 {
                                tunnel: w430 -> [_ w434]
                                frame False {
                                # "WL difference is no <= to -0.0002 nm, do nothing"
                                }
                                frame True {
                                n331 = stacked-sequence {
                                tunnel: w434 -> [w436 w438]
                                frame #0 {
                                # "Specifying laser channel 1,\nwhich is the online channel"
                                n332 = Number To Decimal String(number=w436) -> (decimal integer string=w435:string)  [unwired: 1 in]
                                n333 = GPIB Write(0:w435, 1:"LAS:CHAN 2") -> ()  [unwired: 3 in, 2 out]
                                }
                                frame #1 {
                                # "issuing the command"
                                # "Generating a command \nstring to increment the current"
                                # "WL difference is < -0.0002,\nincrement the DBR current by 0.01 mA"
                                n334 = local read "Lambda Off DBR Current"() -> (w445:dbl)
                                n335 = Add(x=w445, y=0.01) -> (x+y=w440:dbl)
                                n336 = local write "Lambda Off DBR Current"(w440) -> ()
                                n337 = Format Into String(format string="%.4f" ("Format String"), w440) -> (resulting string=w442:string)  [unwired: 2 in, 1 out]
                                n338 = Concatenate Strings("LAS:LDI ", w442) -> (w441:string)
                                n339 = Number To Decimal String(number=w438) -> (decimal integer string=w439:string)  [unwired: 1 in]
                                n340 = GPIB Write(0:w439, 1:w441) -> ()  [unwired: 3 in, 2 out]
                                }
                                }
                                }
                                }
                                }
                              }
                              n341 = Greater?(x=w401, y=-0.00011) -> (0:w403:bool)
                              n342 = Less?(x=w401, y=0.00011) -> (x < y?=w402:bool)
                              n343 = And(x=w403, y=w402) -> (x .and. y?=w398:bool)
                              "Wavelength Lock Offline" <- w398
                            }
                          }
                          frame #1 {
                            # "Set the TSOA switch to\namplify the ABSORBING\nwavelength"
                            n344 = Build Array(TRUE ("Boolean")) -> (w449:bool[])
                            n345 = call-poly <vilib>:"DAQmx Write.vi"("task/channels in"=refnum<k21> "BristolWM", "data"=w449) -> ()  [unwired: 11 in, 3 out]
                          }
                        }
                      }
                    }
                  }
                  frame #1 {
                    # "Reading the power meter"
                    # "Updating the pulse energy plot"
                    # "Converting to pulse energy"
                    # "Reading the offline output power, converting to pulse energy,  and updating the Pulse energy plot"
                    n346 = local read "SampleSize"() -> (w452:i32)
                    n347 = local read "Newport Device Key"() -> (w453:string)
                    n348 = local read "Online Pulse Energy"() -> (w459:dbl)
                    n349 = local read "Offline Pulse Energy"() -> (w458:dbl)
                    n350 = local read "NewportRef"() -> (w450:refnum<k24>)
                    n351 = Number To Decimal String(number=w452) -> (decimal integer string=w454:string)  [unwired: 1 in]
                    n352 = invoke class="PowerMeterCommands" method="PerformDAQ"(reference=w450, "deviceKey"=w453, "interval"="1", "sampleSize"=w454) -> ("PerformDAQ"=w455:dbl[])  [unwired: 2 in, 5 out]
                    n353 = Bundle("Online Pulse Energy"=w459, "Offline Pulse Energy"=w458) -> (w457:T9)  [unwired: 1 in]
                    n354 = local write "Pulse Energy (Micro Joule)"(w457) -> ()
                    n355 = call-poly <vilib>:"Mean.vi"("X"=w455) -> ("mean"=w451:dbl)  [unwired: 1 out]
                    n356 = Multiply(x=w451, y=1000.0) -> (x*y=w464:dbl)
                    n357 = Divide(x=w464, y=0.05) -> (x/y=w462:dbl)
                    n358 = Divide(x=w462, y=10.0) -> (x/y=→"Offline Pulse Energy":dbl)
                  }
                  frame #2 {
                    # "Wait 'Scalar Wait Time' for buffers to clear of online contiminated offline data"
                    n359 = disable-structure shown="Disabled" {
                      frame Disabled {
                        # "Wait 'Scalar Wait Time'"
                        n360 = local read "Scalar Wait Time"() -> (w466:u32)
                        n361 = Wait (ms)(milliseconds to wait=w466) -> ()  [unwired: 1 out]
                      }
                      frame Enabled {
                      }
                    }
                  }
                  frame #3 {
                    w500 = 1 ("dimension size")
                    w504 = 1
                    # "Plotting the normalized relative \nbackscatter"
                    # "Calculating the normalized relative backscatter"
                    # "Calculating/Plotting smoothed data,\ncross sections etc."
                    # "Pick off data with\nout header"
                    # "Calculate mean bin by bin mean"
                    # "Reading in 'Integration Period (Seconds)' of data"
                    # "Read the offline data from the scalar card, perform smoothing, calculate normalized relative backscatter, and plot"
                    # "File path in MATLAB script is of old dial is:\nF:\\Micropulse DIAL\\Micropulse DIAL Matlab\\\nFinal Overlap Function.mat')];"
                    # "Collects Data From Card,\nSends It To The Chart,\nAnd Saves A Copy As A\nFile If Option Selected On\nFront Panel"
                    n362 = for {
                      N: "Data Reads (number of loops)" -> [_]
                      tunnel: [w536] -> w468 mode=indexing
                      tunnel: [w535] -> w467 mode=indexing
                      # "Read in latest scalar card data from \n'Scalar Data' global variable that \nscaler.vi is writing to, then wait 1 sec\nfor next batch of data"
                      n363 = global read "Scalar_Data_2.vi" "Scalar Data 2"() -> (w536:u16[])
                      n364 = global read "Scalar_Data_4.vi" "Scalar Data 4"() -> (w535:u16[])
                    }
                    n365 = local read "Total DIAL Integration Time (Minutes)"() -> (w525:i32)
                    n366 = Divide(x=w525, y="Data Reads (number of loops)") -> (x/y=w523:dbl)
                    n367 = local read "Total Aerosol Integration Time (Minutes)"() -> (w527:dbl)
                    n368 = local read "background length"() -> (w472:i32)
                    n369 = Multiply(x=w523, y=60.0) -> (x*y=w510:dbl)
                    n370 = local read "background start"() -> (w473:u32)
                    n371 = Transpose 2D Array(2D array=w468) -> (transposed array=w533:u16[][])
                    n372 = Transpose 2D Array(2D array=w467) -> (transposed array=w516:u16[][])
                    n373 = Divide(x=w527, y="Data Reads (number of loops)") -> (x/y=w528:dbl)
                    n374 = for {
                      tunnel: w533 -> [w540] mode=indexing
                      tunnel: [w539] -> w534 mode=indexing
                      tunnel: w516 -> [w538] mode=indexing
                      tunnel: [w537] -> _ mode=indexing
                      tunnel: [w537] -> w513 mode=indexing
                      n375 = call-poly <vilib>:"Mean.vi"("X"=w540) -> ("mean"=w539:dbl)  [unwired: 1 out]
                      n376 = call-poly <vilib>:"Mean.vi"("X"=w538) -> ("mean"=w537:dbl)  [unwired: 1 out]
                    }
                    n377 = local read "bins"() -> (w501:u32)
                    n378 = Multiply(x=w528, y=60.0) -> (x*y=w491:dbl)
                    n379 = Array Subset(array=w513, index=w500, length=w501) -> (w514:dbl[])
                    "Off-Line Bin Readings 2" <- w514
                    n380 = Array Subset(array=w534, index=w500, length=w501) -> (w512:dbl[])
                    "Off-Line  Bin Readings" <- w512
                    n381 = Array Subset(array=w514, index=w473, length=w472) -> (w515:dbl[])
                    n382 = Array Subset(array=w512, index=w473, length=w472) -> (w532:dbl[])
                    n383 = local read "Smoothed Bins"() -> (w469:dbl)
                    n384 = call-poly <vilib>:"Mean.vi"("X"=w515) -> ("mean"=w479:dbl)  [unwired: 1 out]
                    n385 = call-poly <vilib>:"Mean.vi"("X"=w532) -> ("mean"=w480:dbl)  [unwired: 1 out]
                    n386 = local read "Index"() -> (w490:i32)
                    n387 = Subtract(x=w514, y=w479) -> (x-y=w492:dbl[])
                    n388 = Subtract(x=w512, y=w480) -> (x-y=w508:dbl[])
                    n389 = call "Ring Buffer Offline Far.vi"("Index"=w490, "Profiles to Average"=w510, "Input Array"=w508) -> ("AvgArray"=w530:dbl[], "RingBufferOut"=→"RingBuffer offline far":dbl[][])  [unwired: 7 in]
                    n390 = call "Ring Buffer Aerosol Far.vi"("Index"=w490, "Profiles to Average"=w491, "Input Array"=w508) -> ("AvgArray"=w526:dbl[], "RingBufferOut"=→"RingBuffer aerosol far":dbl[][])  [unwired: 7 in]
                    n391 = call "Ring Buffer Offline Near.vi"("Index"=w490, "Profiles to Average"=w510, "Input Array"=w492) -> ("AvgArray"=w511:dbl[], "RingBufferOut"=→"RingBuffer offline near":dbl[][])  [unwired: 7 in]
                    n392 = call "Ring Buffer Aerosol Near.vi"("Index"=w490, "Profiles to Average"=w491, "Input Array"=w492) -> ("AvgArray"=w488:dbl[], "RingBufferOut"=→"RingBuffer aerosol near":dbl[][])  [unwired: 7 in]
                    n393 = Reshape Array(w508, w500, w501) -> (→"raw counts":dbl[][])
                    n394 = Reshape Array(w492, w500, w501) -> (→"raw counts near":dbl[][])
                    n395 = call "Smooth Arrray.vi"("smooth size"=w469, "Raw Array"=w530) -> ("Smoothed Array"=→"Off-Line Smoothed":dbl[])  [unwired: 9 in]
                    n396 = call "Smooth Arrray.vi"("smooth size"=w469, "Raw Array"=w526) -> ("Smoothed Array"=w499:dbl[])  [unwired: 9 in]
                    "Aerosol Smoothed" <- w499
                    n397 = call "Smooth Arrray.vi"("smooth size"=w469, "Raw Array"=w511) -> ("Smoothed Array"=→"Off-Line Smoothed 2":dbl[])  [unwired: 9 in]
                    n398 = call "Smooth Arrray.vi"("smooth size"=w469, "Raw Array"=w488) -> ("Smoothed Array"=w471:dbl[])  [unwired: 9 in]
                    "Aerosol Smoothed 2" <- w471
                    n399 = local read "Number of Accumulates"() -> (w475:u32)
                    n400 = local read "Temperature (C)"() -> (w522:dbl)
                    n401 = local read "Pressure (mb)"() -> (w521:dbl)
                    n402 = script code="%accum_num=10000;     % scaler card setting number of accumulations\nt_bin = 500e-9                 % scaler card setting time per bin\n%t_d = 37.3e-9;                % APD dead time from spec sheet\n\n% conversion from accumulated counts to count rate  (c/s)\nc_convert = 1./t_bin./accum_num;\nCR_far = p_raw_far.*c_convert;\nCR_near = p_raw_near.*c_convert;\nCR_total_far = (p_raw_far+b_far).*c_convert;\nCR_total_near = (p_raw_near+b_near).*c_convert;\nb_CR_far =b_far.*c_convert;\nb_CR_near =b_near.*c_convert;\n\n% create a range array\nsize_p =  size(p_raw_far,2);\nr = (75:75:size_p*75)./1e3; \n    \n%APD correction factor\n D_far = 1./(1-(t_d*CR_total_far));\n D_near = 1./(1-(t_d*CR_total_near));\n\n %Calculating normalize relative backscatter profile\n nrb_far = CR_far.*D_far.*r.^2./E.*1e-6;\n nrb_near = CR_near.*D_near.*r.^2./E.*1e-6;"("E"=6.0 ("Real"), "temp"=w522, "press"=w521, "p_raw_far"=w499, "b_far"=w480, "b_near"=w479, "p_raw_near"=w471, "accum_num"=w475, "t_d"="dead time") -> ("nrb_far"=w494:cdb[], "D_far"=w485:dbl[], "nrb_near"=w493:cdb[], "D_near"=w484:dbl[], "b_CR_far"=w477:dbl, "b_CR_near"=w476:dbl)  [unwired: 1 in, 1 out]
                    n403 = local read "bins"() -> (w503:u32)
                    n404 = local read "Altitude Array (km)"() -> (w496:dbl[])
                    n405 = Bundle(w477, w476) -> (→"?":cluster{dbl, dbl})  [unwired: 1 in]
                    n406 = Build Array(w494, w493) -> (w498:cdb[][])
                    n407 = Build Array(w485, w484) -> (w483:dbl[][])
                    n408 = Reshape Array(w493, w504, w503) -> (→"NRB 2":cdb[][])
                    n409 = Reshape Array(w494, w504, w503) -> (→"NRB":cdb[][])
                    n410 = Build Array(w496, w496) -> (w495:dbl[][])
                    n411 = call "Convert to Dynamic Data7"("2D Array"=w483) -> ("Dynamic Data Type"=w482:dynamicdata)  [unwired: 3 in]
                    n412 = call "Convert to Dynamic Data3"("2D Array"=w498) -> ("Dynamic Data Type"=w497:dynamicdata)  [unwired: 3 in]
                    n413 = call "Convert to Dynamic Data4"("2D Array"=w495) -> ("Dynamic Data Type"=w486:dynamicdata)  [unwired: 3 in]
                    n414 = call "Build XY Graph2"("Y Input"=w486, "X Input"=w497) -> ("XY Graph"=→"NRB plot":cluster{"Y":dbl[], "Y":dbl[]}[])  [unwired: 3 in, 6 out]
                    n415 = call "Build XY Graph4"("Y Input"=w486, "X Input"=w482) -> ("XY Graph"=→"Correction":cluster{"Y":dbl[], "Y":dbl[]}[])  [unwired: 3 in, 6 out]
                  }
                  frame #4 {
                    # "REPLACE WITH NEW AGILTRON TASK!"
                    # "Toggle Agiltron switch to online DBR"
                    n416 = disable-structure shown="Disabled" {
                      frame Disabled {
                        # "ABSORBING"
                        n417 = flat-sequence {
                          frame #0 {
                            # "Third one"
                            # "Command the switch to switch to position 1\ncorresponding to the online DBR"
                            # "Hex string command \ncorrespond to online"
                            n418 = local read "Switch Comm Port"() -> (w544:refnum<visa-resource-name>)
                            n419 = VISA Write(VISA resource name=w544, write buffer="\u0001\u0012\u0000\u0002") -> ()  [unwired: 1 in, 3 out]
                          }
                        }
                        n420 = Build Array(FALSE ("Boolean")) -> (w543:bool[])
                        n421 = call-poly <vilib>:"DAQmx Write.vi"("task/channels in"=refnum<k21> "AgiltronSwitch", "data"=w543) -> ()  [unwired: 11 in, 3 out]
                      }
                      frame Enabled {
                      }
                    }
                  }
                  frame #5 {
                    # "If 'Save Data?' is true, save all relavant offline info"
                    n422 = local read "Save Data?"() -> (w546:bool)
                    n423 = case shown="True" w546 {
                      frame False {
                        # "'Save Data?' is false, do nothing"
                      }
                      frame True {
                        # "Write only one data file at this time"
                        # "Retrive Julian Date"
                        # "'Save Data?' is true, save offline data to the Data Disk"
                        n424 = local read "Lambda Off DBR Current"() -> (w568:dbl)
                        n425 = local read "Off-Line Bin Readings 2"() -> (w565:dbl[])
                        n426 = local read "Lambda Off Read (nm)"() -> (w567:dbl)
                        n427 = local read "Off-Line  Bin Readings"() -> (w573:dbl[])
                        n428 = local read "Relative Humdity (%)"() -> (w572:dbl)
                        n429 = local read "Offline Pulse Energy"() -> (w569:dbl)
                        n430 = local read "Temperature (C)"() -> (w570:dbl)
                        n431 = local read "Pressure (mb)"() -> (w571:dbl)
                        n432 = call "Julian_Date_2.vi"() -> ("Julian Date"=w566:dbl)  [unwired: 11 in]
                        n433 = Build Array (concatenate)(w566, w567, w568, w569, w570, w571, w572, w573) -> (w551:dbl[])
                        n434 = Build Array (concatenate)(w566, w567, w568, w569, w570, w571, w572, w565) -> (w548:dbl[])
                        n435 = local read "FF_Off_Ref"() -> (w553:refnum<file>)
                        n436 = local read "NF_Off_Ref"() -> (w550:refnum<file>)
                        n437 = local read "FF_Off_Ptr"() -> (w552:i64)
                        n438 = local read "NF_Off_Ptr"() -> (w549:i64)
                        n439 = Set File Position(offset (in bytes) (0)=w552, refnum=w553) -> (refnum out=w564:refnum<file>, error out=w562:errorcluster)  [unwired: 2 in]
                        n440 = Set File Position(offset (in bytes) (0)=w549, refnum=w550) -> (refnum out=w560:refnum<file>, error out=w558:errorcluster)  [unwired: 2 in]
                        n441 = Write to Binary File(file (use dialog)=w564, data=w551, error in=w562, 5:FALSE ("prepend array or string size? (T)")) -> (refnum out=w563:refnum<file>, error out=w561:errorcluster)  [unwired: 2 in, 1 out]
                        n442 = Write to Binary File(file (use dialog)=w560, data=w548, error in=w558, 5:FALSE ("prepend array or string size? (T)")) -> (refnum out=w559:refnum<file>, error out=w557:errorcluster)  [unwired: 2 in, 1 out]
                        n443 = Get File Position(4:w561, 7:w563) -> (2:w554:i64)  [unwired: 2 out]
                        n444 = Get File Position(4:w557, 7:w559) -> (2:w547:i64)  [unwired: 2 out]
                        n445 = local write "FF_Off_Ptr"(w554) -> ()
                        n446 = local write "NF_Off_Ptr"(w547) -> ()
                      }
                    }
                  }
                }
              }
              frame #4 {
                n447 = First Call?() -> (First Call?: T/F=w576:bool)
                n448 = Or(x="calculate absorption cross sections", y=w576) -> (x .or. y?=w574:bool)
                n449 = case shown="True" w574 {
                  frame False {
                  }
                  frame True {
                    # "calculate absorption cross sections from HITRAN data base"
                    n450 = local read "Off-Line Smoothed"() -> (w577:dbl[])
                    n451 = local read "Lambda On Read (nm)"() -> (w580:dbl)
                    n452 = local read "Lambda Off Set (nm)"() -> (w583:dbl)
                    n453 = local read "Temperature (C)"() -> (w581:dbl)
                    n454 = local read "Pressure (mb)"() -> (w582:dbl)
                    n455 = script code="%Importing HITRAN data\n%hitran = dlmread('C:\\Users\\H2ODial\\Desktop\\Shared Telescope WV DIAL Code\\Libraries and VIs\\824nm_841nm_H2O.csv', ',',[0 1 352 7]);\nhitran = dlmread('C:\\Users\\H2ODial\\Desktop\\Shared Telescope WV DIAL Code\\Libraries and VIs\\824nm_841nm_H2O_Spectral_Calc.csv', ',',[1 1 1209 7]);\n\n%Range vector in meters\nrange = ([75:75:size(Online,2)*75]);\n\nif lambda< 828\nlambda=828.195;\nelse\nlambda=lambda;\nend;\n\n%%\n\n%Voigt profile calculation\nWNmin = 12070.0;\nWNmax = 12076.0;\n\n%Find lines from WNmin to WNmax to calculate voigt profile\nline_indices = find(hitran(1:size(hitran,1),1)>WNmin & hitran(1:size(hitran,1),1)<WNmax);\n\nline = (hitran(line_indices, 1:size(hitran,2)));\n\n%Calculate temperature and pressure profile\nT0 = 273+15.6;\nT0 = 273+T0_C;\n\nT = T0-0.005545.*range; \n\nP0  = 1.0;\nP0  = P0_mb/1000*0.986; %pressure in mb converted to atm\n\nP = P0.*(T0./T).^-5.21986;\n\n%linewidth temperature dependence factor\nalpha = line(:,7);        \n\n%initial Lorentz linewidth from HiTRAN [cm^-1]\ngammal0 = line(:,4);     \n\n%ground state transition energy [cm^-1]\nE = line(:,6);           \n\n%initial linestrength from HiTRAN [cm^-1/(mol*cm^-2)]\nS0 = line(:,2);      \n\n%absorption line center wavenumber from HiTRAN [cm^-1]\nnu0_0 = line(:,1);    \n\nnu_on = (1/(lambda)*1e7);\n\nnu_off = (1/(lambda_off)*1e7);\n\n\nfor i = 1:size(Online,2);\n\n    %Pressure shift\n    nu0 = nu0_0-.0428.*P(i);\n    \n    %Calculate Lorentz lineweidth at temperature T [cm^-1]\n    gammal = gammal0.*(P(i)./P0).*((T0./T(i)).^alpha);\n    \n    %Calculate Doppler linewidth at temperature T [cm^-1]\n    gammad = (nu0).*((2.0.*1.38E-23.*T(i).*log(2.0))./(0.018.*3.0E8.*3.0E8./6.022E23)).^(0.5);\n    \n    y = (gammal./gammad).*((log(2.0)).^(0.5));\n    \n    x_on = ((nu_on-nu0)./gammad).*(log(2.0)).^(0.5);\n    \n    x_off = ((nu_off-nu0)./gammad).*(log(2.0)).^(0.5);\n    \n    %setting up Voigt convolution\n    stepsize = 1;\n    \n    t = [-200:1:199].*stepsize;\n    \n    t = repmat(t',1,length(x_on))';\n    \n    x_on = repmat(x_on,1,length(t));\n    \n    x_off = repmat(x_off,1,length(t));\n    \n    y = repmat(y,1,length(t));\n    \n    f_on = (exp(-t.^2.0))./(y.^2.0+(x_on-t).^2.0);\n    \n    f_off = (exp(-t.^2.0))./(y.^2.0+(x_off-t).^2.0);\n    \n    %Set the integration sum to zero to start\n    integral_on = 0.0;\n    \n    integral_off = 0.0;\n    \n    %Voigt integration\n    z_on = trapz(t(1,:),f_on,2);\n    \n    z_off =  trapz(t(1,:),f_off,2);\n    \n    integral_on = z_on;\n    \n    integral_off = z_off;\n    \n    %Calculate linestrength at temperature T\n    S = S0.*((T0./T(i)).^(1.5)).*exp(1.439.*E.*((1./T0)-(1./T(i))));\n    \n    %Calculate Doppler line-center cross section [cm^2]\n    K = (S./gammad).*(((log(2.0))./pi).^(0.5));\n    \n    %Calculate the Voigt profile\n    V_on = (y(1)/pi).*integral_on;\n    \n    V_off = (y(1)./pi).*integral_off;\n    \n    %Calculate the Voigt profile absorption cross section [cm^2]\n    sigmav_on = K.*V_on;\n    \n    sigmav_off = K.*V_off;\n    \n    %Sum contributions from all of the surrounding lines\n    sigma_on_total(i) = sum(sigmav_on);\n    \n    sigma_off_total(i) = sum(sigmav_off);\n    \nend;"("lambda"=w580, "lambda_off"=w583, "P0_mb"=w582, "T0_C"=w581, "Online"=w577) -> ("sigma_on_total"=→"sigma_on_total":dbl[], "sigma_off_total"=→"sigma_off_total":dbl[])  [unwired: 1 in, 1 out]
                  }
                }
              }
              frame #5 {
                w594 = 1
                # "normalization factor\nfrom 300 to 450m"
                # "OPTICAL DEPTH PLOT"
                # "new rainbow color bar display"
                # "Data Processing Far Channel"
                # "new rainbow color bar display"
                # "Calculating the range resolved water vapor number density and plotting"
                n456 = local read "sigma_off_total"() -> (w617:dbl[])
                n457 = local read "sigma_on_total"() -> (w614:dbl[])
                n458 = local read "On-Line  Smoothed"() -> (w592:dbl[])
                n459 = local read "Off-Line Smoothed"() -> (w591:dbl[])
                n460 = local read "Off-Line Smoothed 2"() -> (w615:dbl[])
                n461 = local read "On-Line Smoothed 2"() -> (w616:dbl[])
                n462 = script code="%Time averaging in seconds.  600 Seconds =10 minutes\ntemporal_average = 600;\n\n%Spatial averaging in bins.  2 bins = 150 meters\nspatial_average = 2;\n\n%Creating r and r+deltar vectors..this can also be acsomplished using the\n%diff command\np_oni = Online(:,1:size(Online,2)-1);\n\np_onii = Online(:,2:size(Online,2));\n\np_offi = Offline(:,1:size(Offline,2)-1);\n\np_offii = Offline(:,2:size(Offline,2));\n\nInside = (p_oni.*p_offii)./(p_onii.*p_offi);\n\ndel_cross = 1./(2.*(sigma_on_total(1:size(Online,2)-1)-sigma_off_total(1:size(Offline,2)-1)).*75*100);\n\ndel_cross(isinf(del_cross)) = 0;\n\n%Calculating Number density\nN = del_cross.*log(Inside);\n\n%Spatial smoothing of the profiles\nfilter1 = ones(1,2)./2;\n\nN_1 = N;\n\nN_1_avg = filter2(filter1,N_1);\n\nfilter1 = ones(1,10)./10;\n\nN_2 = N;\n\nN_2_avg = filter2(filter1,N_2);\n\nN_new = zeros(size(N,1),size(N,2));\n \n%Using different averaging windows for different altitudes \nN_avg=[N_1_avg(:,1:40)';N_2_avg(:,41:size(N,2))']';\n\n\nw = N_avg.*1e6.*18.015./6.022e23"("Online"=w616, "Offline"=w615, "sigma_on_total"=w614, "sigma_off_total"=w617) -> ("N_avg"=w618:cdb[], "w"=w627:cdb[])  [unwired: 1 in, 1 out]
                n463 = script code="%Time averaging in seconds.  600 Seconds = 10 minutes\ntemporal_average = 600;\n\n%Spatial averaging in bins.  2 bins = 150 meters\nspatial_average = 2;\n\n%Creating r and r+deltar vectors..this can also be acsomplished using the\n%diff command\np_oni = Online(:,1:size(Online,2)-1);\n\np_onii = Online(:,2:size(Online,2));\n\np_offi = Offline(:,1:size(Offline,2)-1);\n\np_offii = Offline(:,2:size(Offline,2));\n\nInside = (p_oni.*p_offii)./(p_onii.*p_offi);\n\ndel_cross = 1./(2.*(sigma_on_total(1:size(Online,2)-1)-sigma_off_total(1:size(Offline,2)-1)).*75*100);\n\ndel_cross(isinf(del_cross)) = 0;\n\n%Calculating Number density\nN = del_cross.*log(Inside);\n\n%Spatial smoothing of the profiles\nfilter1 = ones(1,2)./2;\n\nN_1 = N;\n\nN_1_avg = filter2(filter1,N_1);\n\nfilter1 = ones(1,10)./10;\n\nN_2 = N;\n\nN_2_avg = filter2(filter1,N_2);\n\nN_new = zeros(size(N,1),size(N,2));\n \n%Using different averaging windows for different altitudes \nN_avg=[N_1_avg(:,1:40)';N_2_avg(:,41:size(N,2))']';\n\n \nw = N_avg.*1e6.*18.015./6.022e23"("Online"=w592, "Offline"=w591, "sigma_on_total"=w614, "sigma_off_total"=w617) -> ("N_avg"=w623:cdb[], "w"=w624:cdb[])  [unwired: 1 in, 1 out]
                n464 = local read "Time Resolution Per Bin(ns)"() -> (w593:u32)
                n465 = local read "bins"() -> (w619:u32)
                n466 = local read "Altitude Array (km)"() -> (w589:dbl[])
                n467 = Build Array(w624, w627) -> (w630:cdb[][])
                n468 = To Double Precision Float(number=w593) -> (double precision float=w612:dbl)
                n469 = Reshape Array(w623, w594, w619) -> (w634:cdb[][])
                n470 = Reshape Array(w618, w594, w619) -> (w621:cdb[][])
                n471 = Multiply(x=0.15, y=w612) -> (x*y=w610:dbl)
                n472 = Build Array(w623, w618) -> (w628:cdb[][])
                n473 = Divide(x=300.0, y=w610) -> (x/y=w607:dbl)
                n474 = Divide(x=450.0, y=w610) -> (x/y=w606:dbl)
                n475 = Build Array(w589, w589) -> (w613:dbl[][])
                n476 = call "Convert to Dynamic Data5"("2D Array"=w630) -> ("Dynamic Data Type"=w629:dynamicdata)  [unwired: 3 in]
                n477 = call "Convert to Dynamic Data2"("2D Array"=w628) -> ("Dynamic Data Type"=w625:dynamicdata)  [unwired: 3 in]
                n478 = Divide(x=w634, y=1e+17) -> (x/y=→"Water Vapor Number Density":cdb[][])
                n479 = Divide(x=w621, y=1e+17) -> (x/y=→"Water Vapor Number Density 2":cdb[][])
                n480 = call "Convert to Dynamic Data6"("Array"=w589) -> ("Dynamic Data Type"=w590:dynamicdata)  [unwired: 3 in]
                n481 = To Long Integer(number=w607) -> (32bit integer=w605:i32)
                n482 = To Long Integer(number=w606) -> (32bit integer=w604:i32)
                n483 = call "Convert to Dynamic Data"("2D Array"=w613) -> ("Dynamic Data Type"=w626:dynamicdata)  [unwired: 3 in]
                n484 = call "Convert to Dynamic Data8"("2D Array"=w613) -> ("Dynamic Data Type"=w631:dynamicdata)  [unwired: 3 in]
                n485 = Decrement(x=w605) -> (x-1=w602:i32)
                n486 = Decrement(x=w604) -> (x-1=w603:i32)
                n487 = call "Build XY Graph"("Y Input"=w626, "X Input"=w625) -> ("XY Graph"=→"Water Vapor Number Density  2":cluster{"Y":dbl[], "Y":dbl[]}[])  [unwired: 3 in, 6 out]
                n488 = call "Build XY Graph3"("Y Input"=w631, "X Input"=w629) -> ("XY Graph"=→"Absolute Humidity":cluster{"Y":dbl[], "Y":dbl[]}[])  [unwired: 3 in, 6 out]
                n489 = Array Subset(array=w592, index=w602, length=w603) -> (w601:dbl[])
                n490 = Array Subset(array=w591, index=w602, length=w603) -> (w600:dbl[])
                n491 = call-poly <vilib>:"Mean.vi"("X"=w601) -> ("mean"=w599:dbl)  [unwired: 1 out]
                n492 = call-poly <vilib>:"Mean.vi"("X"=w600) -> ("mean"=w598:dbl)  [unwired: 1 out]
                n493 = Divide(x=w599, y=w598) -> (x/y=w597:dbl)
                n494 = Multiply(x=w591, y=w597) -> (x*y=w596:dbl[])
                n495 = Divide(x=w592, y=w596) -> (x/y=w595:dbl[])
                n496 = Natural Logarithm(1:w595) -> (0:w586:dbl[])
                n497 = Multiply(x=-1.0, y=w586) -> (x*y=w585:dbl[])
                n498 = call "Convert to Dynamic Data9"("Array"=w585) -> ("Dynamic Data Type"=w588:dynamicdata)  [unwired: 3 in]
                n499 = call "Build OD Plot"("Y Input"=w590, "X Input"=w588) -> ("XY Graph"=→"Optical Depth":cluster{"Y":dbl[], "Y":dbl[]}[])  [unwired: 3 in, 6 out]
              }
            }
          }
        }
        "L_Count" <- w132
      }
    }
  }
  n500 = case shown="True" w3 {
    frame False {
    }
    frame True {
      # "close data files"
      n501 = local read "NF_Off_Ref"() -> (w637:refnum<file>)
      n502 = local read "NF_On_Ref"() -> (w638:refnum<file>)
      n503 = local read "FF_Off_Ref"() -> (w639:refnum<file>)
      n504 = local read "FF_On_Ref"() -> (w640:refnum<file>)
      n505 = Close File(refnum=w640) -> ()  [unwired: 1 in, 2 out]
      n506 = Close File(refnum=w639) -> ()  [unwired: 1 in, 2 out]
      n507 = Close File(refnum=w638) -> ()  [unwired: 1 in, 2 out]
      n508 = Close File(refnum=w637) -> ()  [unwired: 1 in, 2 out]
    }
  }
  "FileHour" <- -1 ("FileHour")
  "DataOpen" <- FALSE
